vi "XW angle calib checker_fitmode_PN.vi"(0 "XW_Calib_Map file path (dialog if empty)":path=path "C:/Documents and Settings/Paul Nathan/Desktop/XW Calib Map/XW angle calib checker/XW002_OH74.txt") -> (1 "Quantities that vary with Uref (epsilon, theta, k) (higher order method)":string="Uref (m/s)\teps1 (deg)\teps2 (deg)\tProbe zero err. (deg)\ttheta 1 (deg)\ttheta 2 (deg)\tk1\tk2\r\n0.5018157894736842\t6.6267533355295267\t-2.9096917617315063\t1.8585307868990102\t-71.8440498634698343\t62.9636877172930269\t0.6599332295131558\t0.5182677319056692\r\n0.9994315789473684\t-1.5238812538482893\t0.9867720938009588\t-0.2685545800236653\t-50.7967211983630662\t49.0160971121406419\t0.4477378321660209\t0.4147363151308791\r\n2.0002052631578948\t-0.7133248964583326\t0.8757082064818568\t0.0811916550117621\t-47.4142025982968249\t46.7238739777964795\t0.3482854524979783\t0.3208003585595112\r\n3.0007842105263158\t0.1760631838109209\t0.0773496663189839\t0.1267064250649524\t-46.5210606369966584\t46.4000168794064933\t0.3180701353043149\t0.2880980466431173\r\n3.9999473684210529\t0.1906487887884849\t-0.2531251578949695\t-0.0312381845532423\t-46.1290205114913973\t46.2520699692747499\t0.2973863116337986\t0.2724916341605897\r\n4.9998315789473686\t0.2282387696125690\t-0.2130683224321257\t0.0075852235902217\t-45.8252448288331706\t46.0312176850919527\t0.2848963782809624\t0.2591128097080995\r\n6.9997315789473680\t0.1263159354503521\t-0.1724714828642592\t-0.0230777737069536\t-45.2896437061695636\t45.4966612147379905\t0.2642800771604699\t0.2410224971037088\r\n9.0019315789473691\t-0.0565462004426649\t0.0773785766074275\t0.0104161880823813\t-44.8675096760090710\t45.0959281609883007\t0.2463064031896132\t0.2236365187658775\r\n10.9999736842105253\t-0.2539290822848205\t0.4859354251419727\t0.1160031714285761\t-44.4053231675819475\t44.4986166412718589\t0.2285399354877704\t0.2028480726593352\r\n13.0001684210526314\t-0.5118579225506359\t0.7409038885633608\t0.1145229830063624\t-44.0067920576490863\t43.9637273900855589\t0.2106532081178253\t0.1851715125746720\r\n15.0011421052631579\t-0.7550503383633456\t0.9105592735667931\t0.0777544676017238\t-43.6252625738814430\t43.5843363193315980\t0.1938872474806047\t0.1681952069880479\r\n", 2 "Quantities that vary with Uref (epsilon, theta, k) (standard method)":string="Uref (m/s)\teps1 (deg)\teps2 (deg)\tProbe zero err. (deg)\ttheta 1 (deg)\ttheta 2 (deg)\r\n0.5018157894736842\t9.3017890724801830\t-6.2576200383800815\t1.5220845170500508\t-30.2854646617259924\t38.4907443143961103\r\n0.9994315789473684\t-0.5078267063761874\t0.4756008610831978\t-0.0161129226464948\t-33.2549649340571562\t37.2028076780815198\r\n2.0002052631578948\t-0.0170670287325283\t0.4389133857835795\t0.2109231785255256\t-40.3150704772274295\t40.5384275834816208\r\n3.0007842105263158\t0.5397928552976248\t-0.1673075851488837\t0.1862426350743706\t-41.7471477428440920\t42.7336376551682235\r\n3.9999473684210529\t0.5552032611501811\t-0.4809296208955749\t0.0371368201273031\t-42.3649922651800707\t43.4904856798574783\r\n4.9998315789473686\t0.5839145398374913\t-0.4879117310338565\t0.0480014044018174\t-42.5176867926462378\t43.6855272441884636\r\n6.9997315789473680\t0.4769954292660519\t-0.3766339827294708\t0.0501807232682906\t-42.6403950914849332\t43.8399700483001169\r\n9.0019315789473691\t0.2955464302508806\t-0.1481957767585597\t0.0736753267461604\t-42.6422862340712001\t43.6715341103828791\r\n10.9999736842105253\t0.0708841951620765\t0.2586334095830275\t0.1647588023725520\t-42.4997912977266665\t43.2532991548099801\r\n13.0001684210526314\t-0.2243455550085545\t0.5043620030432825\t0.1400082240173640\t-42.3214463588717393\t42.9148784991085179\r\n15.0011421052631579\t-0.4668513181945785\t0.7171710888419789\t0.1251598853237002\t-42.1380350724668275\t42.7497636859784933\r\n")   [LabVIEW 2011]
uses:
  <vilib>/Utility/file.llb/Read From Spreadsheet File (DBL).vi
  <vilib>/Utility/file.llb/Read From Spreadsheet File (string).vi
  <vilib>/Analysis/polynomials.llb/Polynomial Plot (Range).vi
  <vilib>/Analysis/polynomials.llb/Polynomial Roots (DBL).vi
  <vilib>/Analysis/polynomials.llb/Polynomial Plot (Samples).vi
  <vilib>/Analysis/NI_AALPro.lvlib
  <vilib>/Analysis/NI_AALBase.lvlib
panel:
  out "No real roots for the set (i.e. poor dataset)":bool[](array[boolean])
  in  "Transfer query set control here":bool
  in  "Query set (alias)":i32
  out "Quartic tan(2e) function":cluster{dbl[], dbl[]}[](graph)
  out "Roots for e2 (2nd index angle set -1)":cdb[][](array[numeric])=[[-1.531222514048462+0.0i, -5.778988170526063+0.0i, 16.707412903025652+0.0i, 6.4875967459+0.0i, 5.078758977720174+0.0i, 4.514924906289319+0.0i, 3.854535285382964+0.0i, 3.5396117006623293+0.0i, 3.273353030480773+0.0i, 3.048630181958499+0.0i, 2.870340574754266+0.0i], [0.0160598872047017+0.9915361243519932i, 0.030855825212726732+0.9930589066324856i, 0.0324524213798118+1.0004216780304256i, 0.03210670637546993+1.0043354071771735i, 0.03176644318451339+1.0060241435427542i, 0.0316033433674252+1.0067247444186669i, 0.0320563492832904+1.0079772109676077i, 0.032215191064157794+1.0084528128807428i, 0.032831359734918485+1.0088460213011843i, 0.03354547660184823+1.0094431819546545i, 0.03393148490012644+1.0099991970101192i], [0.0160598872047017-0.9915361243519932i, 0.030855825212726732-0.9930589066324856i, 0.0324524213798118-1.0004216780304256i, 0.03210670637546993-1.0043354071771735i, 0.03176644318451339-1.0060241435427542i, 0.0316033433674252-1.0067247444186669i, 0.0320563492832904-1.0079772109676077i, 0.032215191064157794-1.0084528128807428i, 0.032831359734918485-1.0088460213011843i, 0.03354547660184823-1.0094431819546545i, 0.03393148490012644-1.0099991970101192i], [-0.10191810443911936+0.0i, 0.03445847280570602+0.0i, 0.030577507463478096+0.0i, 0.002700019266282215+0.0i, -0.00883596479286889+0.0i, -0.007437624657217361+0.0i, -0.006020463221166026+0.0i, 0.0027010284330839292+0.0i, 0.01696397323767586+0.0i, 0.025868192292574674+0.0i, 0.03179522253597651+0.0i]]
  out "Roots for e1 (2nd index angle set- 1)":cdb[][](array[numeric])=[[-0.015920835836600963+0.9840410941913055i, 3.395480898493786+0.0i, -594.6858847660856+0.0i, -9.256262608165475+0.0i, -6.488582226964654+0.0i, -5.4418669081945525+0.0i, -4.436840208641847+0.0i, -3.919873244378892+0.0i, -3.5319472433943147+0.0i, -3.2746647104988313+0.0i, -3.0804435614198247+0.0i], [-0.015920835836600963-0.9840410941913055i, -0.02744316398189495+0.9898767262763452i, -0.03214949692082159+0.9987358189508451i, -0.033633194220895994+1.0032718682899568i, -0.0335171638363392+1.0048208292329712i, -0.03365083549489199+1.005877792371468i, -0.03393002543702201+1.007203137493328i, -0.03407557298898485+1.0080087857191544i, -0.034416949826886645+1.0087849149152948i, -0.03463560472159085+1.0092611917473095i, -0.03494277753284671+1.009676498285988i], [0.6282192557965216+0.0i, -0.02744316398189495-0.9898767262763452i, -0.03214949692082159-0.9987358189508451i, -0.033633194220895994-1.0032718682899568i, -0.0335171638363392-1.0048208292329712i, -0.03365083549489199-1.005877792371468i, -0.03393002543702201-1.007203137493328i, -0.03407557298898485-1.0080087857191544i, -0.034416949826886645-1.0087849149152948i, -0.03463560472159085-1.0092611917473095i, -0.03494277753284671-1.009676498285988i], [0.23553334080037738+0.0i, -0.053243718596295814+0.0i, -0.024904883355210836+0.0i, 0.006145841875296154+0.0i, 0.0066549964036471156+0.0i, 0.00796720459081318+0.0i, 0.004409286517190577+0.0i, -0.0019738373178073043+0.0i, -0.008864029245855196+0.0i, -0.017869113637998108+0.0i, -0.026362333333484183+0.0i]]
  in  "Coefficient Constraint":cluster{"order":i32, "coefficient":dbl}[](array[cluster])
  in  "Ignore first n pts from calib.":i32
  out "Higher order effective angle method X plot data (each angle set separated by a column of zeros)":string="x_0\ty1_0\ty2_0\t\tx_1\ty1_1\ty2_1\t\tx_2\ty1_2\ty2_2\t\tx_3\ty1_3\ty2_3\t\tx_4\ty1_4\ty2_4\t\tx_5\ty1_5\ty2_5\t\tx_6\ty1_6\ty2_6\t\tx_7\ty1_7\ty2_7\t\tx_8\ty1_8\ty2_8\t\tx_9\ty1_9\ty2_9\t\tx_10\ty1_10\ty2_10\r\n-0.9999999999999999\t-0.9085791502544248\t-3.9630468181290452\t0.0000000000000000\t-0.9999999999999999\t0.1949143754370715\t-2.6536651485735696\t0.0000000000000000\t-0.9999999999999999\t0.5188418104065096\t-2.7107465604685741\t0.0000000000000000\t-0.9999999999999999\t0.6105115215521106\t-2.7972176259688553\t0.0000000000000000\t-0.9999999999999999\t0.6514204222508733\t-2.8375050105836368\t0.0000000000000000\t-0.9999999999999999\t0.6746558655695405\t-2.8404947938821206\t0.0000000000000000\t-0.9999999999999999\t0.7084619405900626\t-2.8035914112508933\t0.0000000000000000\t-0.9999999999999999\t0.7363342408659557\t-2.7810177224561561\t0.0000000000000000\t-0.9999999999999999\t0.7620888951136892\t-2.7288520875385447\t0.0000000000000000\t-0.9999999999999999\t0.7861588927941786\t-2.6856742001602751\t0.0000000000000000\t-0.9999999999999999\t0.8056811585366324\t-2.6550478856042679\t0.0000000000000000\r\n-0.8459634362504808\t-0.4625621144061756\t-2.8818271450789865\t0.0000000000000000\t-0.8459634362504808\t0.2815754544138509\t-2.1394999422469003\t0.0000000000000000\t-0.8459634362504808\t0.5527709767869218\t-2.2324745574527904\t0.0000000000000000\t-0.8459634362504808\t0.6382823976284421\t-2.2665818845631214\t0.0000000000000000\t-0.8459634362504808\t0.6788684735006610\t-2.2842367882197863\t0.0000000000000000\t-0.8459634362504808\t0.7029454921629841\t-2.2878897351586707\t0.0000000000000000\t-0.8459634362504808\t0.7360252511014151\t-2.2626966309367886\t0.0000000000000000\t-0.8459634362504808\t0.7617351722175852\t-2.2416920469763459\t0.0000000000000000\t-0.8432720672116305\t0.7844643868612465\t-2.1887614629441035\t0.0000000000000000\t-0.8432720672116305\t0.8038053956321515\t-2.1508294307461551\t0.0000000000000000\t-0.8432720672116305\t0.8196056618936665\t-2.1284563267855230\t0.0000000000000000\r\n-0.7028117712403573\t-0.0667229984385117\t-1.7990557676966663\t0.0000000000000000\t-0.7028117712403573\t0.3411211378733948\t-1.6837865113002857\t0.0000000000000000\t-0.7028117712403573\t0.5825100736406964\t-1.6930687846557417\t0.0000000000000000\t-0.7028117712403573\t0.6448979960495834\t-1.7825502259833412\t0.0000000000000000\t-0.7028117712403573\t0.6810359033183786\t-1.8105052193118192\t0.0000000000000000\t-0.7028117712403573\t0.7040869499204692\t-1.8110590099219335\t0.0000000000000000\t-0.7028117712403573\t0.7342043939074193\t-1.7929291162742504\t0.0000000000000000\t-0.7028117712403573\t0.7550109725157748\t-1.7756905349598751\t0.0000000000000000\t-0.7028117712403573\t0.7711095218508195\t-1.7384235052178580\t0.0000000000000000\t-0.7028117712403573\t0.7847492951756501\t-1.7045648544699419\t0.0000000000000000\t-0.7028117712403573\t0.7958199433613861\t-1.6859867806778905\t0.0000000000000000\r\n-0.5745611109571804\t-0.0376287976903837\t-1.5446740531776548\t0.0000000000000000\t-0.5745611109571804\t0.3599220910286302\t-1.3459064192482468\t0.0000000000000000\t-0.5745611109571804\t0.5655852803690335\t-1.3559695335879334\t0.0000000000000000\t-0.5745611109571804\t0.6247863747603235\t-1.3916622950809854\t0.0000000000000000\t-0.5745611109571804\t0.6553574621762963\t-1.4097043857813083\t0.0000000000000000\t-0.5745611109571804\t0.6735069299277736\t-1.4112094707533349\t0.0000000000000000\t-0.5745611109571804\t0.6949413208702192\t-1.4067266943759922\t0.0000000000000000\t-0.5745611109571804\t0.7105513693367174\t-1.3847598236387422\t0.0000000000000000\t-0.5745611109571804\t0.7218957685787146\t-1.3544132560361197\t0.0000000000000000\t-0.5766523484064272\t0.7309919560241551\t-1.3305928734680903\t0.0000000000000000\t-0.5745611109571804\t0.7384817158571489\t-1.3099108075871668\t0.0000000000000000\r\n-0.4610063144273182\t0.0412919475631363\t-1.0997890950007321\t0.0000000000000000\t-0.4610063144273182\t0.3770239497989202\t-0.9792680032688384\t0.0000000000000000\t-0.4610063144273182\t0.5367013693167687\t-1.0119826258435312\t0.0000000000000000\t-0.4610063144273182\t0.5743830527285835\t-1.0774202158722981\t0.0000000000000000\t-0.4610063144273182\t0.5979952814046342\t-1.0939710197186976\t0.0000000000000000\t-0.4667326950738877\t0.6116296380054032\t-1.0948501153158237\t0.0000000000000000\t-0.4610063144273182\t0.6279311798252735\t-1.0827733496154128\t0.0000000000000000\t-0.4610063144273182\t0.6377056286721594\t-1.0683619324969325\t0.0000000000000000\t-0.4610063144273182\t0.6452821120555695\t-1.0398621565011508\t0.0000000000000000\t-0.4629123289077153\t0.6520868780188794\t-1.0198362226727229\t0.0000000000000000\t-0.4629123289077153\t0.6571442461528323\t-1.0051143364341999\t0.0000000000000000\r\n-0.3689194771098271\t0.1044333744574640\t-0.7437632758411701\t0.0000000000000000\t-0.3689194771098271\t0.3703284183929321\t-0.7061988569542564\t0.0000000000000000\t-0.3689194771098271\t0.4814947359213608\t-0.7770192864712264\t0.0000000000000000\t-0.3689194771098271\t0.5088608177696153\t-0.8210529776089235\t0.0000000000000000\t-0.3635749763519443\t0.5263421036228286\t-0.8282138902172458\t0.0000000000000000\t-0.3689194771098271\t0.5331564790478260\t-0.8458290235908140\t0.0000000000000000\t-0.3689194771098271\t0.5437170073266897\t-0.8393399765706897\t0.0000000000000000\t-0.3689194771098271\t0.5501602814743358\t-0.8249109991926368\t0.0000000000000000\t-0.3689194771098271\t0.5563221043460842\t-0.7999971908211336\t0.0000000000000000\t-0.3689194771098271\t0.5623927525763176\t-0.7803547186651004\t0.0000000000000000\t-0.3689194771098271\t0.5671583051208874\t-0.7700855374663110\t0.0000000000000000\r\n-0.2718814121476857\t0.0255847727338301\t-0.6689751955611348\t0.0000000000000000\t-0.2718814121476857\t0.3106644522796246\t-0.5047454592362141\t0.0000000000000000\t-0.2718814121476857\t0.3962036651655259\t-0.5446172063124690\t0.0000000000000000\t-0.2718814121476857\t0.4082234758439587\t-0.5916721671054449\t0.0000000000000000\t-0.2718814121476857\t0.4191107855801626\t-0.5983889263646065\t0.0000000000000000\t-0.2718814121476857\t0.4242807676181213\t-0.6036578351430176\t0.0000000000000000\t-0.2718814121476857\t0.4289132363159743\t-0.6011772566633612\t0.0000000000000000\t-0.2718814121476857\t0.4344930216745795\t-0.5885638990500427\t0.0000000000000000\t-0.2718814121476857\t0.4407940406478280\t-0.5667386082032163\t0.0000000000000000\t-0.2718814121476857\t0.4466625036118104\t-0.5511317529698531\t0.0000000000000000\t-0.2718814121476857\t0.4513779468028263\t-0.5395864188016505\t0.0000000000000000\r\n-0.1761470268806888\t-0.0942490676366393\t-0.5868960272983509\t0.0000000000000000\t-0.1761470268806888\t0.2548185009347063\t-0.2645492620955306\t0.0000000000000000\t-0.1761470268806888\t0.3024751991218511\t-0.2921952683619167\t0.0000000000000000\t-0.1761470268806888\t0.2870434875402270\t-0.3500127136267793\t0.0000000000000000\t-0.1761470268806888\t0.2830095550319655\t-0.3828463334548899\t0.0000000000000000\t-0.1761470268806888\t0.2855455723517732\t-0.3809026465127626\t0.0000000000000000\t-0.1761470268806888\t0.2884644985637423\t-0.3799013981302747\t0.0000000000000000\t-0.1761470268806888\t0.2930495918311506\t-0.3699160983941475\t0.0000000000000000\t-0.1761470268806888\t0.2992247712103860\t-0.3541806551714389\t0.0000000000000000\t-0.1761470268806888\t0.3058374237252131\t-0.3408777024657876\t0.0000000000000000\t-0.1761470268806888\t0.3111246627753121\t-0.3320591164269514\t0.0000000000000000\r\n-0.0850270210113130\t-0.0504595050252811\t-0.2775995341357290\t0.0000000000000000\t-0.0850270210113130\t0.1736177181817981\t-0.0758426654882593\t0.0000000000000000\t-0.0850270210113130\t0.1727751104131255\t-0.1124460755508965\t0.0000000000000000\t-0.0850270210113130\t0.1397558723489909\t-0.1611761582181669\t0.0000000000000000\t-0.0850270210113130\t0.1364092384545839\t-0.1803971782800010\t0.0000000000000000\t-0.0850270210113130\t0.1330151029088564\t-0.1846382073328683\t0.0000000000000000\t-0.0850270210113130\t0.1336180079889946\t-0.1859543864792222\t0.0000000000000000\t-0.0850270210113130\t0.1391330147914122\t-0.1779026144672113\t0.0000000000000000\t-0.0881921819968595\t0.1468097530657032\t-0.1664128928822258\t0.0000000000000000\t-0.0850270210113130\t0.1533034947310865\t-0.1537657502004380\t0.0000000000000000\t-0.0850270210113130\t0.1602920927213465\t-0.1466312867329973\t0.0000000000000000\r\n0.0000000000000000\t-0.1396755488429087\t-0.1495552894031837\t0.0000000000000000\t0.0000000000000000\t0.1015398030851381\t0.0979907823209607\t0.0000000000000000\t0.0000000000000000\t0.0485713499475330\t0.0551796899852733\t0.0000000000000000\t0.0000000000000000\t0.0039204586603697\t0.0100793521533393\t0.0000000000000000\t0.0000000000000000\t-0.0123772694902811\t-0.0123048930616856\t0.0000000000000000\t0.0000000000000000\t-0.0158825708767742\t-0.0172400662126269\t0.0000000000000000\t0.0000000000000000\t-0.0185621834928470\t-0.0203971278636718\t0.0000000000000000\t0.0000000000000000\t-0.0117122957217886\t-0.0145134805930901\t0.0000000000000000\t-0.0015707976187244\t-0.0034205951378717\t-0.0026021495757281\t0.0000000000000000\t0.0000000000000000\t0.0051491403774043\t0.0063664317326143\t0.0000000000000000\t0.0000000000000000\t0.0119067452638700\t0.0115332438693104\t0.0000000000000000\r\n0.0834450784477064\t-0.0417648215636864\t0.1352429486294378\t0.0000000000000000\t0.0834450784477064\t-0.0776394529995262\t0.1668355133205353\t0.0000000000000000\t0.0834450784477064\t-0.1147770314630093\t0.1823015191280195\t0.0000000000000000\t0.0834450784477064\t-0.1518089738821856\t0.1616926063828080\t0.0000000000000000\t0.0834450784477064\t-0.1675177345562901\t0.1418323488914914\t0.0000000000000000\t0.0834450784477064\t-0.1743808906051748\t0.1396223268122237\t0.0000000000000000\t0.0834450784477064\t-0.1748799907332232\t0.1407817659046222\t0.0000000000000000\t0.0834450784477064\t-0.1711359562908112\t0.1443459528715696\t0.0000000000000000\t0.0834450784477064\t-0.1631451101745820\t0.1538692306045876\t0.0000000000000000\t0.0834450784477064\t-0.1562961885310737\t0.1594290597441742\t0.0000000000000000\t0.0834450784477064\t-0.1463689695846851\t0.1660732505077365\t0.0000000000000000\r\n0.1745279388943651\t-0.2504441955126037\t0.1552207836757285\t0.0000000000000000\t0.1745279388943651\t-0.1923048605897919\t0.3015431454828965\t0.0000000000000000\t0.1745279388943651\t-0.3118645832700102\t0.3060446247312193\t0.0000000000000000\t0.1745279388943651\t-0.3399045763763606\t0.3042221403451356\t0.0000000000000000\t0.1745279388943651\t-0.3591535093836093\t0.2969861016671120\t0.0000000000000000\t0.1745279388943651\t-0.3625352124879301\t0.2987758625039919\t0.0000000000000000\t0.1745279388943651\t-0.3625811847622155\t0.2987619180587648\t0.0000000000000000\t0.1761470268806888\t-0.3586700905175086\t0.3043173930134577\t0.0000000000000000\t0.1745279388943651\t-0.3487858594270737\t0.3125226906016907\t0.0000000000000000\t0.1745279388943651\t-0.3381938626612139\t0.3167839456066439\t0.0000000000000000\t0.1745279388943651\t-0.3288971373969858\t0.3213424951515983\t0.0000000000000000\r\n0.2701952220731489\t-0.4823610385730527\t0.1684170210190646\t0.0000000000000000\t0.2701952220731489\t-0.3941480974967655\t0.3747405534620119\t0.0000000000000000\t0.2685104627037557\t-0.5123196133813664\t0.4244954643928500\t0.0000000000000000\t0.2685104627037557\t-0.5622716481313378\t0.4320516895393265\t0.0000000000000000\t0.2685104627037557\t-0.5746725215951116\t0.4333475328171350\t0.0000000000000000\t0.2701952220731489\t-0.5761161656795665\t0.4382762721402697\t0.0000000000000000\t0.2701952220731489\t-0.5711564795303717\t0.4462115429854009\t0.0000000000000000\t0.2685104627037557\t-0.5637027508394487\t0.4500064910221563\t0.0000000000000000\t0.2685104627037557\t-0.5531821206069903\t0.4562858049551752\t0.0000000000000000\t0.2685104627037557\t-0.5410697161194152\t0.4598006047578997\t0.0000000000000000\t0.2685104627037557\t-0.5305871950835828\t0.4640535298803268\t0.0000000000000000\r\n0.3635749763519443\t-0.6862363241063577\t0.1938745671240703\t0.0000000000000000\t0.3671359250169842\t-0.6594497435504401\t0.4155995678888906\t0.0000000000000000\t0.3689194771098271\t-0.8062252804138840\t0.4942666230060676\t0.0000000000000000\t0.3671359250169842\t-0.8150435379645339\t0.5333980586374278\t0.0000000000000000\t0.3671359250169842\t-0.8025341705196405\t0.5488805679771741\t0.0000000000000000\t0.3689194771098271\t-0.8130451171136217\t0.5564687631683539\t0.0000000000000000\t0.3671359250169842\t-0.8041120781889549\t0.5656961795372176\t0.0000000000000000\t0.3671359250169842\t-0.7982752853845158\t0.5727446882583248\t0.0000000000000000\t0.3671359250169842\t-0.7840331881102651\t0.5783268868158106\t0.0000000000000000\t0.3671359250169842\t-0.7703712073294504\t0.5816443488942544\t0.0000000000000000\t0.3671359250169842\t-0.7586054072639649\t0.5859279656615510\t0.0000000000000000\r\n0.4629123289077153\t-0.8476294329786266\t0.2235614092068809\t0.0000000000000000\t0.4629123289077153\t-0.9492224197361369\t0.4327728553093401\t0.0000000000000000\t0.4610063144273182\t-0.9819378661710078\t0.5718021480660419\t0.0000000000000000\t0.4610063144273182\t-1.0553848834240576\t0.6055334918430288\t0.0000000000000000\t0.4610063144273182\t-1.0574404797332702\t0.6253666996480907\t0.0000000000000000\t0.4610063144273182\t-1.0556690478955482\t0.6393228823720644\t0.0000000000000000\t0.4610063144273182\t-1.0477195054982680\t0.6529818956214503\t0.0000000000000000\t0.4610063144273182\t-1.0344062288018556\t0.6626927832176096\t0.0000000000000000\t0.4610063144273182\t-1.0205105865152524\t0.6697752152893657\t0.0000000000000000\t0.4610063144273182\t-1.0056840847353361\t0.6738862961883090\t0.0000000000000000\t0.4667326950738877\t-0.9992094770597746\t0.6782936840236679\t0.0000000000000000\r\n0.5724736448682121\t-1.3899789264513560\t0.1020641173846400\t0.0000000000000000\t0.5724736448682121\t-1.2323317956367625\t0.4538004753460074\t0.0000000000000000\t0.5724736448682121\t-1.3238555928281337\t0.6021700169460663\t0.0000000000000000\t0.5724736448682121\t-1.3635980664653848\t0.6589555940191650\t0.0000000000000000\t0.5724736448682121\t-1.3598145734442184\t0.6847037690811968\t0.0000000000000000\t0.5724736448682121\t-1.3684754908238803\t0.7014719043851134\t0.0000000000000000\t0.5724736448682121\t-1.3561242322873066\t0.7226084437915833\t0.0000000000000000\t0.5724736448682121\t-1.3414409891263650\t0.7365615404721209\t0.0000000000000000\t0.5703899296732948\t-1.3202033688759527\t0.7473204528114626\t0.0000000000000000\t0.5703899296732948\t-1.3047561674071091\t0.7540053749349491\t0.0000000000000000\t0.5703899296732948\t-1.2856457129099557\t0.7602089334598410\t0.0000000000000000\r\n0.7004676747806673\t-2.2697364417842891\t-0.1308275547072091\t0.0000000000000000\t0.7004676747806673\t-1.6322660285466430\t0.4389604957859697\t0.0000000000000000\t0.7004676747806673\t-1.7125591635376343\t0.6186366367406101\t0.0000000000000000\t0.7004676747806673\t-1.7507849758841230\t0.6833036449657283\t0.0000000000000000\t0.7004676747806673\t-1.7532033361976842\t0.7149717797808454\t0.0000000000000000\t0.7004676747806673\t-1.7468810658722469\t0.7363863563633494\t0.0000000000000000\t0.6981287310371237\t-1.7323516588972048\t0.7628805858487009\t0.0000000000000000\t0.7004676747806673\t-1.7225575014273988\t0.7821105315579404\t0.0000000000000000\t0.6981287310371237\t-1.6962155420747351\t0.7969917434866054\t0.0000000000000000\t0.6981287310371237\t-1.6783350413415989\t0.8084591863151523\t0.0000000000000000\t0.6981287310371237\t-1.6580717599172035\t0.8184445444178572\t0.0000000000000000\r\n0.8432720672116305\t-2.2413583286537802\t-0.0361829804629510\t0.0000000000000000\t0.8432720672116305\t-2.3075415725227733\t0.3599602272717538\t0.0000000000000000\t0.8432720672116305\t-2.1691060617855422\t0.6115535237817370\t0.0000000000000000\t0.8432720672116305\t-2.2290412862152995\t0.6830463271258672\t0.0000000000000000\t0.8432720672116305\t-2.2222009266918268\t0.7182124425293464\t0.0000000000000000\t0.8379106495048978\t-2.2019648631264235\t0.7421134752332942\t0.0000000000000000\t0.8432720672116305\t-2.1971863462195551\t0.7681137807799585\t0.0000000000000000\t0.8432720672116305\t-2.1821977941933697\t0.7910287339996136\t0.0000000000000000\t0.8432720672116305\t-2.1597258190303488\t0.8104743841359477\t0.0000000000000000\t0.8432720672116305\t-2.1347740356153819\t0.8264250196496778\t0.0000000000000000\t0.8432720672116305\t-2.1122974634158354\t0.8411438740059636\t0.0000000000000000\r\n0.9999999999999999\t-2.8237734406173329\t-0.1791722171870904\t0.0000000000000000\t0.9999999999999999\t-2.6217506945340499\t0.3404580267525550\t0.0000000000000000\t0.9999999999999999\t-2.7652216719375038\t0.5776183997010226\t0.0000000000000000\t0.9999999999999999\t-2.7434622913910154\t0.6673214592086288\t0.0000000000000000\t0.9999999999999999\t-2.7691832771154199\t0.7016501297022305\t0.0000000000000000\t0.9999999999999999\t-2.7634005636598853\t0.7220453961815417\t0.0000000000000000\t0.9999999999999999\t-2.7441674751271026\t0.7453072103707526\t0.0000000000000000\t0.9999999999999999\t-2.7255665231484856\t0.7665049857410070\t0.0000000000000000\t0.9999999999999999\t-2.6957943045968502\t0.7883146132106904\t0.0000000000000000\t0.9999999999999999\t-2.6708083003892944\t0.8079886891481993\t0.0000000000000000\t0.9999999999999999\t-2.6439319990345118\t0.8268920789495620\t0.0000000000000000\r\n"
  out "Standard effective angle method X plot data (each angle set separated by a column of zeros)":string="x_0\ty1_0\ty2_0\t\tx_1\ty1_1\ty2_1\t\tx_2\ty1_2\ty2_2\t\tx_3\ty1_3\ty2_3\t\tx_4\ty1_4\ty2_4\t\tx_5\ty1_5\ty2_5\t\tx_6\ty1_6\ty2_6\t\tx_7\ty1_7\ty2_7\t\tx_8\ty1_8\ty2_8\t\tx_9\ty1_9\ty2_9\t\tx_10\ty1_10\ty2_10\r\n-0.9999999999999999\t-0.3815133550763904\t-1.2277896709808682\t0.0000000000000000\t-0.9999999999999999\t0.1027343623190909\t-0.9114562899981703\t0.0000000000000000\t-0.9999999999999999\t0.3063443292284778\t-0.9263298161188739\t0.0000000000000000\t-0.9999999999999999\t0.3759098795463195\t-0.9486450743962725\t0.0000000000000000\t-0.9999999999999999\t0.4095937180643089\t-0.9589550813083074\t0.0000000000000000\t-0.9999999999999999\t0.4296105414451811\t-0.9597180393827375\t0.0000000000000000\t-0.9999999999999999\t0.4600573554441755\t-0.9502798289606784\t0.0000000000000000\t-0.9999999999999999\t0.4865160575694266\t-0.9444839218816277\t0.0000000000000000\t-0.9999999999999999\t0.5122386804119141\t-0.9310235854433639\t0.0000000000000000\t-0.9999999999999999\t0.5375704300049343\t-0.9198109803207908\t0.0000000000000000\t-0.9999999999999999\t0.5591838915563910\t-0.9118179530499936\t0.0000000000000000\r\n-0.8459634362504808\t-0.2093643431183902\t-0.9702353019573543\t0.0000000000000000\t-0.8459634362504808\t0.1524007163841222\t-0.7718634095908468\t0.0000000000000000\t-0.8459634362504808\t0.3312481602170517\t-0.7979083840543126\t0.0000000000000000\t-0.8459634362504808\t0.3985703678969933\t-0.8073687738154385\t0.0000000000000000\t-0.8459634362504808\t0.4333153200417899\t-0.8122463376207405\t0.0000000000000000\t-0.8459634362504808\t0.4549729292622101\t-0.8132539080775948\t0.0000000000000000\t-0.8459634362504808\t0.4862152698857382\t-0.8062936170337284\t0.0000000000000000\t-0.8459634362504808\t0.5118762167416807\t-0.8004699517004846\t0.0000000000000000\t-0.8432720672116305\t0.5357418679885581\t-0.7857103524771601\t0.0000000000000000\t-0.8432720672116305\t0.5570613988735588\t-0.7750575851915775\t0.0000000000000000\t-0.8432720672116305\t0.5752714536243961\t-0.7687442796474347\t0.0000000000000000\r\n-0.7028117712403573\t-0.0328228301303722\t-0.6730378859119317\t0.0000000000000000\t-0.7028117712403573\t0.1882864654777492\t-0.6382266361222080\t0.0000000000000000\t-0.7028117712403573\t0.3538653960982250\t-0.6410572155338587\t0.0000000000000000\t-0.7028117712403573\t0.4040956419437625\t-0.6680977866969731\t0.0000000000000000\t-0.7028117712403573\t0.4352309350879587\t-0.6764561489379372\t0.0000000000000000\t-0.7028117712403573\t0.4560210940858728\t-0.6766213078456130\t0.0000000000000000\t-0.7028117712403573\t0.4844463111444350\t-0.6712058868596205\t0.0000000000000000\t-0.7028117712403573\t0.5050363372082499\t-0.6660403761493522\t0.0000000000000000\t-0.7028117712403573\t0.5215750025874688\t-0.6548182695443805\t0.0000000000000000\t-0.7028117712403573\t0.5360488120239911\t-0.6445561268834644\t0.0000000000000000\t-0.7028117712403573\t0.5481371262887226\t-0.6388980385240232\t0.0000000000000000\r\n-0.5745611109571804\t-0.0186406617106857\t-0.5952034519702041\t0.0000000000000000\t-0.5745611109571804\t0.1999513083746903\t-0.5316352108933271\t0.0000000000000000\t-0.5745611109571804\t0.3408985513360128\t-0.5349167839293223\t0.0000000000000000\t-0.5745611109571804\t0.3874531648602888\t-0.5465000145751649\t0.0000000000000000\t-0.5745611109571804\t0.4129373646503266\t-0.5523222557772299\t0.0000000000000000\t-0.5745611109571804\t0.4286042789167682\t-0.5528069650646648\t0.0000000000000000\t-0.5745611109571804\t0.4476788261076887\t-0.5513628506497092\t0.0000000000000000\t-0.5745611109571804\t0.4619956964268012\t-0.5442667592222343\t0.0000000000000000\t-0.5745611109571804\t0.4726441131254100\t-0.5344097418995096\t0.0000000000000000\t-0.5766523484064272\t0.4813401461691441\t-0.5266279420566395\t0.0000000000000000\t-0.5745611109571804\t0.4886114157092954\t-0.5198390729242247\t0.0000000000000000\r\n-0.4610063144273182\t0.0208636190821711\t-0.4490649036536395\t0.0000000000000000\t-0.4610063144273182\t0.2107116811955977\t-0.4068646001903803\t0.0000000000000000\t-0.4610063144273182\t0.3193395628632208\t-0.4184437337601838\t0.0000000000000000\t-0.4610063144273182\t0.3476067541187934\t-0.4413258534669730\t0.0000000000000000\t-0.4610063144273182\t0.3659615795589626\t-0.4470559836159407\t0.0000000000000000\t-0.4667326950738877\t0.3768063206397253\t-0.4473597048819011\t0.0000000000000000\t-0.4610063144273182\t0.3900255577692402\t-0.4431816758867931\t0.0000000000000000\t-0.4610063144273182\t0.3980910606014888\t-0.4381800765192558\t0.0000000000000000\t-0.4610063144273182\t0.4044180258399097\t-0.4282374300168551\t0.0000000000000000\t-0.4629123289077153\t0.4101583924636033\t-0.4212094225246056\t0.0000000000000000\t-0.4629123289077153\t0.4144611423251504\t-0.4160205988735473\t0.0000000000000000\r\n-0.3689194771098271\t0.0536561800579369\t-0.3205162913955928\t0.0000000000000000\t-0.3689194771098271\t0.2064815177911305\t-0.3062154711050765\t0.0000000000000000\t-0.3689194771098271\t0.2799269036558585\t-0.3330488687483389\t0.0000000000000000\t-0.3689194771098271\t0.2991867707938265\t-0.3494639593590201\t0.0000000000000000\t-0.3635749763519443\t0.3117719154399675\t-0.3521145995133866\t0.0000000000000000\t-0.3689194771098271\t0.3167405171150758\t-0.3586129042485994\t0.0000000000000000\t-0.3689194771098271\t0.3245127738637020\t-0.3562226869399766\t0.0000000000000000\t-0.3689194771098271\t0.3292990841472899\t-0.3508926675323383\t0.0000000000000000\t-0.3689194771098271\t0.3339084930327397\t-0.3416397395803143\t0.0000000000000000\t-0.3689194771098271\t0.3384811057696974\t-0.3342993362304802\t0.0000000000000000\t-0.3689194771098271\t0.3420929435861684\t-0.3304456161250302\t0.0000000000000000\r\n-0.2718814121476857\t0.0128752726903403\t-0.2918882287416100\t0.0000000000000000\t-0.2718814121476857\t0.1697376633133504\t-0.2266806671812408\t0.0000000000000000\t-0.2718814121476857\t0.2229566711987844\t-0.2428262977232454\t0.0000000000000000\t-0.2718814121476857\t0.2307298756899231\t-0.2616149044401169\t0.0000000000000000\t-0.2718814121476857\t0.2378391151339257\t-0.2642740709057536\t0.0000000000000000\t-0.2718814121476857\t0.2412383560156202\t-0.2663561249281411\t0.0000000000000000\t-0.2718814121476857\t0.2442971723726146\t-0.2653763300549608\t0.0000000000000000\t-0.2718814121476857\t0.2479980197330459\t-0.2603824415827295\t0.0000000000000000\t-0.2718814121476857\t0.2521992515701980\t-0.2516942950270311\t0.0000000000000000\t-0.2718814121476857\t0.2561334149269846\t-0.2454443997906341\t0.0000000000000000\t-0.2718814121476857\t0.2593097454420143\t-0.2408007167960739\t0.0000000000000000\r\n-0.1761470268806888\t-0.0460636059230048\t-0.2597206147786703\t0.0000000000000000\t-0.1761470268806888\t0.1367610417356654\t-0.1245217926281068\t0.0000000000000000\t-0.1761470268806888\t0.1648204978101121\t-0.1367476713685922\t0.0000000000000000\t-0.1761470268806888\t0.1556324778511593\t-0.1619004749232093\t0.0000000000000000\t-0.1761470268806888\t0.1532471169414098\t-0.1759448683738918\t0.0000000000000000\t-0.1761470268806888\t0.1547459389933540\t-0.1751181415129130\t0.0000000000000000\t-0.1761470268806888\t0.1564743623124086\t-0.1746920439546165\t0.0000000000000000\t-0.1761470268806888\t0.1591965698399837\t-0.1704341495334744\t0.0000000000000000\t-0.1761470268806888\t0.1628768138501873\t-0.1636926807243563\t0.0000000000000000\t-0.1761470268806888\t0.1668358047330725\t-0.1579627379435780\t0.0000000000000000\t-0.1761470268806888\t0.1700148572265357\t-0.1541486543885721\t0.0000000000000000\r\n-0.0850270210113130\t-0.0249192675646609\t-0.1303094859974098\t0.0000000000000000\t-0.0850270210113130\t0.0909442911360152\t-0.0372283574450995\t0.0000000000000000\t-0.0850270210113130\t0.0904809569960206\t-0.0547255925362277\t0.0000000000000000\t-0.0850270210113130\t0.0725065349820468\t-0.0775788408363293\t0.0000000000000000\t-0.0850270210113130\t0.0707041582222505\t-0.0864608498606846\t0.0000000000000000\t-0.0850270210113130\t0.0688797622803253\t-0.0884108632923820\t0.0000000000000000\t-0.0850270210113130\t0.0692035711225545\t-0.0890153288541087\t0.0000000000000000\t-0.0850270210113130\t0.0721708211052060\t-0.0853122198092176\t0.0000000000000000\t-0.0881921819968595\t0.0763170203287837\t-0.0800059689104619\t0.0000000000000000\t-0.0850270210113130\t0.0798388699423815\t-0.0741348845468330\t0.0000000000000000\t-0.0850270210113130\t0.0836442245073950\t-0.0708087068813914\t0.0000000000000000\r\n0.0000000000000000\t-0.0675558762158115\t-0.0721731620420199\t0.0000000000000000\t0.0000000000000000\t0.0521285968471978\t0.0502583416112362\t0.0000000000000000\t0.0000000000000000\t0.0245879588335671\t0.0279813221883405\t0.0000000000000000\t0.0000000000000000\t0.0019621543550413\t0.0050524396498774\t0.0000000000000000\t0.0000000000000000\t-0.0061696027461181\t-0.0061336357868599\t0.0000000000000000\t0.0000000000000000\t-0.0079100013774912\t-0.0085831974669353\t0.0000000000000000\t0.0000000000000000\t-0.0092384175668538\t-0.0101470822923124\t0.0000000000000000\t0.0000000000000000\t-0.0058391003146520\t-0.0072305995118944\t0.0000000000000000\t-0.0015707976187244\t-0.0017088375061246\t-0.0013002294895013\t0.0000000000000000\t0.0000000000000000\t0.0025778929547452\t0.0031882984899375\t0.0000000000000000\t0.0000000000000000\t0.0059712002481367\t0.0057833454771090\t0.0000000000000000\r\n0.0834450784477064\t-0.0206688109096341\t0.0700768572776769\t0.0000000000000000\t0.0834450784477064\t-0.0380941445743377\t0.0872215566308192\t0.0000000000000000\t0.0834450784477064\t-0.0558300201561846\t0.0957331804870974\t0.0000000000000000\t0.0834450784477064\t-0.0732236364720010\t0.0844087191234334\t0.0000000000000000\t0.0834450784477064\t-0.0805173457914918\t0.0736266135577358\t0.0000000000000000\t0.0834450784477064\t-0.0836885579377382\t0.0724345450655375\t0.0000000000000000\t0.0834450784477064\t-0.0839188118734830\t0.0730597462104811\t0.0000000000000000\t0.0834450784477064\t-0.0821903512279210\t0.0749842989827523\t0.0000000000000000\t0.0834450784477064\t-0.0784920538300603\t0.0801463326183820\t0.0000000000000000\t0.0834450784477064\t-0.0753121353965432\t0.0831734404720674\t0.0000000000000000\t0.0834450784477064\t-0.0706862143432525\t0.0868041012508523\t0.0000000000000000\r\n0.1745279388943651\t-0.1182326213774142\t0.0808812827908076\t0.0000000000000000\t0.1745279388943651\t-0.0919271315384520\t0.1642626880908670\t0.0000000000000000\t0.1745279388943651\t-0.1453665715699975\t0.1669601598550158\t0.0000000000000000\t0.1745279388943651\t-0.1575424728174603\t0.1658670012193113\t0.0000000000000000\t0.1745279388943651\t-0.1658273926201979\t0.1615407592894643\t0.0000000000000000\t0.1745279388943651\t-0.1672768362680423\t0.1626087309411399\t0.0000000000000000\t0.1745279388943651\t-0.1672965282061860\t0.1626004048596422\t0.0000000000000000\t0.1761470268806888\t-0.1656200455197691\t0.1659240999845745\t0.0000000000000000\t0.1745279388943651\t-0.1613724034206572\t0.1708574854717018\t0.0000000000000000\t0.1745279388943651\t-0.1568032947140209\t0.1734311556843217\t0.0000000000000000\t0.1745279388943651\t-0.1527780087237028\t0.1761932842903005\t0.0000000000000000\r\n0.2701952220731489\t-0.2175225002327688\t0.0880882833404676\t0.0000000000000000\t0.2701952220731489\t-0.1807404869389231\t0.2092665135850209\t0.0000000000000000\t0.2685104627037557\t-0.2297640478487596\t0.2413798476133460\t0.0000000000000000\t0.2685104627037557\t-0.2499086559150384\t0.2463765459722784\t0.0000000000000000\t0.2685104627037557\t-0.2548595624989720\t0.2472367788056693\t0.0000000000000000\t0.2701952220731489\t-0.2554346520944715\t0.2505176934311722\t0.0000000000000000\t0.2701952220731489\t-0.2534578092342684\t0.2558303573682952\t0.0000000000000000\t0.2685104627037557\t-0.2504810077883826\t0.2583845275495908\t0.0000000000000000\t0.2685104627037557\t-0.2462672749482715\t0.2626302182454011\t0.0000000000000000\t0.2685104627037557\t-0.2413982906865207\t0.2650174184090481\t0.0000000000000000\t0.2685104627037557\t-0.2371690244601109\t0.2679163503262259\t0.0000000000000000\r\n0.3635749763519443\t-0.2985516255068020\t0.1021551175866013\t0.0000000000000000\t0.3671359250169842\t-0.2881963140571548\t0.2355391232305545\t0.0000000000000000\t0.3689194771098271\t-0.3439588090465734\t0.2888506647729097\t0.0000000000000000\t0.3671359250169842\t-0.3472355168880212\t0.3169173246505426\t0.0000000000000000\t0.3671359250169842\t-0.3425848839159632\t0.3283457496428495\t0.0000000000000000\t0.3689194771098271\t-0.3464936379774030\t0.3340185912267175\t0.0000000000000000\t0.3671359250169842\t-0.3431723933244590\t0.3409826857640367\t0.0000000000000000\t0.3671359250169842\t-0.3409978692691930\t0.3463523030395692\t0.0000000000000000\t0.3671359250169842\t-0.3356770523259974\t0.3506363783024263\t0.0000000000000000\t0.3671359250169842\t-0.3305529705086716\t0.3531958170313479\t0.0000000000000000\t0.3671359250169842\t-0.3261242050667670\t0.3565157077764454\t0.0000000000000000\r\n0.4629123289077153\t-0.3592753337637767\t0.1188424710682436\t0.0000000000000000\t0.4629123289077153\t-0.3961455582195348\t0.2468551635371455\t0.0000000000000000\t0.4610063144273182\t-0.4078131503047583\t0.3456317153666766\t0.0000000000000000\t0.4610063144273182\t-0.4336613559080322\t0.3719343122276372\t0.0000000000000000\t0.4610063144273182\t-0.4343780811673295\t0.3879270465443606\t0.0000000000000000\t0.4610063144273182\t-0.4337604569437492\t0.3994360003896873\t0.0000000000000000\t0.4610063144273182\t-0.4309855014982744\t0.4109175742066737\t0.0000000000000000\t0.4610063144273182\t-0.4263261298882018\t0.4192184431454539\t0.0000000000000000\t0.4610063144273182\t-0.4214466527152020\t0.4253481186747629\t0.0000000000000000\t0.4610063144273182\t-0.4162217639675419\t0.4289363399657696\t0.0000000000000000\t0.4667326950738877\t-0.4139340426836660\t0.4328083957106452\t0.0000000000000000\r\n0.5724736448682121\t-0.5459556676862879\t0.0524052118044550\t0.0000000000000000\t0.5724736448682121\t-0.4940989912441419\t0.2609468729150842\t0.0000000000000000\t0.5724736448682121\t-0.5244197561131690\t0.3692623500583355\t0.0000000000000000\t0.5724736448682121\t-0.5373997744456009\t0.4160099264706334\t0.0000000000000000\t0.5724736448682121\t-0.5361687971848075\t0.4384875505219825\t0.0000000000000000\t0.5724736448682121\t-0.5389852146215962\t0.4536227533883877\t0.0000000000000000\t0.5724736448682121\t-0.5349671762898730\t0.4733202527071914\t0.0000000000000000\t0.5724736448682121\t-0.5301767836189272\t0.4867374360740118\t0.0000000000000000\t0.5703899296732948\t-0.5232213788139769\t0.4973275945622862\t0.0000000000000000\t0.5703899296732948\t-0.5181423409572335\t0.5040215477815080\t0.0000000000000000\t0.5703899296732948\t-0.5118352135434456\t0.5103153396928193\t0.0000000000000000\r\n0.7004676747806673\t-0.8082412565209017\t-0.0634037590243930\t0.0000000000000000\t0.7004676747806673\t-0.6224259701282654\t0.2509742966933443\t0.0000000000000000\t0.7004676747806673\t-0.6469848704640956\t0.3824537561774100\t0.0000000000000000\t0.7004676747806673\t-0.6585490574246281\t0.4372421879402547\t0.0000000000000000\t0.7004676747806673\t-0.6592779562802864\t0.4661196573958219\t0.0000000000000000\t0.7004676747806673\t-0.6573717343650598\t0.4865668070365429\t0.0000000000000000\t0.6981287310371237\t-0.6529826553528034\t0.5130509121568261\t0.0000000000000000\t0.7004676747806673\t-0.6500174245829644\t0.5332136801039905\t0.0000000000000000\t0.6981287310371237\t-0.6420156948320364\t0.5494356244515167\t0.0000000000000000\t0.6981287310371237\t-0.6365619576849509\t0.5623462399512057\t0.0000000000000000\t0.6981287310371237\t-0.6303593959361240\t0.5739067524799967\t0.0000000000000000\r\n0.8432720672116305\t-0.8003772739772571\t-0.0179307346096546\t0.0000000000000000\t0.8432720672116305\t-0.8186647773910324\t0.1999751424310329\t0.0000000000000000\t0.8432720672116305\t-0.7801983209141452\t0.3767452557595226\t0.0000000000000000\t0.8432720672116305\t-0.7969533344567685\t0.4370136121768726\t0.0000000000000000\t0.8432720672116305\t-0.7950490039806231\t0.4691633420056094\t0.0000000000000000\t0.8379106495048978\t-0.7894034936610645\t0.4921747103907626\t0.0000000000000000\t0.8432720672116305\t-0.7880677689113339\t0.5184543435768094\t0.0000000000000000\t0.8432720672116305\t-0.7838715744675596\t0.5428662493313512\t0.0000000000000000\t0.8432720672116305\t-0.7775617623673021\t0.5646546016505375\t0.0000000000000000\t0.8432720672116305\t-0.7705293094482739\t0.5833766925023012\t0.0000000000000000\t0.8432720672116305\t-0.7641704745902068\t0.6014324072456010\t0.0000000000000000\r\n0.9999999999999999\t-0.9554471203838094\t-0.0858969643511720\t0.0000000000000000\t0.9999999999999999\t-0.9030897757420824\t0.1878781044403217\t0.0000000000000000\t0.9999999999999999\t-0.9404179116719943\t0.3500910830747300\t0.0000000000000000\t0.9999999999999999\t-0.9348029076345258\t0.4232170765432015\t0.0000000000000000\t0.9999999999999999\t-0.9414384556599829\t0.4537858750473681\t0.0000000000000000\t0.9999999999999999\t-0.9399485982004485\t0.4727859980819380\t0.0000000000000000\t0.9999999999999999\t-0.9349851356346648\t0.4953290283469364\t0.0000000000000000\t0.9999999999999999\t-0.9301726666670225\t0.5167867817836591\t0.0000000000000000\t0.9999999999999999\t-0.9224448768682160\t0.5399071976336627\t0.0000000000000000\t0.9999999999999999\t-0.9159353591364442\t0.5618090475012055\t0.0000000000000000\t0.9999999999999999\t-0.9089085884438031\t0.5839375995713647\t0.0000000000000000\r\n"
  out "E1, E2 maps for each method":string="E1' actual data (Volts)\tE2' actual data (Volts)\tE1' eff. angle method (Volts)\tE2' eff. angle method (Volts)\tE1' higher order eff. angle method (Volts)\tE2' higher order eff. angle method (Volts)\r\n2.3579666669999999\t2.9299833330000000\t2.0395896997665717\t2.9328725567299103\t2.3383503559788656\t2.9316284744959002\r\n2.3677166669999998\t2.9294583329999999\t2.2229759600321208\t2.9317042465898777\t2.3592701729486278\t2.9298814778055742\r\n2.4008333330000000\t2.9260500000000000\t2.3377343167669569\t2.9280299068921094\t2.4048236830520433\t2.9257250223026992\r\n2.4493749999999999\t2.9185666669999999\t2.4252876660973257\t2.9203955354098214\t2.4594505790418708\t2.9177220756629936\r\n2.5012333330000001\t2.9088250000000002\t2.4933951475581342\t2.9105498564271732\t2.5115913483381052\t2.9076529792842338\r\n2.5454750000000002\t2.8961416670000002\t2.5444962163141009\t2.8972084895806418\t2.5544939228716399\t2.8942399191403410\r\n2.5916916670000001\t2.8796666670000000\t2.5932962266712836\t2.8803907042279793\t2.5979496262689916\t2.8775059223987949\r\n2.6357833330000000\t2.8591916670000002\t2.6365116405011255\t2.8589275557438158\t2.6378890227350245\t2.8563540026666883\r\n2.6740083330000002\t2.8352249999999999\t2.6734852724476332\t2.8342193226229382\t2.6729624184416063\t2.8322389597734614\r\n2.7039083330000002\t2.8084750000000001\t2.7033947062654788\t2.8062562148127403\t2.7018303550309795\t2.8051956731962187\r\n2.7292333329999998\t2.7755916670000000\t2.7285827443609558\t2.7743852739265726\t2.7264793868299213\t2.7747012472666093\r\n2.7522583329999999\t2.7347416670000002\t2.7519825795542219\t2.7351857769490371\t2.7496761697964351\t2.7377544628056012\r\n2.7705500000000001\t2.6868083330000001\t2.7707162675015229\t2.6889651205445642\t2.7684960736541346\t2.6950384733553792\r\n2.7864583330000001\t2.6357333330000001\t2.7869251327715823\t2.6361899851827268\t2.7850102267006274\t2.6478961670718619\r\n2.7969249999999999\t2.5853166669999998\t2.7982097891734603\t2.5767009830581906\t2.7967509844150462\t2.5972697210789715\r\n2.8072916669999999\t2.5308250000000001\t2.8076664849362332\t2.5097557370787613\t2.8067764571536102\t2.5451810967499253\r\n2.8134833330000002\t2.4766949999999999\t2.8133766584614035\t2.4155406964295745\t2.8132596002773957\t2.4833141088915944\r\n2.8174833330000002\t2.4419083330000002\t2.8170945987406228\t2.2872498626066324\t2.8178884541640654\t2.4293442883413543\r\n2.8178166670000002\t2.4331749999999999\t2.8171173442379427\t2.0739015043781590\t2.8188839610583316\t2.4047536835037193\r\n2.3343583330000000\t2.8727916670000000\t2.0239861365087388\t2.8749489876388608\t2.3158879734420950\t2.8743595443189611\r\n2.3435000000000001\t2.8738916670000001\t2.1975417726471727\t2.8757064602648690\t2.3346533288434306\t2.8744167182193658\r\n2.3714750000000002\t2.8703249999999998\t2.3064220586468598\t2.8719611509911518\t2.3751365251972980\t2.8700709383334031\r\n2.4142416670000002\t2.8624833330000001\t2.3880671783238858\t2.8641129706694453\t2.4238198263324695\t2.8617459752350940\r\n2.4608750000000001\t2.8512000000000000\t2.4528463298915280\t2.8525716099039187\t2.4717792647178030\t2.8498721288557669\r\n2.5054500000000002\t2.8424999999999998\t2.5043471033652853\t2.8435738132132702\t2.5148485663699311\t2.8407023272977865\r\n2.5484416670000001\t2.8258666670000001\t2.5500597207993620\t2.8263240004930599\t2.5550039513135379\t2.8234453018600409\r\n2.5895250000000001\t2.8049416670000000\t2.5903600691464788\t2.8046603519516120\t2.5919002511243088\t2.8020074818932690\r\n2.6267416670000001\t2.7825500000000001\t2.6262022217331515\t2.7816750997190507\t2.6257747186158844\t2.7795390318909603\r\n2.6555416670000000\t2.7572416670000002\t2.6552012173959194\t2.7554273967253837\t2.6537006688968261\t2.7541545449172755\r\n2.6786083330000001\t2.7247833330000000\t2.6777746956268902\t2.7235055578770364\t2.6757295847117124\t2.7235750231381171\r\n2.7000750000000000\t2.6853333330000000\t2.6998398803254786\t2.6859049900378817\t2.6976016491294419\t2.6882208511098544\r\n2.7202500000000001\t2.6422333330000001\t2.7204207146156505\t2.6443183476483778\t2.7182867360527414\t2.6502011926536486\r\n2.7338249999999999\t2.5924333329999998\t2.7342713039074544\t2.5926269166959042\t2.7324792043794761\t2.6042743447956163\r\n2.7455750000000001\t2.5466750000000000\t2.7460446222696948\t2.5406178579450600\t2.7447152330790900\t2.5607784404159464\r\n2.7540749999999998\t2.4944783330000000\t2.7540552420019719\t2.4724338067578486\t2.7533725574405614\t2.5085053460411464\r\n2.7618916670000000\t2.4476916670000000\t2.7615081667655650\t2.3843136301964321\t2.7616548966630807\t2.4535044878158234\r\n2.7636250000000002\t2.4171916670000000\t2.7630099651968179\t2.2617445111296450\t2.7641303636212169\t2.4046965022006161\r\n2.7645749999999998\t2.4109500000000001\t2.7636004624758725\t2.0619468018969167\t2.7657590592939294\t2.3850742592889547\r\n2.3075791670000001\t2.8102583330000002\t2.0089964937990503\t2.8122092391196531\t2.2900992757661354\t2.8120202846450195\r\n2.3143783330000001\t2.8105000000000002\t2.1692451736672211\t2.8120127420867869\t2.3052373411332345\t2.8110647501828767\r\n2.3374916670000001\t2.8074750000000002\t2.2713373467921389\t2.8086762219285344\t2.3408120702512694\t2.8070707374121655\r\n2.3759583329999998\t2.8013416670000000\t2.3502255205959677\t2.8024289706437471\t2.3863658470930544\t2.8002834462357233\r\n2.4189250000000002\t2.7911000000000001\t2.4115654286773642\t2.7919544624384089\t2.4307625657786436\t2.7894306694399891\r\n2.4590999999999998\t2.7811166670000000\t2.4580286929991617\t2.7818944687275433\t2.4687541687154013\t2.7791719495193767\r\n2.4994583330000002\t2.7651666669999999\t2.5012275432366482\t2.7654734346188512\t2.5062212556052352\t2.7627114786855547\r\n2.5392833330000002\t2.7464333330000001\t2.5403090179369228\t2.7459954718144264\t2.5417904795306292\t2.7434336766945329\r\n2.5737250000000000\t2.7246416670000002\t2.5726117460105717\t2.7243539042023279\t2.5721200886672095\t2.7222775540908688\r\n2.6007166669999999\t2.6997666670000000\t2.6000648104747359\t2.6983837450669692\t2.5984393691881378\t2.6971844613138889\r\n2.6247250000000002\t2.6711583330000002\t2.6244175809892569\t2.6700834472656307\t2.6222284263428426\t2.6702787510211685\r\n2.6453000000000002\t2.6334916669999999\t2.6451453836987904\t2.6341096641725317\t2.6427817678884478\t2.6366281689017925\r\n2.6619666670000002\t2.5904416669999999\t2.6621251587267953\t2.5923034812904673\t2.6599037817614808\t2.5985140216684437\r\n2.6758500000000001\t2.5444249999999999\t2.6762182790962887\t2.5441240150503699\t2.6743812861950405\t2.5563365634294906\r\n2.6868249999999998\t2.5016850000000002\t2.6872064354138456\t2.4946668887373571\t2.6858800185168428\t2.5157277834205085\r\n2.6947916670000001\t2.4541700000000000\t2.6947609976576055\t2.4300238165174246\t2.6941400582634114\t2.4675550084744655\r\n2.7006916670000001\t2.4125916670000000\t2.7002517904340890\t2.3455625120289674\t2.7005295928331581\t2.4168745382417525\r\n2.7041916669999999\t2.3881000000000001\t2.7032373067701321\t2.2303196121775088\t2.7045660651345798\t2.3754795919178893\r\n2.7053166670000000\t2.3835083330000000\t2.7041616969929625\t2.0394752588310658\t2.7066081675391604\t2.3603966859582410\r\n2.2740350000000000\t2.7394500000000002\t1.9888965958821232\t2.7412722941471630\t2.2592353460317391\t2.7411826499505429\r\n2.2802375000000001\t2.7401583330000001\t2.1343538232445378\t2.7416112881648735\t2.2708863077094392\t2.7407401618922655\r\n2.2992593330000002\t2.7379166669999999\t2.2315222768149621\t2.7390906730983739\t2.3018633452963102\t2.7375151626217229\r\n2.3320333330000000\t2.7315749999999999\t2.3047654561740369\t2.7327589710081690\t2.3417254197323403\t2.7306160526915919\r\n2.3698583329999998\t2.7217166669999999\t2.3617349721094114\t2.7224881664885294\t2.3814274565447313\t2.7199466119961460\r\n2.4067666669999999\t2.7124750000000000\t2.4052785148382876\t2.7131907748388033\t2.4162716901086929\t2.7104369685913996\r\n2.4441916670000001\t2.6973583329999999\t2.4455624869313626\t2.6976100087209871\t2.4506487990414483\t2.6948099367453247\r\n2.4818250000000002\t2.6800666670000002\t2.4827199825730450\t2.6799921215729974\t2.4841929985006939\t2.6773927754172049\r\n2.5130499999999998\t2.6580416670000000\t2.5127447358120110\t2.6574732242119432\t2.5121447029676571\t2.6554016487178655\r\n2.5383499999999999\t2.6351333330000002\t2.5380161764700944\t2.6336273176606388\t2.5363137470211590\t2.6324570264792277\r\n2.5605583329999999\t2.6081249999999998\t2.5602590109407983\t2.6074583357850729\t2.5580235188590832\t2.6077087089170816\r\n2.5799750000000001\t2.5730083330000002\t2.5800899069953851\t2.5732514851668262\t2.5777160943799244\t2.5759559394444471\r\n2.5960666670000001\t2.5331666670000001\t2.5961032113458304\t2.5351484025649800\t2.5939200220338292\t2.5416134066039042\r\n2.6095083330000000\t2.4905450000000000\t2.6094937166066461\t2.4902476478674158\t2.6077560275977389\t2.5028929061626579\r\n2.6199750000000002\t2.4518916669999999\t2.6201074903450534\t2.4442717013574442\t2.6189430250224723\t2.4659864166354399\r\n2.6276833329999998\t2.4097916669999999\t2.6274218921703163\t2.3827933491868900\t2.6270535829437507\t2.4216415685885599\r\n2.6343500000000000\t2.3747750000000001\t2.6335720028504097\t2.3043131243740471\t2.6341924724784342\t2.3773936133675067\r\n2.6365666669999999\t2.3542083329999999\t2.6352651869411852\t2.1979727469950676\t2.6370115771767688\t2.3418766992389477\r\n2.6372249999999999\t2.3495416670000000\t2.6355371970178276\t2.0206328722204168\t2.6384940165840556\t2.3296455946375976\r\n2.2321166670000001\t2.6560999999999999\t1.9684294426581215\t2.6577172178134587\t2.2202101663833704\t2.6578836922781353\r\n2.2376083329999998\t2.6560333329999999\t2.0973561134959082\t2.6572554096634176\t2.2286043562002589\t2.6566140989136295\r\n2.2525750000000002\t2.6530250000000000\t2.1846371842787229\t2.6540636420544308\t2.2537015862099481\t2.6526936866308528\r\n2.2800241670000001\t2.6478999999999999\t2.2513211064978007\t2.6485005413472500\t2.2880886028809031\t2.6465401675612070\r\n2.3128224999999998\t2.6395000000000000\t2.3039914641539188\t2.6401139175293542\t2.3237292296665646\t2.6377331025544257\r\n2.3450083330000000\t2.6305749999999999\t2.3433959642607727\t2.6310204924832177\t2.3544433903813884\t2.6284150669358177\r\n2.3794666670000000\t2.6172666670000000\t2.3807513954922404\t2.6173186526483287\t2.3858891342469701\t2.6146533928379920\r\n2.4135749999999998\t2.6010249999999999\t2.4146312764018951\t2.6009186884995810\t2.4161571994053390\t2.5984478179293506\r\n2.4428333329999998\t2.5811833329999998\t2.4426120510207512\t2.5807339797714763\t2.4420854184734901\t2.5787888873502567\r\n2.4661166670000001\t2.5598083329999999\t2.4656681658104924\t2.5586917381341974\t2.4640734865814595\t2.5576545635213841\r\n2.4855499999999999\t2.5341833330000001\t2.4855116702976199\t2.5341124751896000\t2.4834304287479552\t2.5345096975866337\r\n2.5037333330000000\t2.5027591669999998\t2.5036302877301275\t2.5035525237550127\t2.5014677538275567\t2.5063743788185424\r\n2.5192749999999999\t2.4664025000000001\t2.5194475452450429\t2.4679454296724042\t2.5175482691966784\t2.4747007316821454\r\n2.5313500000000002\t2.4283833330000002\t2.5312301771259316\t2.4273112969791173\t2.5298423214509862\t2.4401875997107205\r\n2.5405500000000001\t2.3935749999999998\t2.5399759705665690\t2.3845636520256690\t2.5392317193639520\t2.4064660035973326\r\n2.5480333329999998\t2.3577916669999999\t2.5470386846550213\t2.3288217599125969\t2.5471697666667450\t2.3676313057223171\r\n2.5532666669999999\t2.3286416669999999\t2.5517085370270203\t2.2583688271283400\t2.5528945334315658\t2.3294278068141314\r\n2.5558833330000001\t2.3118500000000002\t2.5539792571543773\t2.1611533926393642\t2.5564004938563545\t2.2994994849500370\r\n2.5566333330000002\t2.3058500000000000\t2.5542437701077998\t2.0026571628304319\t2.5579639991190097\t2.2900290779522594\r\n2.1775000000000002\t2.5542500000000001\t1.9415555742813055\t2.5535039822684187\t2.1701290194757528\t2.5556156338827889\r\n2.1830250000000002\t2.5535416670000002\t2.0515760060873882\t2.5528409488885657\t2.1752481019937617\t2.5539334836982759\r\n2.1960166669999999\t2.5513249999999998\t2.1280333659204724\t2.5507638268717474\t2.1948604897554085\t2.5508994495111712\r\n2.2165416670000000\t2.5454166670000000\t2.1862304370459098\t2.5452617839041642\t2.2222903772082740\t2.5445722334409013\r\n2.2438583329999999\t2.5389666670000000\t2.2312505488906140\t2.5394665711806734\t2.2514025040047851\t2.5381504130275676\r\n2.2702916670000000\t2.5302500000000001\t2.2675988928831154\t2.5299799511187833\t2.2785020167160894\t2.5282010087853983\r\n2.2996759999999998\t2.5183249999999999\t2.3008771430343304\t2.5181277072658399\t2.3059413806125288\t2.5160476008130059\r\n2.3292166669999999\t2.5031358330000000\t2.3304276891400169\t2.5030703779449945\t2.3319406385634860\t2.5009302356624836\r\n2.3559749999999999\t2.4863166670000001\t2.3562600801360234\t2.4863587655058175\t2.3557911966161349\t2.4844811643729878\r\n2.3760916669999999\t2.4666950000000001\t2.3764373981884686\t2.4665699031511434\t2.3749772752480527\t2.4653454480928079\r\n2.3937666670000000\t2.4444666669999999\t2.3940665703904651\t2.4448853889365343\t2.3922038783313639\t2.4448336972957656\r\n2.4100833330000002\t2.4163500000000000\t2.4101404129061494\t2.4179339823593757\t2.4082944010114500\t2.4200098586485472\r\n2.4243666670000001\t2.3856666670000002\t2.4241174321996186\t2.3865429877992042\t2.4226408161080477\t2.3922233075293238\r\n2.4357583329999999\t2.3528916670000002\t2.4352097369385954\t2.3505529974037724\t2.4343636777940874\t2.3621283582934387\r\n2.4436166670000001\t2.3235916670000001\t2.4423728946928538\t2.3134500463252969\t2.4422582076255486\t2.3334807173521246\r\n2.4501916669999999\t2.2949333329999999\t2.4482738230449779\t2.2645432104356891\t2.4491471702855887\t2.3006666252684655\r\n2.4553416669999999\t2.2722166669999999\t2.4531560217556367\t2.2025800770307180\t2.4552254746024911\t2.2697560352357065\r\n2.4578833329999998\t2.2576166670000002\t2.4546899973480207\t2.1234607436460573\t2.4580452103119077\t2.2478443043679976\r\n2.4582000000000002\t2.2499500000000001\t2.4547346941160888\t1.9884250641875831\t2.4595552996241476\t2.2415854888313325\r\n2.1434833329999998\t2.4913675000000000\t1.9237891650455088\t2.4898848249321008\t2.1388703075628865\t2.4927400161895208\r\n2.1502083330000001\t2.4918591669999999\t2.0237367442566487\t2.4905347357014502\t2.1431099469176700\t2.4923198608678301\r\n2.1616333330000002\t2.4891800000000002\t2.0932279940783838\t2.4879445898397705\t2.1588467025521054\t2.4887143147054815\r\n2.1792166669999999\t2.4840724999999999\t2.1468994044775682\t2.4833563160886225\t2.1827500400170079\t2.4832433478433602\r\n2.2021833329999998\t2.4772233330000000\t2.1893423236250586\t2.4761883316962998\t2.2088200252962240\t2.4753652240812771\r\n2.2257333330000000\t2.4692133329999999\t2.2235347904198344\t2.4687610929179624\t2.2340989619211231\t2.4674320198639599\r\n2.2519166670000001\t2.4583266670000001\t2.2522805866379101\t2.4581809347785417\t2.2573987264012101\t2.4565234278259576\r\n2.2789400000000000\t2.4450916669999998\t2.2797447212212218\t2.4445771039115458\t2.2813113555610403\t2.4428068912367107\r\n2.3021067500000001\t2.4280249999999999\t2.3027860955210340\t2.4283441322009560\t2.3023811038298891\t2.4267895055529904\r\n2.3218883330000000\t2.4108833330000001\t2.3224978508706515\t2.4113104571718162\t2.3211207830190337\t2.4103615983426550\r\n2.3376666670000001\t2.3902916670000001\t2.3384555460351355\t2.3910674240644307\t2.3367052351734290\t2.3912490791293921\r\n2.3533249999999999\t2.3650166669999999\t2.3534162448591012\t2.3664434690486824\t2.3517208567333325\t2.3687063915906279\r\n2.3658250000000001\t2.3365333330000002\t2.3650708231710498\t2.3372965993788632\t2.3637825665278984\t2.3430220401927895\r\n2.3771583330000001\t2.3082500000000001\t2.3766806250384951\t2.3055545058027098\t2.3760663951051386\t2.3170506850911354\r\n2.3848583329999999\t2.2828416670000000\t2.3831410060243945\t2.2707692559592494\t2.3833188930501366\t2.2906883720483218\r\n2.3908583330000002\t2.2581416669999999\t2.3890381088767825\t2.2264662201276790\t2.3902597246905519\t2.2620510652975150\r\n2.3955750000000000\t2.2385083330000000\t2.3926846180386101\t2.1696188438039501\t2.3951605612875402\t2.2347724676556395\r\n2.3980583329999998\t2.2255333330000000\t2.3943701140777640\t2.0952170088433557\t2.3982430721836430\t2.2161551624453129\r\n2.3979333330000001\t2.2170083329999999\t2.3938533657737646\t1.9788862042908513\t2.3991986886511989\t2.2115758068653273\r\n2.1050916669999999\t2.4168500000000002\t1.9127402638136541\t2.4137325334227357\t2.1031063962079748\t2.4184506588112717\r\n2.1117916669999999\t2.4177083330000002\t1.9958246310782282\t2.4142631644164938\t2.1055858580074953\t2.4177188174051123\r\n2.1217166669999998\t2.4152583330000001\t2.0560693014720246\t2.4126225577875515\t2.1179118773200525\t2.4148584235364052\r\n2.1360083329999999\t2.4109500000000001\t2.1030325104939913\t2.4086686900143359\t2.1372275909775755\t2.4098137791561305\r\n2.1542916669999999\t2.4042833330000000\t2.1400995182298539\t2.4019585171104119\t2.1586888726529172\t2.4021899140704828\r\n2.1732416670000001\t2.3967083329999999\t2.1684423576164558\t2.3954861010982538\t2.1788271310352627\t2.3950610646593389\r\n2.1953499999999999\t2.3868499999999999\t2.1951081650589019\t2.3852835091352285\t2.1998726202469192\t2.3843109990040028\r\n2.2187583329999998\t2.3741666669999999\t2.2207469910199640\t2.3747534114946194\t2.2221484743301518\t2.3734655585315605\r\n2.2397000000000000\t2.3594166670000001\t2.2409859609023943\t2.3601173617975930\t2.2405824645436310\t2.3588524311755443\r\n2.2565833330000000\t2.3436249999999998\t2.2587704455430786\t2.3452968066194142\t2.2575547029220413\t2.3444593128731412\r\n2.2699833329999999\t2.3238916669999998\t2.2717594061651964\t2.3262130662683442\t2.2703340867252422\t2.3263376321193308\r\n2.2846758330000001\t2.3031166669999998\t2.2856179243336023\t2.3049916291479930\t2.2844236525152906\t2.3070234980919864\r\n2.2971474999999999\t2.2791250000000001\t2.2963414336278878\t2.2795788112205875\t2.2957341711881858\t2.2849086800034519\r\n2.3069916670000001\t2.2548499999999998\t2.3044821077412991\t2.2498740226742204\t2.3047340741860558\t2.2607567907770889\r\n2.3146800000000001\t2.2347333329999999\t2.3117189407415295\t2.2204999766665585\t2.3129294552874535\t2.2395960527336158\r\n2.3208058330000001\t2.2148750000000001\t2.3172051349855818\t2.1818781755412364\t2.3196459325088279\t2.2160846035695516\r\n2.3247091670000000\t2.1991000000000001\t2.3201880631609542\t2.1322226322316244\t2.3240772720804843\t2.1942160777261446\r\n2.3268333330000002\t2.1878750000000000\t2.3210110378067368\t2.0678940799316967\t2.3264876888333275\t2.1800156722641160\r\n2.3271250000000001\t2.1803583330000000\t2.3217851908992997\t1.9722390346352847\t2.3289343815238182\t2.1785288618302885\r\n2.0602083329999998\t2.3236666669999999\t1.8945741084460315\t2.3160192660819017\t2.0626720498635471\t2.3254667149933739\r\n2.0647416669999998\t2.3234916669999999\t1.9579945301777324\t2.3147606361792992\t2.0603578405384124\t2.3223407345237268\r\n2.0721750000000001\t2.3222749999999999\t2.0085059309727127\t2.3170264818831048\t2.0687369797223232\t2.3228151932054719\r\n2.0817916670000001\t2.3177083330000001\t2.0454816829280649\t2.3115221438264446\t2.0790309931676458\t2.3155822498434677\r\n2.0951333330000002\t2.3128166669999999\t2.0780523505434103\t2.3088780631345016\t2.0960300617523631\t2.3114415975864317\r\n2.1082666670000001\t2.3056999999999999\t2.1007099247871599\t2.3024682957730995\t2.1102045261773608\t2.3038554567246399\r\n2.1244999999999998\t2.2963916670000000\t2.1227701507283316\t2.2940263188045642\t2.1264836177437183\t2.2942966064052577\r\n2.1421666670000001\t2.2852583329999998\t2.1452533220281285\t2.2867307510115102\t2.1456055329825201\t2.2861110610925035\r\n2.1578333330000001\t2.2717583330000002\t2.1613408743870957\t2.2739070639043182\t2.1600330708935993\t2.2727610822130821\r\n2.1720666670000002\t2.2582416670000001\t2.1765915224451970\t2.2622537562270653\t2.1747041296043985\t2.2610336823042854\r\n2.1853250000000002\t2.2438083330000000\t2.1879316211980124\t2.2471645887868465\t2.1861316598790248\t2.2464437935778672\r\n2.1978916669999999\t2.2268249999999998\t2.1983138379371079\t2.2288322881824261\t2.1971209732448242\t2.2295584474779031\r\n2.2085750000000002\t2.2084250000000001\t2.2082405123256605\t2.2090979552250873\t2.2080460882958683\t2.2127115999283027\r\n2.2177166669999999\t2.1911749999999999\t2.2130869597131904\t2.1830435817613303\t2.2142151042228972\t2.1919024572594381\r\n2.2262333330000001\t2.1776583330000001\t2.2238229762489512\t2.1635665646687663\t2.2263180586584856\t2.1801952510387896\r\n2.2299083330000000\t2.1629583330000002\t2.2247055338315920\t2.1302079651857735\t2.2288885158442500\t2.1607837959550262\r\n2.2349833330000002\t2.1523083330000001\t2.2283665816600475\t2.0920478960885767\t2.2345163014586076\t2.1474263279081578\r\n2.2355416670000001\t2.1430333330000000\t2.2280073959394491\t2.0426169279397808\t2.2362468566696942\t2.1389030046037796\r\n2.2367249999999999\t2.1377166669999998\t2.2268507673957147\t1.9760802393018486\t2.2372400818313447\t2.1389112820815122\r\n2.0031583330000000\t2.1960250000000001\t1.9019612645998605\t2.1831421859349507\t2.0081588878691328\t2.1976404350378567\r\n2.0045999999999999\t2.1949000000000001\t1.9319746950658814\t2.1830336647272226\t2.0039875824271043\t2.1949519062093539\r\n2.0074833330000001\t2.1930499999999999\t1.9584065903439416\t2.1826576229729575\t2.0035360947586591\t2.1920273716756120\r\n2.0119250000000002\t2.1903666670000002\t1.9801641259671172\t2.1801844568774982\t2.0059225051618341\t2.1871525078010197\r\n2.0170333330000001\t2.1855416669999999\t2.0000274625477767\t2.1788799536517498\t2.0130992447705691\t2.1837401331474653\r\n2.0236333329999998\t2.1812083329999998\t2.0162489268636810\t2.1777133679827481\t2.0220456271373544\t2.1809144764269583\r\n2.0313416670000000\t2.1737250000000001\t2.0286520782094364\t2.1707048282156798\t2.0294429076397300\t2.1722597936161585\r\n2.0397916669999998\t2.1643750000000002\t2.0419486186959115\t2.1649401743976786\t2.0401618078465047\t2.1651474904973740\r\n2.0486416670000001\t2.1545083329999999\t2.0529522074309767\t2.1574905104636430\t2.0504270297604310\t2.1568028159743058\r\n2.0583250000000000\t2.1458750000000002\t2.0651530618072602\t2.1522677806504142\t2.0630700092522662\t2.1512481057232393\r\n2.0650333330000001\t2.1343250000000000\t2.0666295474425942\t2.1368143195021050\t2.0658101545565470\t2.1361673035829787\r\n2.0748666670000002\t2.1247666669999998\t2.0773227366920373\t2.1285187336793170\t2.0784776331032386\t2.1292989369291262\r\n2.0832999999999999\t2.1147499999999999\t2.0823995257905596\t2.1140351068652841\t2.0860819442264806\t2.1178731597677332\r\n2.0910083330000000\t2.1058833330000000\t2.0849526345171618\t2.0971600975349647\t2.0914336463851146\t2.1061634918419938\r\n2.0972083330000002\t2.0990750000000000\t2.0864196057127251\t2.0796416941451303\t2.0957559686116736\t2.0962651165977686\r\n2.1020249999999998\t2.0923416669999999\t2.0890605762920598\t2.0600755150567536\t2.1017074652566765\t2.0891387266941703\r\n2.1062166670000000\t2.0873249999999999\t2.0896839126202984\t2.0348423236542255\t2.1060469717271464\t2.0837032208741397\r\n2.1089833329999998\t2.0837249999999998\t2.0845169297931143\t2.0019675828935743\t2.1045492973006641\t2.0786918971248558\r\n2.1112916670000001\t2.0818833329999999\t2.0896757218574296\t1.9679402695348538\t2.1139565471797277\t2.0860855205854398\r\n1.9603916669999999\t2.1036166669999998\t1.8934688001273940\t2.0760101295912388\t1.9575788692332172\t2.0993450708002266\r\n1.9639500000000001\t2.1090666670000000\t1.9150391481407605\t2.0880779278329378\t1.9638754448679856\t2.1081859723393812\r\n1.9648583330000000\t2.1094166670000001\t1.9375643137532430\t2.1007171609491402\t1.9718851848727175\t2.1172539074645957\r\n1.9647833330000000\t2.1051083330000000\t1.9452415389350925\t2.0953221654156229\t1.9657952573738438\t2.1074171893413549\r\n1.9650666670000001\t2.0985000000000000\t1.9550332022470638\t2.0939099746666976\t1.9656095922632972\t2.1021547889051000\r\n1.9663583330000001\t2.0928749999999998\t1.9642891216107354\t2.0939175677102417\t1.9684471598944637\t2.0990573928252814\r\n1.9673416669999999\t2.0863999999999998\t1.9652918270304494\t2.0840508359044243\t1.9645307106499681\t2.0859254402479026\r\n1.9705333330000001\t2.0802000000000000\t1.9665350032635691\t2.0747891686994242\t1.9630488586900885\t2.0738583707786344\r\n1.9759333330000000\t2.0757916669999998\t1.9782059506058267\t2.0766180654902922\t1.9737393912563916\t2.0734453420996939\r\n1.9812083330000001\t2.0706166669999999\t1.9826551832974333\t2.0714914989147863\t1.9787210752237252\t2.0669094436170874\r\n1.9869916670000001\t2.0655083329999999\t1.9974601612851701\t2.0761059125300494\t1.9950392155024053\t2.0708341977011009\r\n1.9886999999999999\t2.0561500000000001\t1.9923386963545016\t2.0609213301259333\t1.9926978447339572\t2.0566333134353028\r\n1.9939833330000001\t2.0512166669999998\t1.9916189875950911\t2.0494920321920445\t1.9955596231884831\t2.0480645848067485\r\n1.9985250000000001\t2.0469833330000000\t1.9922865106934413\t2.0395649531157347\t2.0001865052800407\t2.0431501331204016\r\n2.0033666669999999\t2.0445500000000001\t1.9955094259535489\t2.0309281417320171\t2.0080080426725826\t2.0425933159008554\r\n2.0072916670000001\t2.0421833330000001\t1.9882902965039071\t2.0129827696169316\t2.0054975528492105\t2.0360097778954516\r\n2.0103749999999998\t2.0405666669999998\t1.9777719086080350\t1.9911729128344049\t2.0000078973718614\t2.0297592737895616\r\n2.0160833330000001\t2.0411750000000000\t1.9882748694566297\t1.9816940824139573\t2.0175964547338414\t2.0441717971286488\r\n2.0187750000000002\t2.0414916669999998\t1.9863117544070898\t1.9611513314605555\t2.0219756231439270\t2.0504677149198711\r\n"
  out "Effective angle X plot_":cluster{dbl[], dbl[]}[](graph)=[{[-0.9999999999999999, -0.8459634362504808, -0.7028117712403573, -0.5745611109571804, -0.46100631442731815, -0.3689194771098271, -0.2718814121476857, -0.17614702688068878, -0.08502702101131297, 0.0, 0.0834450784477064, 0.17452793889436508, 0.26851046270375567, 0.3689194771098271, 0.46100631442731815, 0.5724736448682121, 0.7004676747806673, 0.8432720672116305, 0.9999999999999999], [0.5188418104065096, 0.5527709767869218, 0.5825100736406964, 0.5655852803690335, 0.5367013693167687, 0.4814947359213608, 0.3962036651655259, 0.30247519912185106, 0.17277511041312554, 0.04857134994753296, -0.11477703146300927, -0.31186458327001015, -0.5123196133813664, -0.806225280413884, -0.9819378661710078, -1.3238555928281337, -1.7125591635376343, -2.169106061785542, -2.765221671937504]}, {[-0.9999999999999999, -0.8459634362504808, -0.7028117712403573, -0.5745611109571804, -0.46100631442731815, -0.3689194771098271, -0.2718814121476857, -0.17614702688068878, -0.08502702101131297, 0.0, 0.0834450784477064, 0.17452793889436508, 0.26851046270375567, 0.3689194771098271, 0.46100631442731815, 0.5724736448682121, 0.7004676747806673, 0.8432720672116305, 0.9999999999999999], [-2.710746560468574, -2.2324745574527904, -1.6930687846557417, -1.3559695335879334, -1.0119826258435312, -0.7770192864712264, -0.544617206312469, -0.29219526836191667, -0.1124460755508965, 0.05517968998527327, 0.1823015191280195, 0.30604462473121935, 0.42449546439284996, 0.49426662300606755, 0.5718021480660419, 0.6021700169460663, 0.6186366367406101, 0.611553523781737, 0.5776183997010226]}, {[-0.9999999999999999, -0.8459634362504808, -0.7028117712403573, -0.5745611109571804, -0.46100631442731815, -0.3689194771098271, -0.2718814121476857, -0.17614702688068878, -0.08502702101131297, 0.0, 0.0834450784477064, 0.17452793889436508, 0.26851046270375567, 0.3689194771098271, 0.46100631442731815, 0.5724736448682121, 0.7004676747806673, 0.8432720672116305, 0.9999999999999999], [0.5019896305748249, 0.5792706211983512, 0.6016610033211531, 0.5812787539845566, 0.5313291123028855, 0.4688203592849763, 0.38162762409276796, 0.2741639698201765, 0.15209777501455407, 0.020792179522619768, -0.12440427224684139, -0.3013603842087858, -0.5041583453049923, -0.7435017841584197, -0.983603543532702, -1.3005993546185817, -1.7002055402395366, -2.1909817665541462, -2.7841533319516247]}, {[-0.9999999999999999, -0.8459634362504808, -0.7028117712403573, -0.5745611109571804, -0.46100631442731815, -0.3689194771098271, -0.2718814121476857, -0.17614702688068878, -0.08502702101131297, 0.0, 0.0834450784477064, 0.17452793889436508, 0.26851046270375567, 0.3689194771098271, 0.46100631442731815, 0.5724736448682121, 0.7004676747806673, 0.8432720672116305, 0.9999999999999999], [-2.775453643139415, -2.1968375982636825, -1.7071271648913744, -1.3076789676725487, -0.9849942600134657, -0.7446882768884536, -0.5121759440962989, -0.30361736510901655, -0.12432862939743507, 0.026066724526630485, 0.15779656128314734, 0.28364140853636544, 0.393861287390072, 0.48958734148827554, 0.5573717280147603, 0.613812254983678, 0.6440268523548214, 0.6340896215868709, 0.5701968170808951]}]
  out "Variation of tangential cooling coefficient k with speed":cluster{dbl[], dbl[]}[](graph)=[{[0.5018157894736842, 0.9994315789473684, 2.000205263157895, 3.000784210526316, 3.999947368421053, 4.999831578947369, 6.999731578947368, 9.001931578947369, 10.999973684210525, 13.000168421052631, 15.001142105263158], [0.6599332295131558, 0.4477378321660209, 0.34828545249797827, 0.31807013530431494, 0.2973863116337986, 0.28489637828096237, 0.26428007716046986, 0.24630640318961317, 0.22853993548777038, 0.21065320811782534, 0.19388724748060474]}, {[0.5018157894736842, 0.9994315789473684, 2.000205263157895, 3.000784210526316, 3.999947368421053, 4.999831578947369, 6.999731578947368, 9.001931578947369, 10.999973684210525, 13.000168421052631, 15.001142105263158], [0.5182677319056692, 0.41473631513087905, 0.32080035855951117, 0.28809804664311733, 0.2724916341605897, 0.25911280970809947, 0.24102249710370885, 0.22363651876587745, 0.20284807265933522, 0.185171512574672, 0.1681952069880479]}]
  out "Probe zero alignment error_":cluster{dbl[], dbl[]}(graph)={[0.5018157894736842, 0.9994315789473684, 2.000205263157895, 3.000784210526316, 3.999947368421053, 4.999831578947369, 6.999731578947368, 9.001931578947369, 10.999973684210525, 13.000168421052631, 15.001142105263158], [1.8585307868990102, -0.2685545800236653, 0.08119165501176207, 0.1267064250649524, -0.0312381845532423, 0.007585223590221665, -0.023077773706953575, 0.010416188082381303, 0.11600317142857608, 0.11452298300636243, 0.07775446760172378]}
  out "Effective angle variation with speed_":cluster{dbl[], dbl[]}[](graph)=[{[0.5018157894736842, 0.9994315789473684, 2.000205263157895, 3.000784210526316, 3.999947368421053, 4.999831578947369, 6.999731578947368, 9.001931578947369, 10.999973684210525, 13.000168421052631, 15.001142105263158], [-71.84404986346983, -50.796721198363066, -47.414202598296825, -46.52106063699666, -46.1290205114914, -45.82524482883317, -45.289643706169564, -44.86750967600907, -44.40532316758195, -44.006792057649086, -43.62526257388144]}, {[0.5018157894736842, 0.9994315789473684, 2.000205263157895, 3.000784210526316, 3.999947368421053, 4.999831578947369, 6.999731578947368, 9.001931578947369, 10.999973684210525, 13.000168421052631, 15.001142105263158], [62.96368771729303, 49.01609711214064, 46.72387397779648, 46.40001687940649, 46.25206996927475, 46.03121768509195, 45.49666121473799, 45.0959281609883, 44.49861664127186, 43.96372739008556, 43.5843363193316]}]
  out "Wire angle error with speed_":cluster{dbl[], dbl[]}[](graph)=[{[0.5018157894736842, 0.9994315789473684, 2.000205263157895, 3.000784210526316, 3.999947368421053, 4.999831578947369, 6.999731578947368, 9.001931578947369, 10.999973684210525, 13.000168421052631, 15.001142105263158], [6.626753335529527, -1.5238812538482893, -0.7133248964583326, 0.17606318381092093, 0.19064878878848493, 0.228238769612569, 0.12631593545035208, -0.05654620044266492, -0.25392908228482053, -0.5118579225506359, -0.7550503383633456]}, {[0.5018157894736842, 0.9994315789473684, 2.000205263157895, 3.000784210526316, 3.999947368421053, 4.999831578947369, 6.999731578947368, 9.001931578947369, 10.999973684210525, 13.000168421052631, 15.001142105263158], [-2.9096917617315063, 0.9867720938009588, 0.8757082064818568, 0.07734966631898385, -0.25312515789496953, -0.21306832243212567, -0.17247148286425923, 0.07737857660742753, 0.4859354251419727, 0.7409038885633608, 0.9105592735667931]}]
  out "E1', E2' map synthesized from effective angle methods LS fits":cluster{dbl[], dbl[]}[](graph)=[{[2.357966667, 2.367716667, 2.400833333, 2.449375, 2.501233333, 2.545475, 2.591691667, 2.635783333, 2.674008333, 2.703908333, 2.729233333, 2.752258333, 2.77055, 2.786458333, 2.796925, 2.807291667, 2.813483333, 2.817483333, 2.817816667, 2.334358333, 2.3435, 2.371475, 2.414241667, 2.460875, 2.50545, 2.548441667, 2.589525, 2.626741667, 2.655541667, 2.678608333, 2.700075, 2.72025, 2.733825, 2.745575, 2.754075, 2.761891667, 2.763625, 2.764575, 2.307579167, 2.314378333, 2.337491667, 2.375958333, 2.418925, 2.4591, 2.499458333, 2.539283333, 2.573725, 2.600716667, 2.624725, 2.6453, 2.661966667, 2.67585, 2.686825, 2.694791667, 2.700691667, 2.704191667, 2.705316667, 2.274035, 2.2802375, 2.299259333, 2.332033333, 2.369858333, 2.406766667, 2.444191667, 2.481825, 2.51305, 2.53835, 2.560558333, 2.579975, 2.596066667, 2.609508333, 2.619975, 2.627683333, 2.63435, 2.636566667, 2.637225, 2.232116667, 2.237608333, 2.252575, 2.280024167, 2.3128225, 2.345008333, 2.379466667, 2.413575, 2.442833333, 2.466116667, 2.48555, 2.503733333, 2.519275, 2.53135, 2.54055, 2.548033333, 2.553266667, 2.555883333, 2.556633333, 2.1775, 2.183025, 2.196016667, 2.216541667, 2.243858333, 2.270291667, 2.299676, 2.329216667, 2.355975, 2.376091667, 2.393766667, 2.410083333, 2.424366667, 2.435758333, 2.443616667, 2.450191667, 2.455341667, 2.457883333, 2.4582, 2.143483333, 2.150208333, 2.161633333, 2.179216667, 2.202183333, 2.225733333, 2.251916667, 2.27894, 2.30210675, 2.321888333, 2.337666667, 2.353325, 2.365825, 2.377158333, 2.384858333, 2.390858333, 2.395575, 2.398058333, 2.397933333, 2.105091667, 2.111791667, 2.121716667, 2.136008333, 2.154291667, 2.173241667, 2.19535, 2.218758333, 2.2397, 2.256583333, 2.269983333, 2.284675833, 2.2971475, 2.306991667, 2.31468, 2.320805833, 2.324709167, 2.326833333, 2.327125, 2.060208333, 2.064741667, 2.072175, 2.081791667, 2.095133333, 2.108266667, 2.1245, 2.142166667, 2.157833333, 2.172066667, 2.185325, 2.197891667, 2.208575, 2.217716667, 2.226233333, 2.229908333, 2.234983333, 2.235541667, 2.236725, 2.003158333, 2.0046, 2.007483333, 2.011925, 2.017033333, 2.023633333, 2.031341667, 2.039791667, 2.048641667, 2.058325, 2.065033333, 2.074866667, 2.0833, 2.091008333, 2.097208333, 2.102025, 2.106216667, 2.108983333, 2.111291667, 1.960391667, 1.96395, 1.964858333, 1.964783333, 1.965066667, 1.966358333, 1.967341667, 1.970533333, 1.975933333, 1.981208333, 1.986991667, 1.9887, 1.993983333, 1.998525, 2.003366667, 2.007291667, 2.010375, 2.016083333, 2.018775], [2.929983333, 2.929458333, 2.92605, 2.918566667, 2.908825, 2.896141667, 2.879666667, 2.859191667, 2.835225, 2.808475, 2.775591667, 2.734741667, 2.686808333, 2.635733333, 2.585316667, 2.530825, 2.476695, 2.441908333, 2.433175, 2.872791667, 2.873891667, 2.870325, 2.862483333, 2.8512, 2.8425, 2.825866667, 2.804941667, 2.78255, 2.757241667, 2.724783333, 2.685333333, 2.642233333, 2.592433333, 2.546675, 2.494478333, 2.447691667, 2.417191667, 2.41095, 2.810258333, 2.8105, 2.807475, 2.801341667, 2.7911, 2.781116667, 2.765166667, 2.746433333, 2.724641667, 2.699766667, 2.671158333, 2.633491667, 2.590441667, 2.544425, 2.501685, 2.45417, 2.412591667, 2.3881, 2.383508333, 2.73945, 2.740158333, 2.737916667, 2.731575, 2.721716667, 2.712475, 2.697358333, 2.680066667, 2.658041667, 2.635133333, 2.608125, 2.573008333, 2.533166667, 2.490545, 2.451891667, 2.409791667, 2.374775, 2.354208333, 2.349541667, 2.6561, 2.656033333, 2.653025, 2.6479, 2.6395, 2.630575, 2.617266667, 2.601025, 2.581183333, 2.559808333, 2.534183333, 2.502759167, 2.4664025, 2.428383333, 2.393575, 2.357791667, 2.328641667, 2.31185, 2.30585, 2.55425, 2.553541667, 2.551325, 2.545416667, 2.538966667, 2.53025, 2.518325, 2.503135833, 2.486316667, 2.466695, 2.444466667, 2.41635, 2.385666667, 2.352891667, 2.323591667, 2.294933333, 2.272216667, 2.257616667, 2.24995, 2.4913675, 2.491859167, 2.48918, 2.4840725, 2.477223333, 2.469213333, 2.458326667, 2.445091667, 2.428025, 2.410883333, 2.390291667, 2.365016667, 2.336533333, 2.30825, 2.282841667, 2.258141667, 2.238508333, 2.225533333, 2.217008333, 2.41685, 2.417708333, 2.415258333, 2.41095, 2.404283333, 2.396708333, 2.38685, 2.374166667, 2.359416667, 2.343625, 2.323891667, 2.303116667, 2.279125, 2.25485, 2.234733333, 2.214875, 2.1991, 2.187875, 2.180358333, 2.323666667, 2.323491667, 2.322275, 2.317708333, 2.312816667, 2.3057, 2.296391667, 2.285258333, 2.271758333, 2.258241667, 2.243808333, 2.226825, 2.208425, 2.191175, 2.177658333, 2.162958333, 2.152308333, 2.143033333, 2.137716667, 2.196025, 2.1949, 2.19305, 2.190366667, 2.185541667, 2.181208333, 2.173725, 2.164375, 2.154508333, 2.145875, 2.134325, 2.124766667, 2.11475, 2.105883333, 2.099075, 2.092341667, 2.087325, 2.083725, 2.081883333, 2.103616667, 2.109066667, 2.109416667, 2.105108333, 2.0985, 2.092875, 2.0864, 2.0802, 2.075791667, 2.070616667, 2.065508333, 2.05615, 2.051216667, 2.046983333, 2.04455, 2.042183333, 2.040566667, 2.041175, 2.041491667]}, {[2.0395896997665717, 2.222975960032121, 2.337734316766957, 2.4252876660973257, 2.493395147558134, 2.544496216314101, 2.5932962266712836, 2.6365116405011255, 2.6734852724476332, 2.703394706265479, 2.728582744360956, 2.751982579554222, 2.770716267501523, 2.7869251327715823, 2.7982097891734603, 2.807666484936233, 2.8133766584614035, 2.817094598740623, 2.8171173442379427, 2.023986136508739, 2.1975417726471727, 2.30642205864686, 2.388067178323886, 2.452846329891528, 2.5043471033652853, 2.550059720799362, 2.5903600691464788, 2.6262022217331515, 2.6552012173959194, 2.67777469562689, 2.6998398803254786, 2.7204207146156505, 2.7342713039074544, 2.746044622269695, 2.754055242001972, 2.761508166765565, 2.763009965196818, 2.7636004624758725, 2.0089964937990503, 2.169245173667221, 2.271337346792139, 2.3502255205959677, 2.4115654286773642, 2.4580286929991617, 2.501227543236648, 2.5403090179369228, 2.5726117460105717, 2.600064810474736, 2.624417580989257, 2.6451453836987904, 2.6621251587267953, 2.6762182790962887, 2.6872064354138456, 2.6947609976576055, 2.700251790434089, 2.703237306770132, 2.7041616969929625, 1.9888965958821232, 2.134353823244538, 2.231522276814962, 2.304765456174037, 2.3617349721094114, 2.4052785148382876, 2.4455624869313626, 2.482719982573045, 2.512744735812011, 2.5380161764700944, 2.5602590109407983, 2.580089906995385, 2.5961032113458304, 2.609493716606646, 2.6201074903450534, 2.6274218921703163, 2.6335720028504097, 2.635265186941185, 2.6355371970178276, 1.9684294426581215, 2.0973561134959082, 2.184637184278723, 2.2513211064978007, 2.3039914641539188, 2.3433959642607727, 2.3807513954922404, 2.414631276401895, 2.442612051020751, 2.4656681658104924, 2.48551167029762, 2.5036302877301275, 2.519447545245043, 2.5312301771259316, 2.539975970566569, 2.5470386846550213, 2.5517085370270203, 2.5539792571543773, 2.5542437701078, 1.9415555742813055, 2.051576006087388, 2.1280333659204724, 2.18623043704591, 2.231250548890614, 2.2675988928831154, 2.3008771430343304, 2.330427689140017, 2.3562600801360234, 2.3764373981884686, 2.394066570390465, 2.4101404129061494, 2.4241174321996186, 2.4352097369385954, 2.442372894692854, 2.448273823044978, 2.4531560217556367, 2.4546899973480207, 2.454734694116089, 1.9237891650455088, 2.0237367442566487, 2.093227994078384, 2.146899404477568, 2.1893423236250587, 2.2235347904198344, 2.25228058663791, 2.279744721221222, 2.302786095521034, 2.3224978508706515, 2.3384555460351355, 2.353416244859101, 2.3650708231710498, 2.376680625038495, 2.3831410060243945, 2.3890381088767825, 2.39268461803861, 2.394370114077764, 2.3938533657737646, 1.9127402638136541, 1.9958246310782282, 2.0560693014720246, 2.1030325104939913, 2.140099518229854, 2.1684423576164558, 2.195108165058902, 2.220746991019964, 2.2409859609023943, 2.2587704455430786, 2.2717594061651964, 2.2856179243336023, 2.296341433627888, 2.304482107741299, 2.3117189407415295, 2.317205134985582, 2.320188063160954, 2.321011037806737, 2.3217851908992997, 1.8945741084460315, 1.9579945301777324, 2.0085059309727127, 2.045481682928065, 2.0780523505434103, 2.10070992478716, 2.1227701507283316, 2.1452533220281285, 2.1613408743870957, 2.176591522445197, 2.1879316211980124, 2.198313837937108, 2.2082405123256605, 2.2130869597131904, 2.223822976248951, 2.224705533831592, 2.2283665816600475, 2.228007395939449, 2.2268507673957147, 1.9019612645998605, 1.9319746950658814, 1.9584065903439416, 1.9801641259671172, 2.0000274625477767, 2.016248926863681, 2.0286520782094364, 2.0419486186959115, 2.0529522074309767, 2.06515306180726, 2.066629547442594, 2.0773227366920373, 2.0823995257905596, 2.084952634517162, 2.086419605712725, 2.0890605762920598, 2.0896839126202984, 2.0845169297931143, 2.0896757218574296, 1.893468800127394, 1.9150391481407605, 1.937564313753243, 1.9452415389350926, 1.9550332022470638, 1.9642891216107354, 1.9652918270304494, 1.9665350032635691, 1.9782059506058267, 1.9826551832974333, 1.9974601612851701, 1.9923386963545016, 1.9916189875950912, 1.9922865106934413, 1.9955094259535489, 1.988290296503907, 1.977771908608035, 1.9882748694566297, 1.9863117544070898], [2.9328725567299103, 2.9317042465898777, 2.9280299068921094, 2.9203955354098214, 2.9105498564271732, 2.897208489580642, 2.8803907042279793, 2.858927555743816, 2.834219322622938, 2.8062562148127403, 2.7743852739265726, 2.735185776949037, 2.688965120544564, 2.636189985182727, 2.5767009830581906, 2.5097557370787613, 2.4155406964295745, 2.2872498626066324, 2.073901504378159, 2.8749489876388608, 2.875706460264869, 2.871961150991152, 2.8641129706694453, 2.8525716099039187, 2.84357381321327, 2.82632400049306, 2.804660351951612, 2.7816750997190507, 2.7554273967253837, 2.7235055578770364, 2.6859049900378817, 2.644318347648378, 2.592626916695904, 2.54061785794506, 2.4724338067578486, 2.384313630196432, 2.261744511129645, 2.0619468018969167, 2.812209239119653, 2.812012742086787, 2.8086762219285344, 2.802428970643747, 2.791954462438409, 2.7818944687275433, 2.765473434618851, 2.7459954718144264, 2.724353904202328, 2.698383745066969, 2.6700834472656307, 2.6341096641725317, 2.5923034812904673, 2.54412401505037, 2.494666888737357, 2.4300238165174246, 2.3455625120289674, 2.230319612177509, 2.039475258831066, 2.741272294147163, 2.7416112881648735, 2.739090673098374, 2.732758971008169, 2.7224881664885294, 2.7131907748388033, 2.697610008720987, 2.6799921215729974, 2.657473224211943, 2.633627317660639, 2.607458335785073, 2.5732514851668262, 2.53514840256498, 2.490247647867416, 2.444271701357444, 2.38279334918689, 2.304313124374047, 2.1979727469950676, 2.0206328722204168, 2.6577172178134587, 2.6572554096634176, 2.654063642054431, 2.64850054134725, 2.640113917529354, 2.6310204924832177, 2.6173186526483287, 2.600918688499581, 2.5807339797714763, 2.5586917381341974, 2.5341124751896, 2.5035525237550127, 2.467945429672404, 2.4273112969791173, 2.384563652025669, 2.328821759912597, 2.25836882712834, 2.1611533926393642, 2.002657162830432, 2.5535039822684187, 2.5528409488885657, 2.5507638268717474, 2.5452617839041642, 2.5394665711806734, 2.5299799511187833, 2.51812770726584, 2.5030703779449945, 2.4863587655058175, 2.4665699031511434, 2.4448853889365343, 2.4179339823593757, 2.386542987799204, 2.3505529974037724, 2.313450046325297, 2.264543210435689, 2.202580077030718, 2.1234607436460573, 1.9884250641875831, 2.489884824932101, 2.4905347357014502, 2.4879445898397705, 2.4833563160886225, 2.4761883316963, 2.4687610929179624, 2.4581809347785417, 2.444577103911546, 2.428344132200956, 2.4113104571718162, 2.3910674240644307, 2.3664434690486824, 2.3372965993788632, 2.30555450580271, 2.2707692559592494, 2.226466220127679, 2.16961884380395, 2.0952170088433557, 1.9788862042908513, 2.4137325334227357, 2.414263164416494, 2.4126225577875515, 2.408668690014336, 2.401958517110412, 2.3954861010982538, 2.3852835091352285, 2.3747534114946194, 2.360117361797593, 2.345296806619414, 2.3262130662683442, 2.304991629147993, 2.2795788112205875, 2.2498740226742204, 2.2204999766665585, 2.1818781755412364, 2.1322226322316244, 2.0678940799316967, 1.9722390346352847, 2.3160192660819017, 2.314760636179299, 2.317026481883105, 2.3115221438264446, 2.3088780631345016, 2.3024682957730995, 2.294026318804564, 2.2867307510115102, 2.273907063904318, 2.2622537562270653, 2.2471645887868466, 2.228832288182426, 2.2090979552250873, 2.1830435817613303, 2.1635665646687663, 2.1302079651857735, 2.0920478960885767, 2.042616927939781, 1.9760802393018486, 2.1831421859349507, 2.1830336647272226, 2.1826576229729575, 2.180184456877498, 2.17887995365175, 2.177713367982748, 2.17070482821568, 2.1649401743976786, 2.157490510463643, 2.1522677806504142, 2.136814319502105, 2.128518733679317, 2.114035106865284, 2.0971600975349647, 2.0796416941451303, 2.0600755150567536, 2.0348423236542255, 2.0019675828935743, 1.9679402695348538, 2.0760101295912388, 2.0880779278329378, 2.10071716094914, 2.095322165415623, 2.0939099746666976, 2.0939175677102417, 2.0840508359044243, 2.074789168699424, 2.076618065490292, 2.0714914989147863, 2.0761059125300494, 2.0609213301259333, 2.0494920321920445, 2.0395649531157347, 2.030928141732017, 2.0129827696169316, 1.991172912834405, 1.9816940824139573, 1.9611513314605555]}, {[2.3383503559788656, 2.359270172948628, 2.4048236830520433, 2.459450579041871, 2.511591348338105, 2.55449392287164, 2.5979496262689916, 2.6378890227350245, 2.6729624184416063, 2.7018303550309795, 2.7264793868299213, 2.749676169796435, 2.7684960736541346, 2.7850102267006274, 2.796750984415046, 2.8067764571536102, 2.8132596002773957, 2.8178884541640654, 2.8188839610583316, 2.315887973442095, 2.3346533288434306, 2.375136525197298, 2.4238198263324695, 2.471779264717803, 2.514848566369931, 2.555003951313538, 2.5919002511243088, 2.6257747186158844, 2.653700668896826, 2.6757295847117124, 2.697601649129442, 2.7182867360527414, 2.732479204379476, 2.74471523307909, 2.7533725574405614, 2.7616548966630807, 2.764130363621217, 2.7657590592939294, 2.2900992757661354, 2.3052373411332345, 2.3408120702512694, 2.3863658470930544, 2.4307625657786436, 2.4687541687154013, 2.5062212556052352, 2.541790479530629, 2.5721200886672095, 2.598439369188138, 2.6222284263428426, 2.6427817678884478, 2.659903781761481, 2.6743812861950405, 2.6858800185168428, 2.6941400582634114, 2.700529592833158, 2.7045660651345798, 2.7066081675391604, 2.259235346031739, 2.2708863077094392, 2.30186334529631, 2.3417254197323403, 2.3814274565447313, 2.416271690108693, 2.4506487990414483, 2.484192998500694, 2.512144702967657, 2.536313747021159, 2.558023518859083, 2.5777160943799244, 2.593920022033829, 2.607756027597739, 2.6189430250224723, 2.6270535829437507, 2.6341924724784342, 2.637011577176769, 2.6384940165840556, 2.2202101663833704, 2.228604356200259, 2.253701586209948, 2.288088602880903, 2.3237292296665646, 2.3544433903813884, 2.38588913424697, 2.416157199405339, 2.44208541847349, 2.4640734865814595, 2.483430428747955, 2.5014677538275567, 2.5175482691966784, 2.529842321450986, 2.539231719363952, 2.547169766666745, 2.552894533431566, 2.5564004938563545, 2.5579639991190097, 2.1701290194757528, 2.1752481019937617, 2.1948604897554085, 2.222290377208274, 2.251402504004785, 2.2785020167160894, 2.305941380612529, 2.331940638563486, 2.355791196616135, 2.3749772752480527, 2.392203878331364, 2.40829440101145, 2.4226408161080477, 2.4343636777940874, 2.4422582076255486, 2.4491471702855887, 2.455225474602491, 2.4580452103119077, 2.4595552996241477, 2.1388703075628865, 2.14310994691767, 2.1588467025521054, 2.182750040017008, 2.208820025296224, 2.234098961921123, 2.25739872640121, 2.2813113555610403, 2.302381103829889, 2.3211207830190337, 2.336705235173429, 2.3517208567333325, 2.3637825665278984, 2.3760663951051386, 2.3833188930501366, 2.390259724690552, 2.39516056128754, 2.398243072183643, 2.399198688651199, 2.103106396207975, 2.1055858580074953, 2.1179118773200525, 2.1372275909775755, 2.158688872652917, 2.1788271310352627, 2.199872620246919, 2.222148474330152, 2.240582464543631, 2.2575547029220413, 2.270334086725242, 2.2844236525152906, 2.295734171188186, 2.304734074186056, 2.3129294552874535, 2.319645932508828, 2.3240772720804843, 2.3264876888333275, 2.328934381523818, 2.062672049863547, 2.0603578405384124, 2.068736979722323, 2.079030993167646, 2.096030061752363, 2.1102045261773608, 2.1264836177437183, 2.14560553298252, 2.1600330708935993, 2.1747041296043985, 2.186131659879025, 2.1971209732448242, 2.2080460882958683, 2.2142151042228972, 2.2263180586584856, 2.22888851584425, 2.2345163014586076, 2.2362468566696942, 2.2372400818313447, 2.0081588878691328, 2.0039875824271043, 2.003536094758659, 2.005922505161834, 2.013099244770569, 2.0220456271373544, 2.02944290763973, 2.0401618078465047, 2.050427029760431, 2.0630700092522662, 2.065810154556547, 2.0784776331032386, 2.0860819442264806, 2.0914336463851146, 2.0957559686116736, 2.1017074652566765, 2.1060469717271464, 2.104549297300664, 2.1139565471797277, 1.9575788692332172, 1.9638754448679856, 1.9718851848727175, 1.9657952573738438, 1.9656095922632972, 1.9684471598944637, 1.964530710649968, 1.9630488586900885, 1.9737393912563916, 1.9787210752237252, 1.9950392155024053, 1.9926978447339572, 1.9955596231884831, 2.0001865052800407, 2.0080080426725826, 2.0054975528492105, 2.0000078973718614, 2.0175964547338414, 2.021975623143927], [2.9316284744959002, 2.929881477805574, 2.925725022302699, 2.9177220756629936, 2.907652979284234, 2.894239919140341, 2.877505922398795, 2.8563540026666883, 2.8322389597734614, 2.8051956731962187, 2.7747012472666093, 2.737754462805601, 2.695038473355379, 2.647896167071862, 2.5972697210789715, 2.5451810967499253, 2.4833141088915944, 2.4293442883413543, 2.4047536835037193, 2.874359544318961, 2.874416718219366, 2.870070938333403, 2.861745975235094, 2.849872128855767, 2.8407023272977865, 2.823445301860041, 2.802007481893269, 2.7795390318909603, 2.7541545449172755, 2.723575023138117, 2.6882208511098544, 2.6502011926536486, 2.6042743447956163, 2.5607784404159464, 2.5085053460411464, 2.4535044878158234, 2.404696502200616, 2.3850742592889547, 2.8120202846450195, 2.8110647501828767, 2.8070707374121655, 2.8002834462357233, 2.789430669439989, 2.7791719495193767, 2.7627114786855547, 2.743433676694533, 2.722277554090869, 2.697184461313889, 2.6702787510211685, 2.6366281689017925, 2.5985140216684437, 2.5563365634294906, 2.5157277834205085, 2.4675550084744655, 2.4168745382417525, 2.3754795919178893, 2.360396685958241, 2.741182649950543, 2.7407401618922655, 2.737515162621723, 2.730616052691592, 2.719946611996146, 2.7104369685913996, 2.6948099367453247, 2.677392775417205, 2.6554016487178655, 2.6324570264792277, 2.6077087089170816, 2.575955939444447, 2.5416134066039042, 2.502892906162658, 2.46598641663544, 2.42164156858856, 2.3773936133675067, 2.3418766992389477, 2.3296455946375976, 2.6578836922781353, 2.6566140989136295, 2.652693686630853, 2.646540167561207, 2.6377331025544257, 2.6284150669358177, 2.614653392837992, 2.5984478179293506, 2.5787888873502567, 2.557654563521384, 2.5345096975866337, 2.5063743788185424, 2.4747007316821454, 2.4401875997107205, 2.4064660035973326, 2.367631305722317, 2.3294278068141314, 2.299499484950037, 2.2900290779522594, 2.555615633882789, 2.553933483698276, 2.550899449511171, 2.5445722334409013, 2.5381504130275676, 2.5282010087853983, 2.516047600813006, 2.5009302356624836, 2.484481164372988, 2.465345448092808, 2.4448336972957656, 2.4200098586485472, 2.3922233075293238, 2.3621283582934387, 2.3334807173521246, 2.3006666252684655, 2.2697560352357065, 2.2478443043679976, 2.2415854888313325, 2.492740016189521, 2.49231986086783, 2.4887143147054815, 2.48324334784336, 2.475365224081277, 2.46743201986396, 2.4565234278259576, 2.4428068912367107, 2.4267895055529904, 2.410361598342655, 2.391249079129392, 2.368706391590628, 2.3430220401927895, 2.3170506850911354, 2.2906883720483218, 2.262051065297515, 2.2347724676556395, 2.216155162445313, 2.2115758068653273, 2.4184506588112717, 2.4177188174051123, 2.4148584235364052, 2.4098137791561305, 2.4021899140704828, 2.395061064659339, 2.384310999004003, 2.3734655585315605, 2.3588524311755443, 2.3444593128731412, 2.3263376321193308, 2.3070234980919864, 2.284908680003452, 2.260756790777089, 2.239596052733616, 2.2160846035695516, 2.1942160777261446, 2.180015672264116, 2.1785288618302885, 2.325466714993374, 2.322340734523727, 2.322815193205472, 2.3155822498434677, 2.3114415975864318, 2.30385545672464, 2.2942966064052577, 2.2861110610925035, 2.272761082213082, 2.2610336823042854, 2.246443793577867, 2.229558447477903, 2.2127115999283027, 2.191902457259438, 2.1801952510387896, 2.1607837959550262, 2.147426327908158, 2.1389030046037796, 2.138911282081512, 2.1976404350378567, 2.194951906209354, 2.192027371675612, 2.1871525078010197, 2.1837401331474653, 2.1809144764269583, 2.1722597936161585, 2.165147490497374, 2.156802815974306, 2.1512481057232393, 2.1361673035829787, 2.129298936929126, 2.117873159767733, 2.106163491841994, 2.0962651165977686, 2.0891387266941703, 2.0837032208741397, 2.078691897124856, 2.08608552058544, 2.0993450708002266, 2.108185972339381, 2.1172539074645957, 2.107417189341355, 2.1021547889051, 2.0990573928252814, 2.0859254402479026, 2.0738583707786344, 2.073445342099694, 2.0669094436170874, 2.070834197701101, 2.0566333134353028, 2.0480645848067485, 2.0431501331204016, 2.0425933159008554, 2.0360097778954516, 2.0297592737895616, 2.044171797128649, 2.050467714919871]}]
  out "E1', E2' map coloured by angle set":cluster{dbl[], dbl[]}[](graph)=[{[1.960391667, 1.96395, 1.964858333, 1.964783333, 1.965066667, 1.966358333, 1.967341667, 1.970533333, 1.975933333, 1.981208333, 1.986991667, 1.9887, 1.993983333, 1.998525, 2.003366667, 2.007291667, 2.010375, 2.016083333, 2.018775], [2.103616667, 2.109066667, 2.109416667, 2.105108333, 2.0985, 2.092875, 2.0864, 2.0802, 2.075791667, 2.070616667, 2.065508333, 2.05615, 2.051216667, 2.046983333, 2.04455, 2.042183333, 2.040566667, 2.041175, 2.041491667]}, {[2.003158333, 2.0046, 2.007483333, 2.011925, 2.017033333, 2.023633333, 2.031341667, 2.039791667, 2.048641667, 2.058325, 2.065033333, 2.074866667, 2.0833, 2.091008333, 2.097208333, 2.102025, 2.106216667, 2.108983333, 2.111291667], [2.196025, 2.1949, 2.19305, 2.190366667, 2.185541667, 2.181208333, 2.173725, 2.164375, 2.154508333, 2.145875, 2.134325, 2.124766667, 2.11475, 2.105883333, 2.099075, 2.092341667, 2.087325, 2.083725, 2.081883333]}, {[2.060208333, 2.064741667, 2.072175, 2.081791667, 2.095133333, 2.108266667, 2.1245, 2.142166667, 2.157833333, 2.172066667, 2.185325, 2.197891667, 2.208575, 2.217716667, 2.226233333, 2.229908333, 2.234983333, 2.235541667, 2.236725], [2.323666667, 2.323491667, 2.322275, 2.317708333, 2.312816667, 2.3057, 2.296391667, 2.285258333, 2.271758333, 2.258241667, 2.243808333, 2.226825, 2.208425, 2.191175, 2.177658333, 2.162958333, 2.152308333, 2.143033333, 2.137716667]}, {[2.105091667, 2.111791667, 2.121716667, 2.136008333, 2.154291667, 2.173241667, 2.19535, 2.218758333, 2.2397, 2.256583333, 2.269983333, 2.284675833, 2.2971475, 2.306991667, 2.31468, 2.320805833, 2.324709167, 2.326833333, 2.327125], [2.41685, 2.417708333, 2.415258333, 2.41095, 2.404283333, 2.396708333, 2.38685, 2.374166667, 2.359416667, 2.343625, 2.323891667, 2.303116667, 2.279125, 2.25485, 2.234733333, 2.214875, 2.1991, 2.187875, 2.180358333]}, {[2.143483333, 2.150208333, 2.161633333, 2.179216667, 2.202183333, 2.225733333, 2.251916667, 2.27894, 2.30210675, 2.321888333, 2.337666667, 2.353325, 2.365825, 2.377158333, 2.384858333, 2.390858333, 2.395575, 2.398058333, 2.397933333], [2.4913675, 2.491859167, 2.48918, 2.4840725, 2.477223333, 2.469213333, 2.458326667, 2.445091667, 2.428025, 2.410883333, 2.390291667, 2.365016667, 2.336533333, 2.30825, 2.282841667, 2.258141667, 2.238508333, 2.225533333, 2.217008333]}, {[2.1775, 2.183025, 2.196016667, 2.216541667, 2.243858333, 2.270291667, 2.299676, 2.329216667, 2.355975, 2.376091667, 2.393766667, 2.410083333, 2.424366667, 2.435758333, 2.443616667, 2.450191667, 2.455341667, 2.457883333, 2.4582], [2.55425, 2.553541667, 2.551325, 2.545416667, 2.538966667, 2.53025, 2.518325, 2.503135833, 2.486316667, 2.466695, 2.444466667, 2.41635, 2.385666667, 2.352891667, 2.323591667, 2.294933333, 2.272216667, 2.257616667, 2.24995]}, {[2.232116667, 2.237608333, 2.252575, 2.280024167, 2.3128225, 2.345008333, 2.379466667, 2.413575, 2.442833333, 2.466116667, 2.48555, 2.503733333, 2.519275, 2.53135, 2.54055, 2.548033333, 2.553266667, 2.555883333, 2.556633333], [2.6561, 2.656033333, 2.653025, 2.6479, 2.6395, 2.630575, 2.617266667, 2.601025, 2.581183333, 2.559808333, 2.534183333, 2.502759167, 2.4664025, 2.428383333, 2.393575, 2.357791667, 2.328641667, 2.31185, 2.30585]}, {[2.274035, 2.2802375, 2.299259333, 2.332033333, 2.369858333, 2.406766667, 2.444191667, 2.481825, 2.51305, 2.53835, 2.560558333, 2.579975, 2.596066667, 2.609508333, 2.619975, 2.627683333, 2.63435, 2.636566667, 2.637225], [2.73945, 2.740158333, 2.737916667, 2.731575, 2.721716667, 2.712475, 2.697358333, 2.680066667, 2.658041667, 2.635133333, 2.608125, 2.573008333, 2.533166667, 2.490545, 2.451891667, 2.409791667, 2.374775, 2.354208333, 2.349541667]}, {[2.307579167, 2.314378333, 2.337491667, 2.375958333, 2.418925, 2.4591, 2.499458333, 2.539283333, 2.573725, 2.600716667, 2.624725, 2.6453, 2.661966667, 2.67585, 2.686825, 2.694791667, 2.700691667, 2.704191667, 2.705316667], [2.810258333, 2.8105, 2.807475, 2.801341667, 2.7911, 2.781116667, 2.765166667, 2.746433333, 2.724641667, 2.699766667, 2.671158333, 2.633491667, 2.590441667, 2.544425, 2.501685, 2.45417, 2.412591667, 2.3881, 2.383508333]}, {[2.334358333, 2.3435, 2.371475, 2.414241667, 2.460875, 2.50545, 2.548441667, 2.589525, 2.626741667, 2.655541667, 2.678608333, 2.700075, 2.72025, 2.733825, 2.745575, 2.754075, 2.761891667, 2.763625, 2.764575], [2.872791667, 2.873891667, 2.870325, 2.862483333, 2.8512, 2.8425, 2.825866667, 2.804941667, 2.78255, 2.757241667, 2.724783333, 2.685333333, 2.642233333, 2.592433333, 2.546675, 2.494478333, 2.447691667, 2.417191667, 2.41095]}, {[2.357966667, 2.367716667, 2.400833333, 2.449375, 2.501233333, 2.545475, 2.591691667, 2.635783333, 2.674008333, 2.703908333, 2.729233333, 2.752258333, 2.77055, 2.786458333, 2.796925, 2.807291667, 2.813483333, 2.817483333, 2.817816667], [2.929983333, 2.929458333, 2.92605, 2.918566667, 2.908825, 2.896141667, 2.879666667, 2.859191667, 2.835225, 2.808475, 2.775591667, 2.734741667, 2.686808333, 2.635733333, 2.585316667, 2.530825, 2.476695, 2.441908333, 2.433175]}]
  out "Probe angles traversed in each angle set\n1st index: angle (deg)\n2nd index: angle set":dbl[][](array[numeric])=[[-45.0, -45.0, -45.0, -45.0, -45.0, -45.0, -45.0, -45.0, -45.0, -45.0, -45.0], [-40.23, -40.23, -40.23, -40.23, -40.23, -40.23, -40.23, -40.23, -40.14, -40.14, -40.14], [-35.1, -35.1, -35.1, -35.1, -35.1, -35.1, -35.1, -35.1, -35.1, -35.1, -35.1], [-29.88, -29.88, -29.88, -29.88, -29.88, -29.88, -29.88, -29.88, -29.88, -29.97, -29.88], [-24.75, -24.75, -24.75, -24.75, -24.75, -25.02, -24.75, -24.75, -24.75, -24.84, -24.84], [-20.25, -20.25, -20.25, -20.25, -19.98, -20.25, -20.25, -20.25, -20.25, -20.25, -20.25], [-15.21, -15.21, -15.21, -15.21, -15.21, -15.21, -15.21, -15.21, -15.21, -15.21, -15.21], [-9.99, -9.99, -9.99, -9.99, -9.99, -9.99, -9.99, -9.99, -9.99, -9.99, -9.99], [-4.86, -4.86, -4.86, -4.86, -4.86, -4.86, -4.86, -4.86, -5.04, -4.86, -4.86], [0.0, 0.0, 0.0, 0.0, 0.0, 0.0, 0.0, 0.0, -0.09, 0.0, 0.0], [4.77, 4.77, 4.77, 4.77, 4.77, 4.77, 4.77, 4.77, 4.77, 4.77, 4.77], [9.9, 9.9, 9.9, 9.9, 9.9, 9.9, 9.9, 9.99, 9.9, 9.9, 9.9], [15.12, 15.12, 15.03, 15.03, 15.03, 15.12, 15.12, 15.03, 15.03, 15.03, 15.03], [19.98, 20.16, 20.25, 20.16, 20.16, 20.25, 20.16, 20.16, 20.16, 20.16, 20.16], [24.84, 24.84, 24.75, 24.75, 24.75, 24.75, 24.75, 24.75, 24.75, 24.75, 25.02], [29.79, 29.79, 29.79, 29.79, 29.79, 29.79, 29.79, 29.79, 29.7, 29.7, 29.7], [35.01, 35.01, 35.01, 35.01, 35.01, 35.01, 34.92, 35.01, 34.92, 34.92, 34.92], [40.14, 40.14, 40.14, 40.14, 40.14, 39.96, 40.14, 40.14, 40.14, 40.14, 40.14], [45.0, 45.0, 45.0, 45.0, 45.0, 45.0, 45.0, 45.0, 45.0, 45.0, 45.0]]
  out "Uref associated with each angle set (m/s)":dbl[](array[numeric])=[0.5018157894736842, 0.9994315789473684, 2.000205263157895, 3.000784210526316, 3.999947368421053, 4.999831578947369, 6.999731578947368, 9.001931578947369, 10.999973684210525, 13.000168421052631, 15.001142105263158] format="%#.2f"
  out "Effective angle X plot":cluster{dbl[], dbl[]}[](graph)=[{[-0.9999999999999999, -0.8459634362504808, -0.7028117712403573, -0.5745611109571804, -0.46100631442731815, -0.3689194771098271, -0.2718814121476857, -0.17614702688068878, -0.08502702101131297, 0.0, 0.0834450784477064, 0.17452793889436508, 0.26851046270375567, 0.3689194771098271, 0.46100631442731815, 0.5724736448682121, 0.7004676747806673, 0.8432720672116305, 0.9999999999999999], [0.30634432922847776, 0.33124816021705167, 0.35386539609822504, 0.3408985513360128, 0.31933956286322085, 0.27992690365585854, 0.2229566711987844, 0.1648204978101121, 0.09048095699602061, 0.024587958833567094, -0.05583002015618459, -0.14536657156999755, -0.22976404784875964, -0.3439588090465734, -0.4078131503047583, -0.524419756113169, -0.6469848704640956, -0.7801983209141452, -0.9404179116719943]}, {[-0.9999999999999999, -0.8459634362504808, -0.7028117712403573, -0.5745611109571804, -0.46100631442731815, -0.3689194771098271, -0.2718814121476857, -0.17614702688068878, -0.08502702101131297, 0.0, 0.0834450784477064, 0.17452793889436508, 0.26851046270375567, 0.3689194771098271, 0.46100631442731815, 0.5724736448682121, 0.7004676747806673, 0.8432720672116305, 0.9999999999999999], [-0.9263298161188739, -0.7979083840543126, -0.6410572155338587, -0.5349167839293223, -0.41844373376018384, -0.3330488687483389, -0.2428262977232454, -0.1367476713685922, -0.05472559253622773, 0.027981322188340485, 0.0957331804870974, 0.16696015985501583, 0.24137984761334605, 0.2888506647729097, 0.3456317153666766, 0.3692623500583355, 0.38245375617740995, 0.37674525575952256, 0.35009108307473]}, {[-0.9999999999999999, -0.8459634362504808, -0.7028117712403573, -0.5745611109571804, -0.46100631442731815, -0.3689194771098271, -0.2718814121476857, -0.17614702688068878, -0.08502702101131297, 0.0, 0.0834450784477064, 0.17452793889436508, 0.26851046270375567, 0.3689194771098271, 0.46100631442731815, 0.5724736448682121, 0.7004676747806673, 0.8432720672116305, 0.9999999999999999], [0.8490646106157206, 0.718316555449873, 0.5968077309329735, 0.48794705527528537, 0.3915604023947652, 0.31339600692555414, 0.23102895093559755, 0.14976847367312107, 0.07242473615963936, 0.00025279617886625743, -0.07057637226415707, -0.14788858030398422, -0.2276620568639879, -0.31289041456782163, -0.3910548100370327, -0.48566959703900026, -0.5943124418060763, -0.7155264972549548, -0.848559018257988]}, {[-0.9999999999999999, -0.8459634362504808, -0.7028117712403573, -0.5745611109571804, -0.46100631442731815, -0.3689194771098271, -0.2718814121476857, -0.17614702688068878, -0.08502702101131297, 0.0, 0.0834450784477064, 0.17452793889436508, 0.26851046270375567, 0.3689194771098271, 0.46100631442731815, 0.5724736448682121, 0.7004676747806673, 0.8432720672116305, 0.9999999999999999], [-0.8562957498298522, -0.7233812051257119, -0.5998589847170553, -0.48919449243934415, -0.3912107169489937, -0.3117511408758629, -0.22801926638152503, -0.14541230657563686, -0.06678698672456035, 0.006580839135572939, 0.07858364379248216, 0.15717691172790887, 0.23827223129491767, 0.3249128191470088, 0.40437239522013957, 0.50055494509206, 0.610997997030858, 0.7342205640609676, 0.8694574281009981]}]
  out "Wire angle error with speed":cluster{dbl[], dbl[]}[](graph)=[{[0.5018157894736842, 0.9994315789473684, 2.000205263157895, 3.000784210526316, 3.999947368421053, 4.999831578947369, 6.999731578947368, 9.001931578947369, 10.999973684210525, 13.000168421052631, 15.001142105263158], [9.301789072480183, -0.5078267063761874, -0.017067028732528303, 0.5397928552976248, 0.5552032611501811, 0.5839145398374913, 0.47699542926605193, 0.29554643025088057, 0.07088419516207646, -0.22434555500855446, -0.46685131819457854]}, {[0.5018157894736842, 0.9994315789473684, 2.000205263157895, 3.000784210526316, 3.999947368421053, 4.999831578947369, 6.999731578947368, 9.001931578947369, 10.999973684210525, 13.000168421052631, 15.001142105263158], [-6.2576200383800815, 0.4756008610831978, 0.43891338578357947, -0.1673075851488837, -0.48092962089557495, -0.4879117310338565, -0.3766339827294708, -0.1481957767585597, 0.2586334095830275, 0.5043620030432825, 0.7171710888419789]}]
  out "Effective angle variation with speed":cluster{dbl[], dbl[]}[](graph)=[{[0.5018157894736842, 0.9994315789473684, 2.000205263157895, 3.000784210526316, 3.999947368421053, 4.999831578947369, 6.999731578947368, 9.001931578947369, 10.999973684210525, 13.000168421052631, 15.001142105263158], [-30.285464661725992, -33.254964934057156, -40.31507047722743, -41.74714774284409, -42.36499226518007, -42.51768679264624, -42.64039509148493, -42.6422862340712, -42.49979129772667, -42.32144635887174, -42.13803507246683]}, {[0.5018157894736842, 0.9994315789473684, 2.000205263157895, 3.000784210526316, 3.999947368421053, 4.999831578947369, 6.999731578947368, 9.001931578947369, 10.999973684210525, 13.000168421052631, 15.001142105263158], [38.49074431439611, 37.20280767808152, 40.53842758348162, 42.73363765516822, 43.49048567985748, 43.685527244188464, 43.83997004830012, 43.67153411038288, 43.25329915480998, 42.91487849910852, 42.74976368597849]}]
  out "Probe zero alignment error":cluster{dbl[], dbl[]}(graph)={[0.5018157894736842, 0.9994315789473684, 2.000205263157895, 3.000784210526316, 3.999947368421053, 4.999831578947369, 6.999731578947368, 9.001931578947369, 10.999973684210525, 13.000168421052631, 15.001142105263158], [1.5220845170500508, -0.016112922646494804, 0.21092317852552558, 0.18624263507437055, 0.0371368201273031, 0.04800140440181741, 0.05018072326829057, 0.07367532674616044, 0.16475880237255197, 0.140008224017364, 0.12515988532370018]}
  out "Zero angle calibration coeffs. (King's 1914 law)":T1={"A1"=2.895294801714706, "B1"=1.359762188126494, "n1"=0.4357683216387929, "A2"=3.2944413738572145, "B2"=1.3280301230872396, "n2"=0.4590330236259289}
  in  "No. of pts. about zero angle to make up linear least squares fit (for std. method)":i32=4
  in  "Query set":i32=3
  out "Pts per set":i32=19
  out "Angle sets":i32=11
  # "This vi allows you to inspect the finer details of your angle calibration. You can check the extent of validity of the effective angle method. The probe zero angle alignment error is given graphically, you can then correct the recorded angles in the calibration file by ADDING the value obtained from the graph where the curve has levelled off (which typically occurs at speed > 4m/s. Similarly the effective angle typically becomes constant at speed > 4m/s)."
  # "of"
  # "Paul Nathan 23/02/10"
  # "HIGHER ORDER METHOD\nBELOW"
  # "HIGHER ORDER METHOD\nBELOW"
  # "HIGHER ORDER METHOD\nBELOW"
  # "0. Actual data\n1. Standard effective angle method\n2. Higher order effective angle method\n    with tangential cooling factor"
  # "ADVANCED DIAGNOSTICS: This section reveals the guts of the quartic equation for epsilon and whether the algorithm fell back to the lower order method. You can check all the roots for each angle set and see the effects of constraining the polynomial coefficients (in particular setting the zero order coeff to zero). Since the constraint affects the master plots, be sure to empty the coefficient constraint array when finished."
  # "The numerical data for all the standard effective angle method plots is available for copying and pasting into Excel below"
  # "The numerical data for all the higher order effective angle method plots is available for copying and pasting into Excel below"
  # "The numerical data for the E1, E2 plane maps (actual data, and synthesis from both effective angle methods) is available for copying and pasting into Excel below"
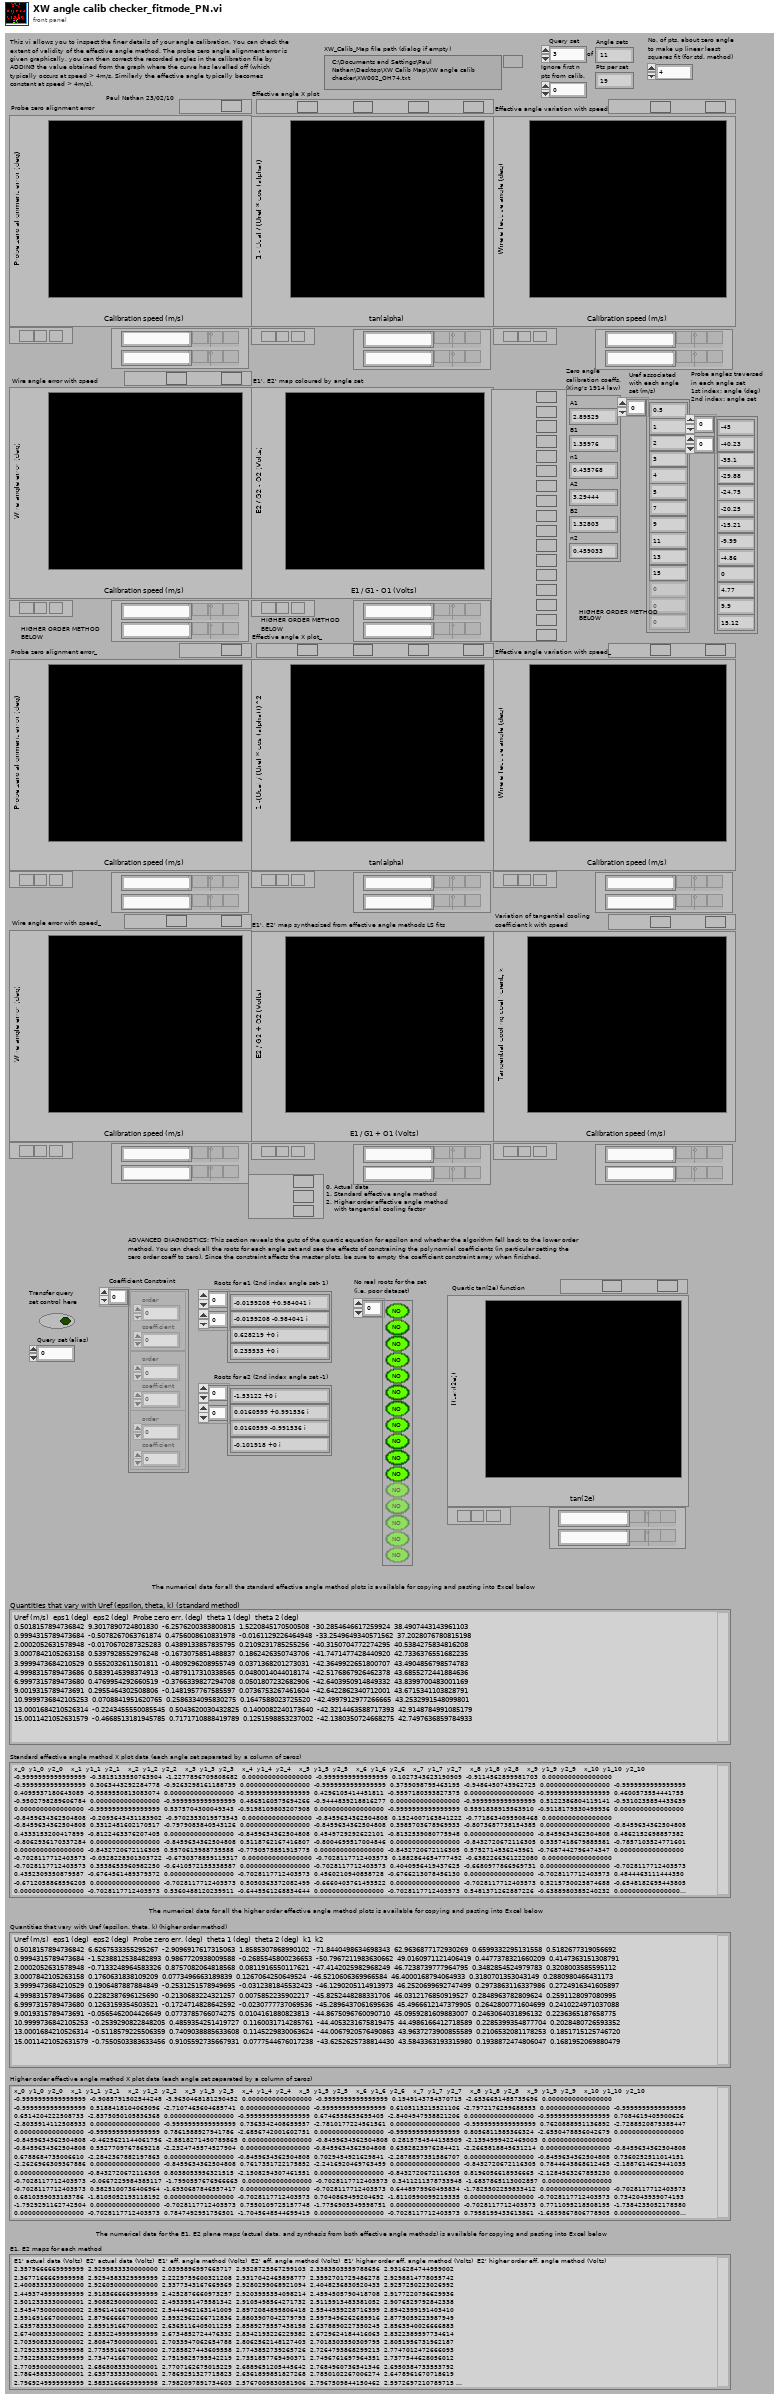
[diagram p1: front panel]
types:
  T1 = cluster{"A1":dbl, "B1":dbl, "n1":dbl, "A2":dbl, "B2":dbl, "n2":dbl}
  T2 = cluster{"A":dbl, "B":dbl, "n":dbl, "A":dbl, "B":dbl, "n":dbl}
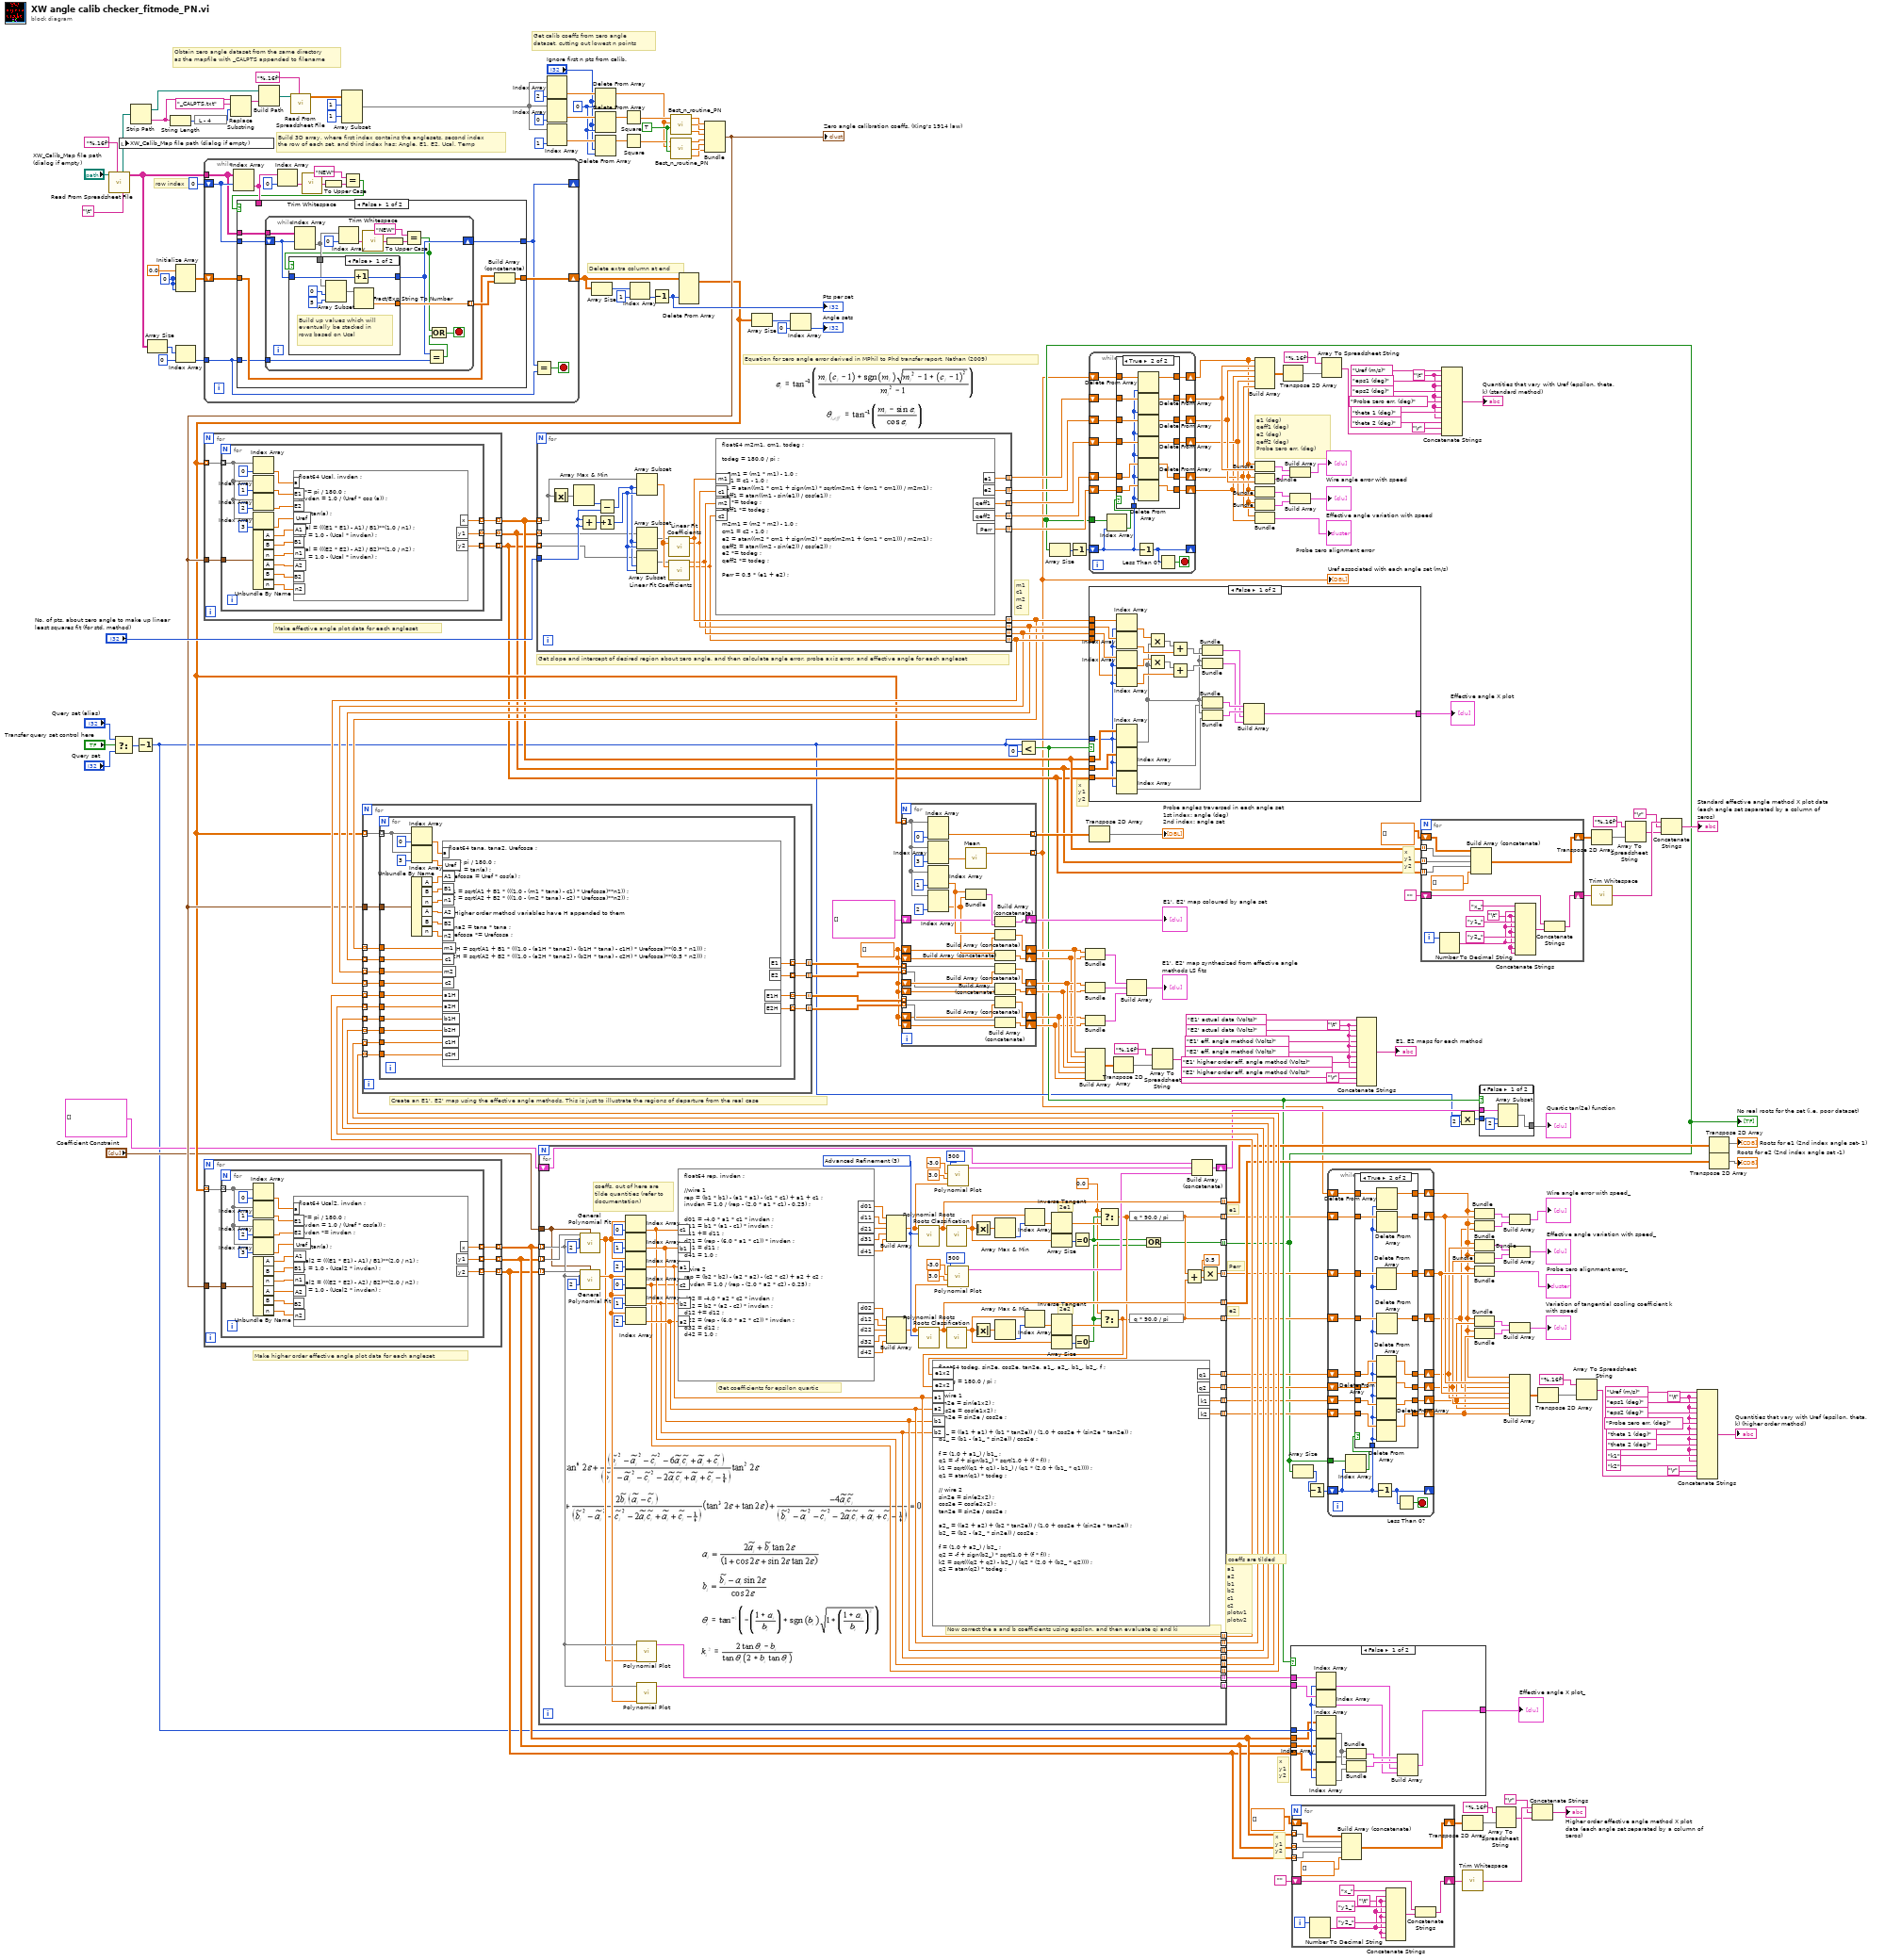
[diagram p0: block diagram]
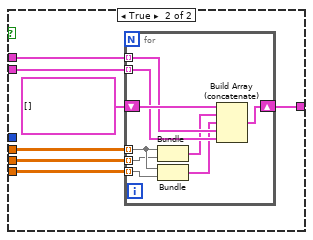
[diagram p5: hidden frame]
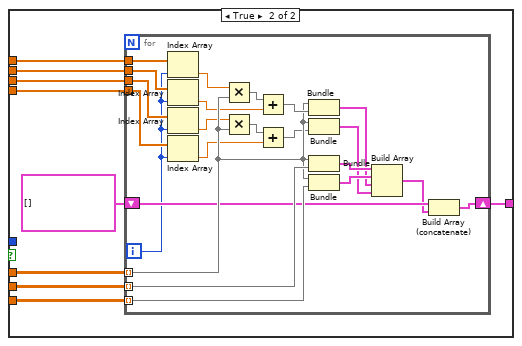
[diagram p6: hidden frame]
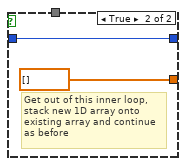
[diagram p7: hidden frame]
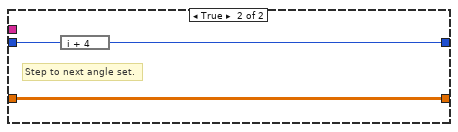
[diagram p8: hidden frame]
diagram:
  w54 = 0 ("index")
  w62 = "\t"
  w108 = "\t"
  w121 = "\t"
  w58 = dbl[] []
  w188 = TRUE ("variable n?")
  w205 = 0 ("dimension size")
  # "x\ny1\ny2"
  # "x\ny1\ny2"
  # "x\ny1\ny2"
  # "coeffs are tilded"
  # "a1\na2\nb1\nb2\nc1\nc2\nplotw1\nplotw2"
  # "Make higher order effective angle plot data for each angleset"
  # "e2"
  # "e1"
  # "Perr"
  # "Create an E1', E2' map using the effective angle methods. This is just to illustrate the regions of departure from the real case"
  # "Equation for zero angle error derived in MPhil to Phd transfer report, Nathan (2009)"
  # "x\ny1\ny2"
  # "m1\nc1\nm2\nc2"
  # "e1 (deg)\nqeff1 (deg)\ne2 (deg)\nqeff2 (deg)\nProbe zero err. (deg)"
  # "Get slope and intercept of desired region about zero angle, and then calculate angle error, probe axis error, and effective angle for each angleset"
  # "Make effective angle plot data for each angleset"
  # "Get calib coeffs from zero angle dataset, cutting out lowest n points"
  # "Obtain zero angle dataset from the same directory as the mapfile with _CALPTS appended to filename"
  # "Delete extra column at end"
  # "Build 3D array, where first index contains the anglesets, second index the row of each set, and third index has: Angle, E1, E2, Ucal, Temp"
  # "row index"
  n1 = call-poly <vilib>:"Read From Spreadsheet File.vi"("delimiter (\\t)"="\t", "format (%s)"="%.16f" ("format (%.3f)"), "file path (dialog if empty)"="XW_Calib_Map file path (dialog if empty)") -> ("all rows"=w219:string[][], "new file path (Not A Path if cancelled)"=w191:path)  [unwired: 2 in, 5 out]
  n2 = Select(t="Query set (alias)", s="Transfer query set control here", f="Query set") -> (s? t:f=w37:i32)
  n3 = local write "XW_Calib_Map file path (dialog if empty)"(w191) -> ()
  n4 = Strip Path(path=w191) -> (stripped path=w198:path, name=w202:string)
  n5 = Decrement(x=w37) -> (x-1=w35:i32)
  n6 = Array Size(array=w219) -> (size(s)=w216:i32[])
  n7 = String Length(string=w202) -> (length=w201:i32)
  n8 = Initialize Array(0.0 ("element"), w205, w205, w205) -> (w204:dbl[][][])
  n9 = Index Array(array=w216, index=0) -> (element=w215:i32)
  n10 = expression code="L - 4"(w201) -> (w200:i32)
  n11 = while {
    tunnel: w219 -> [w228]
    shift-right: [w226] -> w209
    shift-left: w204 -> [w227]
    shift-right: [w225] -> _
    shift-left: 0 ("index") -> [w231]
    tunnel: w215 -> [w224]
    stop <- w233 stop-if-true
    n12 = Index Array(array=w228, index (row)=w231) -> (element=w230:string[])  [unwired: 1 in]
    n13 = Index Array(array=w230, index=0) -> (element=w223:string)
    n14 = call <vilib>:"Trim Whitespace.vi"("string"=w223) -> ("trimmed string"=w222:string)  [unwired: 1 in]
    n15 = To Upper Case(1:w222) -> (0:w235:string)
    n16 = Equal?(x="NEW", y=w235) -> (x = y?=w229:bool)
    n17 = case shown="False" w229 {
      tunnel: w231 -> [w242 w268]
      tunnel: [w237 w266] -> w225
      tunnel: w230 -> [_ _]
      tunnel: w228 -> [w241 _]
      tunnel: w227 -> [w238 w267]
      tunnel: [w240 w267] -> w226
      tunnel: w224 -> [w236 _]
      frame False {
        n18 = while {
          tunnel: w241 -> [w252]
          shift-right: [w247] -> w237
          shift-left: w242 -> [w250]
          tunnel: [w251] -> w239 mode=indexing
          tunnel: w236 -> [w249]
          stop <- w246 stop-if-true
          n19 = Index Array(array=w252, index (row)=w250) -> (element=w253:string[])  [unwired: 1 in]
          n20 = Index Array(array=w253, index=0) -> (element=w244:string)
          n21 = call <vilib>:"Trim Whitespace.vi"("string"=w244) -> ("trimmed string"=w243:string)  [unwired: 1 in]
          n22 = To Upper Case(1:w243) -> (0:w256:string)
          n23 = Equal?(x="NEW", y=w256) -> (x = y?=w245:bool)
          n24 = case shown="False" w245 {
            tunnel: w253 -> [w258 _]
            tunnel: [w257 dbl[] []] -> w251
            tunnel: w250 -> [w261 w265]
            tunnel: [w260 w265] -> w247
            frame False {
              # "Build up values which will eventually be stacked in rows based on Ucal"
              n25 = Array Subset(array=w258, index=0, length=5) -> (w262:string[])
              n26 = Increment(x=w261) -> (x+1=w260:i32)
              n27 = Fract/Exp String To Number(string=w262) -> (number=w257:dbl[])  [unwired: 4 out]
            }
            frame True {
              # "Get out of this inner loop, stack new 1D array onto existing array and continue as before"
            }
          }
          n28 = Equal?(x=w247, y=w249) -> (x = y?=w248:bool)
          n29 = Or(x=w245, y=w248) -> (x .or. y?=w246:bool)
        }
        n30 = Build Array (concatenate)(w238, w239) -> (w240:dbl[][][])
      }
      frame True {
        # "Step to next angle set."
        n31 = expression code="i + 4"(w268) -> (w266:i32)
      }
    }
    n32 = Equal?(x=w225, y=w224) -> (x = y?=w233:bool)
  }
  n33 = Replace Substring(3:w200, 4:"_CALPTS.txt" ("substring (\"\")"), 5:w202) -> (1:w197:string)  [unwired: 2 out]
  n34 = Build Path(base path=w198, name or relative path=w197) -> (appended path=w192:path)
  n35 = call-poly <vilib>:"Read From Spreadsheet File.vi"("format (%.3f)"="%.16f", "file path (dialog if empty)"=w192) -> ("all rows"=w194:dbl[][])  [unwired: 2 in, 7 out]
  n36 = Array Subset(array=w194, index (row)=1 ("index"), index (col)=1 ("index")) -> (w189:dbl[][])  [unwired: 2 in]
  n37 = Index Array(array=w189, index (col)=2 ("index")) -> (element=w57:dbl[])  [unwired: 1 in]
  n38 = Index Array(array=w189, index (col)=0 ("index")) -> (element=w56:dbl[])  [unwired: 1 in]
  n39 = Index Array(array=w189, index (col)=1 ("index")) -> (element=w55:dbl[])  [unwired: 1 in]
  n40 = Array Size(array=w209) -> (size(s)=w211:i32[])
  n41 = Delete From Array(array=w57, length="Ignore first n pts from calib.", index=w54) -> (array with subset deleted=w53:dbl[])  [unwired: 1 out]
  n42 = Delete From Array(array=w56, length="Ignore first n pts from calib.", index=w54) -> (array with subset deleted=w52:dbl[])  [unwired: 1 out]
  n43 = Delete From Array(array=w55, length="Ignore first n pts from calib.", index=w54) -> (array with subset deleted=w51:dbl[])  [unwired: 1 out]
  n44 = Square(x=w52) -> (x^2=w177:dbl[])
  n45 = Square(x=w51) -> (x^2=w176:dbl[])
  n46 = Index Array(array=w211, index=1) -> (element=w210:i32)
  n47 = Decrement(x=w210) -> (x-1=w207:i32)
  "Pts per set" <- w207
  n48 = call "Best_n_routine_PN.vi"("variable n?"=w188, "U"=w53, "E^2"=w177) -> ("n"=w183:dbl, "B"=w184:dbl, "A"=w185:dbl)  [unwired: 1 in]
  n49 = call "Best_n_routine_PN.vi"("variable n?"=w188, "U"=w53, "E^2"=w176) -> ("n"=w180:dbl, "B"=w181:dbl, "A"=w182:dbl)  [unwired: 1 in]
  n50 = Delete From Array(array=w209, index (dim 1)=w207) -> (array with subset deleted=w153:dbl[][][])  [unwired: 3 in, 1 out]
  n51 = Bundle("A"=w185, "B"=w184, "n"=w183, "A"=w182, "B"=w181, "n"=w180) -> (w154:T2)  [unwired: 1 out]
  "Zero angle calibration coeffs. (King's 1914 law)" <- w154
  n52 = for {
    tunnel: w153 -> [w273] mode=indexing
    tunnel: w154 -> [w272]
    tunnel: [w271] -> w97 mode=indexing
    tunnel: [w270] -> w96 mode=indexing
    tunnel: [w269] -> w95 mode=indexing
    n53 = for {
      tunnel: w273 -> [w278] mode=indexing
      tunnel: w272 -> [w291]
      tunnel: [w276] -> w271 mode=indexing
      tunnel: [w275] -> w270 mode=indexing
      tunnel: [w274] -> w269 mode=indexing
      n54 = Index Array(array=w278, index=0) -> (element=w290:dbl)
      n55 = Index Array(array=w278, index=1) -> (element=w279:dbl)
      n56 = Index Array(array=w278, index=2) -> (element=w277:dbl)
      n57 = Index Array(array=w278, index=3) -> (element=w280:dbl)
      n58 = Unbundle By Name(w291) -> ("A"=w289:dbl, "B"=w288:dbl, "n"=w287:dbl, "A"=w286:dbl, "B"=w285:dbl, "n"=w284:dbl)
      n59 = formula code="float64 Ucal, invden ;\n\na *= pi / 180.0 ;\ninvden = 1.0 / (Uref * cos (a)) ;\n\nx = tan(a) ;\n\nUcal = (((E1 * E1) - A1) / B1)**(1.0 / n1) ;\ny1 = 1.0 - (Ucal * invden) ;\n\nUcal = (((E2 * E2) - A2) / B2)**(1.0 / n2) ;\ny2 = 1.0 - (Ucal * invden) ;"("A1"=w289, "B1"=w288, "n1"=w287, "A2"=w286, "B2"=w285, "n2"=w284, "E1"=w279, "E2"=w277, "a"=w290, "Uref"=w280) -> ("x"=w276:dbl, "y1"=w275:dbl, "y2"=w274:dbl)
    }
  }
  n60 = for {
    tunnel: w153 -> [w297] mode=indexing
    tunnel: w154 -> [w296]
    tunnel: [w295] -> w75 mode=indexing
    tunnel: [w294] -> w74 mode=indexing
    tunnel: [w293] -> w73 mode=indexing
    n61 = for {
      tunnel: w297 -> [w302] mode=indexing
      tunnel: w296 -> [w315]
      tunnel: [w300] -> w295 mode=indexing
      tunnel: [w299] -> w294 mode=indexing
      tunnel: [w298] -> w293 mode=indexing
      n62 = Index Array(array=w302, index=0) -> (element=w314:dbl)
      n63 = Index Array(array=w302, index=1) -> (element=w303:dbl)
      n64 = Index Array(array=w302, index=2) -> (element=w301:dbl)
      n65 = Index Array(array=w302, index=3) -> (element=w304:dbl)
      n66 = Unbundle By Name(w315) -> ("A"=w313:dbl, "B"=w312:dbl, "n"=w311:dbl, "A"=w310:dbl, "B"=w309:dbl, "n"=w308:dbl)
      n67 = formula code="float64 Ucal2, invden ;\n\na *= pi / 180.0 ;\ninvden = 1.0 / (Uref * cos(a)) ;\ninvden *= invden ;\n\nx = tan(a) ;\n\nUcal2 = (((E1 * E1) - A1) / B1)**(2.0 / n1) ;\ny1 = 1.0 - (Ucal2 * invden) ;\n\nUcal2 = (((E2 * E2) - A2) / B2)**(2.0 / n2) ;\ny2 = 1.0 - (Ucal2 * invden) ;"("A1"=w313, "B1"=w312, "n1"=w311, "A2"=w310, "B2"=w309, "n2"=w308, "E1"=w303, "E2"=w301, "a"=w314, "Uref"=w304) -> ("x"=w300:dbl, "y1"=w299:dbl, "y2"=w298:dbl)
    }
  }
  n68 = for {
    tunnel: w97 -> [w336] mode=indexing
    tunnel: w96 -> [w330] mode=indexing
    tunnel: w95 -> [w329] mode=indexing
    tunnel: "No. of pts. about zero angle to make up linear least squares fit (for std. method)" -> [w334]
    tunnel: [w325] -> w9 mode=indexing
    tunnel: [w324] -> w11 mode=indexing
    tunnel: [w323] -> w10 mode=indexing
    tunnel: [w322] -> w12 mode=indexing
    tunnel: [w321] -> w13 mode=indexing
    tunnel: [w320] -> w161 mode=indexing
    tunnel: [w319] -> w162 mode=indexing
    tunnel: [w318] -> w163 mode=indexing
    tunnel: [w317] -> w164 mode=indexing
    n69 = Absolute Value(x=w336) -> (abs(x)=w337:dbl[])
    n70 = Array Max & Min(array=w337) -> (min index (indices)=w335:i32)  [unwired: 3 out]
    n71 = Add(x=w334, y=w334) -> (x+y=w333:i32)
    n72 = Subtract(x=w335, y=w334) -> (x-y=w331:i32)
    n73 = Increment(x=w333) -> (x+1=w332:i32)
    n74 = Array Subset(array=w336, index=w331, length=w332) -> (w328:dbl[])
    n75 = Array Subset(array=w330, index=w331, length=w332) -> (w327:dbl[])
    n76 = Array Subset(array=w329, index=w331, length=w332) -> (w326:dbl[])
    n77 = call <vilib>:"Linear Fit Coefficients.vi"("Y"=w327, "X"=w328) -> ("slope"=w320:dbl, "intercept"=w319:dbl)  [unwired: 3 in, 9 out]
    n78 = call <vilib>:"Linear Fit Coefficients.vi"("Y"=w326, "X"=w328) -> ("slope"=w318:dbl, "intercept"=w317:dbl)  [unwired: 3 in, 9 out]
    n79 = formula code="float64 m2m1, cm1, todeg ;\n\ntodeg = 180.0 / pi ;\n\nm2m1 = (m1 * m1) - 1.0 ;\ncm1 = c1 - 1.0 ;\ne1 = atan((m1 * cm1 + sign(m1) * sqrt(m2m1 + (cm1 * cm1))) / m2m1) ;\nqeff1 = atan((m1 - sin(e1)) / cos(e1)) ;\ne1 *= todeg ;\nqeff1 *= todeg ;\n\nm2m1 = (m2 * m2) - 1.0 ;\ncm1 = c2 - 1.0 ;\ne2 = atan((m2 * cm1 + sign(m2) * sqrt(m2m1 + (cm1 * cm1))) / m2m1) ;\nqeff2 = atan((m2 - sin(e2)) / cos(e2)) ;\ne2 *= todeg ;\nqeff2 *= todeg ;\n\nPerr = 0.5 * (e1 + e2) ;"("m1"=w320, "c1"=w319, "m2"=w318, "c2"=w317) -> ("e1"=w325:dbl, "qeff1"=w324:dbl, "Perr"=w321:dbl, "e2"=w323:dbl, "qeff2"=w322:dbl)
  }
  n80 = for {
    tunnel: w75 -> [w381] mode=indexing
    tunnel: w74 -> [w410] mode=indexing
    tunnel: w73 -> [w402] mode=indexing
    tunnel: [w382] -> w32 mode=indexing
    tunnel: [w380] -> w33 mode=indexing
    tunnel: [w379] -> w31 mode=indexing
    tunnel: [w378] -> w30 mode=indexing
    tunnel: [w377] -> w29 mode=indexing
    tunnel: [w376] -> w28 mode=indexing
    tunnel: [w375] -> w27 mode=indexing
    tunnel: [w374] -> w132 mode=indexing
    tunnel: [w373] -> w131 mode=indexing
    tunnel: [w372] -> w152 mode=indexing
    tunnel: [w371] -> w151 mode=indexing
    tunnel: [w370] -> w150 mode=indexing
    tunnel: [w369] -> w149 mode=indexing
    tunnel: [w368] -> w148 mode=indexing
    tunnel: [w367] -> w147 mode=indexing
    tunnel: "Coefficient Constraint" -> [w360]
    tunnel: [w359] -> w48 mode=indexing
    shift-right: [w351] -> w43
    shift-left: cluster{dbl[], dbl[]}[] [] -> [w354]
    tunnel: [w350] -> w45 mode=indexing
    tunnel: [w344] -> w8 mode=indexing
    w343 = 0.0 ("end")
    w391 = u16 3 items=["General", "Simple Classification", "Refinement", "Advanced Refinement"] ("option")
    # "Now correct the a and b coefficients using epsilon, and then evaluate qi and ki"
    # "2e2"
    # "2e1"
    # "coeffs. out of here are tilde quantities (refer to documentation)"
    # "Get coefficients for epsilon quartic"
    n81 = call <vilib>:"General Polynomial Fit.vi"("Y"=w410, "polynomial order"=2, "Coefficient Constraint"=w360, "X"=w381) -> ("Polynomial Coefficients"=w365:dbl[])  [unwired: 8 in, 3 out]
    n82 = call <vilib>:"General Polynomial Fit.vi"("Y"=w402, "polynomial order"=2, "Coefficient Constraint"=w360, "X"=w381) -> ("Polynomial Coefficients"=w366:dbl[])  [unwired: 8 in, 3 out]
    n83 = Index Array(array=w365, index=0) -> (element=w368:dbl)
    n84 = Index Array(array=w365, index=1) -> (element=w370:dbl)
    n85 = Index Array(array=w365, index=2) -> (element=w372:dbl)
    n86 = Index Array(array=w366, index=0) -> (element=w367:dbl)
    n87 = Index Array(array=w366, index=1) -> (element=w369:dbl)
    n88 = Index Array(array=w366, index=2) -> (element=w371:dbl)
    n89 = call-poly <vilib>:"Polynomial Plot.vi"("P(x)"=w365, "X"=w381) -> ("polynomial plot"=w374:cluster{dbl[], "P(A)":dbl[]})  [unwired: 9 out]
    n90 = call-poly <vilib>:"Polynomial Plot.vi"("P(x)"=w366, "X"=w381) -> ("polynomial plot"=w373:cluster{dbl[], "P(A)":dbl[]})  [unwired: 9 out]
    n91 = formula code="float64 rep, invden ;\n\n//wire 1\nrep = (b1 * b1) - (a1 * a1) - (c1 * c1) + a1 + c1 ;\ninvden = 1.0 / (rep - (2.0 * a1 * c1) - 0.25) ;\n\nd01 = -4.0 * a1 * c1 * invden ;\nd11 = b1 * (a1 - c1) * invden ; \nd11 += d11 ;\nd21 = (rep - (6.0 * a1 * c1)) * invden ;\nd31 = d11 ;\nd41 = 1.0 ;\n\n//wire 2\nrep = (b2 * b2) - (a2 * a2) - (c2 * c2) + a2 + c2 ;\ninvden = 1.0 / (rep - (2.0 * a2 * c2) - 0.25) ;\n\nd02 = -4.0 * a2 * c2 * invden ;\nd12 = b2 * (a2 - c2) * invden ;\nd12 += d12 ;\nd22 = (rep - (6.0 * a2 * c2)) * invden ;\nd32 = d12 ;\nd42 = 1.0 ;"("c1"=w368, "a1"=w372, "b1"=w370, "c2"=w367, "b2"=w369, "a2"=w371) -> ("d01"=w401:dbl, "d11"=w400:dbl, "d21"=w399:dbl, "d02"=w394:dbl, "d12"=w395:dbl, "d22"=w396:dbl, "d31"=w398:dbl, "d41"=w397:dbl, "d32"=w393:dbl, "d42"=w392:dbl)
    n92 = Build Array(w401, w400, w399, w398, w397) -> (w364:dbl[])
    n93 = Build Array(w394, w395, w396, w393, w392) -> (w355:dbl[])
    n94 = call-poly <vilib>:"Polynomial Roots.vi"("option"=w391, "P(x)"=w364) -> ("Roots"=w359:cdb[])  [unwired: 9 out]
    n95 = call-poly <vilib>:"Polynomial Roots.vi"("option"=w391, "P(x)"=w355) -> ("Roots"=w350:cdb[])  [unwired: 9 out]
    n96 = call <vilib>:"Roots Classification.vi"("Roots"=w359) -> ("Real Roots"=w341:dbl[])  [unwired: 2 in, 8 out]
    n97 = call <vilib>:"Roots Classification.vi"("Roots"=w350) -> ("Real Roots"=w338:dbl[])  [unwired: 2 in, 8 out]
    n98 = call-poly <vilib>:"Polynomial Plot.vi"("P(x)"=w364, "end"=3.0, "start"=-3.0, "samples"=500) -> ("polynomial plot"=w353:cluster{"Ramp Pattern":dbl[], "P(A)":dbl[]})  [unwired: 7 out]
    n99 = call-poly <vilib>:"Polynomial Plot.vi"("P(x)"=w355, "end"=3.0, "start"=-3.0, "samples"=500) -> ("polynomial plot"=w352:cluster{"Ramp Pattern":dbl[], "P(A)":dbl[]})  [unwired: 7 out]
    n100 = Absolute Value(x=w341) -> (abs(x)=w390:dbl[])
    n101 = Absolute Value(x=w338) -> (abs(x)=w387:dbl[])
    n102 = Array Max & Min(array=w390) -> (min index (indices)=w389:i32)  [unwired: 3 out]
    n103 = Array Max & Min(array=w387) -> (min index (indices)=w388:i32)  [unwired: 3 out]
    n104 = Index Array(array=w341, index=w389) -> (element=w386:dbl)
    n105 = Index Array(array=w338, index=w388) -> (element=w385:dbl)
    n106 = Inverse Tangent(1:w386) -> (0:w349:dbl)
    n107 = Array Size(array=w341) -> (size(s)=w342:i32)
    n108 = Inverse Tangent(1:w385) -> (0:w347:dbl)
    n109 = Array Size(array=w338) -> (size(s)=w340:i32)
    n110 = Equal To 0?(x=w342) -> (x = 0?=w345:bool)
    n111 = Equal To 0?(x=w340) -> (x = 0?=w339:bool)
    n112 = Select(t=w343, s=w345, f=w349) -> (s? t:f=w348:dbl)
    n113 = Select(t=w343, s=w339, f=w347) -> (s? t:f=w346:dbl)
    n114 = formula code="float64 todeg, sin2e, cos2e, tan2e, a1_, a2_, b1_, b2_, f ;\n\ntodeg = 180.0 / pi ;\n\n// wire 1\nsin2e = sin(e1x2) ; \ncos2e = cos(e1x2) ; \ntan2e = sin2e / cos2e ;\n\na1_ = ((a1 + a1) + (b1 * tan2e)) / (1.0 + cos2e + (sin2e * tan2e)) ;\nb1_ = (b1 - (a1_ * sin2e)) / cos2e ;\n\nf = (1.0 + a1_) / b1_ ;\nq1 = -f + sign(b1_) * sqrt(1.0 + (f * f)) ;\nk1 = sqrt(((q1 + q1) - b1_) / (q1 * (2.0 + (b1_ * q1)))) ;\nq1 = atan(q1) * todeg ;\n\n// wire 2\nsin2e = sin(e2x2) ; \ncos2e = cos(e2x2) ; \ntan2e = sin2e / cos2e ;\n\na2_ = ((a2 + a2) + (b2 * tan2e)) / (1.0 + cos2e + (sin2e * tan2e)) ;\nb2_ = (b2 - (a2_ * sin2e)) / cos2e ;\n\nf = (1.0 + a2_) / b2_ ;\nq2 = -f + sign(b2_) * sqrt(1.0 + (f * f)) ;\nk2 = sqrt(((q2 + q2) - b2_) / (q2 * (2.0 + (b2_ * q2)))) ;\nq2 = atan(q2) * todeg ;"("e1x2"=w348, "e2x2"=w346, "a1"=w372, "a2"=w371, "b1"=w370, "b2"=w369) -> ("q1"=w378:dbl, "q2"=w377:dbl, "k1"=w376:dbl, "k2"=w375:dbl)
    n115 = expression code="q * 90.0 / pi"(w348) -> (w380:dbl)
    n116 = expression code="q * 90.0 / pi"(w346) -> (w379:dbl)
    n117 = Or(x=w345, y=w339) -> (x .or. y?=w344:bool)
    n118 = Add(x=w380, y=w379) -> (x+y=w383:dbl)
    n119 = Build Array (concatenate)(w354, w353, w352) -> (w351:cluster{"Ramp Pattern":dbl[], "P(A)":dbl[]}[])
    n120 = Multiply(x=0.5, y=w383) -> (x*y=w382:dbl)
  }
  "No real roots for the set (i.e. poor dataset)" <- w8
  n121 = for {
    tunnel: w153 -> [w427] mode=indexing
    tunnel: w154 -> [w426]
    tunnel: [w425] -> w159 mode=indexing
    tunnel: [w424] -> w160 mode=indexing
    tunnel: w164 -> [w423] mode=indexing
    tunnel: w163 -> [w422] mode=indexing
    tunnel: w162 -> [w421] mode=indexing
    tunnel: w161 -> [w420] mode=indexing
    tunnel: w152 -> [w419] mode=indexing
    tunnel: w151 -> [w418] mode=indexing
    tunnel: w150 -> [w417] mode=indexing
    tunnel: w149 -> [w416] mode=indexing
    tunnel: w148 -> [w415] mode=indexing
    tunnel: w147 -> [w414] mode=indexing
    tunnel: [w413] -> w136 mode=indexing
    tunnel: [w412] -> w135 mode=indexing
    n122 = for {
      tunnel: w427 -> [w442] mode=indexing
      tunnel: w426 -> [w452]
      tunnel: [w441] -> w425 mode=indexing
      tunnel: [w440] -> w424 mode=indexing
      tunnel: w423 -> [w439]
      tunnel: w422 -> [w438]
      tunnel: w421 -> [w437]
      tunnel: w420 -> [w436]
      tunnel: w419 -> [w435]
      tunnel: w418 -> [w434]
      tunnel: w417 -> [w433]
      tunnel: w416 -> [w432]
      tunnel: w415 -> [w431]
      tunnel: w414 -> [w430]
      tunnel: [w429] -> w413 mode=indexing
      tunnel: [w428] -> w412 mode=indexing
      n123 = Index Array(array=w442, index=0) -> (element=w451:dbl)
      n124 = Index Array(array=w442, index=3) -> (element=w443:dbl)
      n125 = Unbundle By Name(w452) -> ("A"=w450:dbl, "B"=w449:dbl, "n"=w448:dbl, "A"=w447:dbl, "B"=w446:dbl, "n"=w445:dbl)
      n126 = formula code="float64 tana, tana2, Urefcosa ;\n\na *= pi / 180.0 ;\ntana = tan(a) ;\nUrefcosa = Uref * cos(a) ;\n\nE1 = sqrt(A1 + B1 * (((1.0 - (m1 * tana) - c1) * Urefcosa)**n1)) ;\nE2 = sqrt(A2 + B2 * (((1.0 - (m2 * tana) - c2) * Urefcosa)**n2)) ;\n\n// Higher order method variables have H appended to them\n\ntana2 = tana * tana ;\nUrefcosa *= Urefcosa ;\n\nE1H = sqrt(A1 + B1 * (((1.0 - (a1H * tana2) - (b1H * tana) - c1H) * Urefcosa)**(0.5 * n1))) ;\nE2H = sqrt(A2 + B2 * (((1.0 - (a2H * tana2) - (b2H * tana) - c2H) * Urefcosa)**(0.5 * n2))) ;"("A1"=w450, "B1"=w449, "n1"=w448, "A2"=w447, "B2"=w446, "n2"=w445, "a"=w451, "Uref"=w443, "m1"=w436, "c1"=w437, "m2"=w438, "c2"=w439, "a1H"=w435, "a2H"=w434, "b1H"=w433, "b2H"=w432, "c1H"=w431, "c2H"=w430) -> ("E1"=w441:dbl, "E2"=w440:dbl, "E1H"=w429:dbl, "E2H"=w428:dbl)
    }
  }
  n127 = Array Size(array=w153) -> (size(s)=w214:i32[])
  n128 = Index Array(array=w214, index=0) -> (element=→"Angle sets":i32)
  n129 = for {
    shift-right: [w475] -> w167
    shift-left: cluster{dbl[], dbl[]}[] [] -> [w472]
    tunnel: w153 -> [w476] mode=indexing
    tunnel: [w482] -> w166 mode=indexing
    tunnel: [w480] -> w1 mode=indexing
    shift-right: [w471] -> w114
    shift-left: w58 -> [w466]
    tunnel: w160 -> [w467] mode=indexing
    tunnel: w159 -> [w468] mode=indexing
    shift-right: [w469] -> w115
    shift-left: w58 -> [w470]
    shift-right: [w462] -> w98
    shift-left: w58 -> [w465]
    shift-right: [w464] -> w116
    shift-left: w58 -> [w463]
    shift-right: [w454] -> w112
    shift-left: w58 -> [w459]
    tunnel: w135 -> [w458] mode=indexing
    tunnel: w136 -> [w457] mode=indexing
    shift-right: [w456] -> w113
    shift-left: w58 -> [w455]
    n130 = Index Array(array=w476, index (col)=0 ("index")) -> (element=w482:dbl[])  [unwired: 1 in]
    n131 = Index Array(array=w476, index (col)=3 ("index")) -> (element=w481:dbl[])  [unwired: 1 in]
    n132 = Index Array(array=w476, index (col)=1 ("index")) -> (element=w461:dbl[])  [unwired: 1 in]
    n133 = Index Array(array=w476, index (col)=2 ("index")) -> (element=w460:dbl[])  [unwired: 1 in]
    n134 = call <vilib>:"Mean.vi"("X"=w481) -> ("mean"=w480:dbl)  [unwired: 1 out]
    n135 = Bundle(w461, w460) -> (w473:cluster{dbl[], dbl[]})  [unwired: 1 out]
    n136 = Build Array (concatenate)(w472, w473) -> (w475:cluster{dbl[], dbl[]}[])
    n137 = Build Array (concatenate)(w461, w463) -> (w464:dbl[])
    n138 = Build Array (concatenate)(w460, w465) -> (w462:dbl[])
    n139 = Build Array (concatenate)(w468, w470) -> (w469:dbl[])
    n140 = Build Array (concatenate)(w467, w466) -> (w471:dbl[])
    n141 = Build Array (concatenate)(w457, w455) -> (w456:dbl[])
    n142 = Build Array (concatenate)(w458, w459) -> (w454:dbl[])
  }
  "Uref associated with each angle set (m/s)" <- w1
  "E1', E2' map coloured by angle set" <- w167
  n143 = Less?(x=w35, y=0) -> (x < y?=w42:bool)
  n144 = Array Size(array=w8) -> (size(s)=w15:i32)
  n145 = Decrement(x=w15) -> (x-1=w14:i32)
  n146 = Bundle(w116, w98) -> (w157:cluster{dbl[], dbl[]})  [unwired: 1 out]
  n147 = Bundle(w115, w114) -> (w156:cluster{dbl[], dbl[]})  [unwired: 1 out]
  n148 = Bundle(w113, w112) -> (w134:cluster{dbl[], dbl[]})  [unwired: 1 out]
  n149 = Build Array(w116, w98, w115, w114, w113, w112) -> (w111:dbl[][])
  n150 = while {
    shift-right: [w496] -> w7
    shift-left: w9 -> [w499]
    shift-right: [w497] -> w6
    shift-left: w10 -> [w498]
    shift-right: [w494] -> w5
    shift-left: w11 -> [w495]
    shift-right: [w490] -> w4
    shift-left: w12 -> [w493]
    shift-right: [w491] -> w3
    shift-left: w13 -> [w492]
    shift-right: [w488] -> w2
    shift-left: w1 -> [w489]
    shift-right: [w483] -> _
    shift-left: w14 -> [w484]
    tunnel: w8 -> [w487]
    stop <- w486 stop-if-true
    n151 = Index Array(array=w487, index=w484) -> (element=w485:bool)
    n152 = case shown="True" w485 {
      tunnel: [w505 w517] -> w496
      tunnel: w499 -> [w505 w518]
      tunnel: w498 -> [w504 w516]
      tunnel: [w504 w515] -> w497
      tunnel: w495 -> [w503 w514]
      tunnel: [w503 w513] -> w494
      tunnel: w493 -> [w501 w511]
      tunnel: w492 -> [w502 w512]
      tunnel: [w502 w509] -> w491
      tunnel: [w501 w510] -> w490
      tunnel: w489 -> [w500 w508]
      tunnel: [w500 w507] -> w488
      tunnel: w484 -> [_ w506]
      frame False {
      }
      frame True {
        n153 = Delete From Array(array=w508, index=w506) -> (array with subset deleted=w507:dbl[])  [unwired: 1 in, 1 out]
        n154 = Delete From Array(array=w518, index=w506) -> (array with subset deleted=w517:dbl[])  [unwired: 1 in, 1 out]
        n155 = Delete From Array(array=w516, index=w506) -> (array with subset deleted=w515:dbl[])  [unwired: 1 in, 1 out]
        n156 = Delete From Array(array=w514, index=w506) -> (array with subset deleted=w513:dbl[])  [unwired: 1 in, 1 out]
        n157 = Delete From Array(array=w511, index=w506) -> (array with subset deleted=w510:dbl[])  [unwired: 1 in, 1 out]
        n158 = Delete From Array(array=w512, index=w506) -> (array with subset deleted=w509:dbl[])  [unwired: 1 in, 1 out]
      }
    }
    n159 = Decrement(x=w484) -> (x-1=w483:i32)
    n160 = Less Than 0?(x=w483) -> (x < 0?=w486:bool)
  }
  n161 = case shown="False" w42 {
    tunnel: w161 -> [w539 w548]
    tunnel: w162 -> [w538 w547]
    tunnel: w163 -> [w537 w546]
    tunnel: w164 -> [w535 w545]
    tunnel: w97 -> [w542 w551]
    tunnel: w96 -> [w541 w550]
    tunnel: w95 -> [w540 w549]
    tunnel: [w519 w543] -> w168
    tunnel: w35 -> [w536 _]
    frame False {
      n162 = Index Array(array=w539, index=w536) -> (element=w527:dbl)
      n163 = Index Array(array=w538, index=w536) -> (element=w526:dbl)
      n164 = Index Array(array=w537, index=w536) -> (element=w525:dbl)
      n165 = Index Array(array=w535, index=w536) -> (element=w524:dbl)
      n166 = Index Array(array=w542, index (row)=w536) -> (element=w523:dbl[])  [unwired: 1 in]
      n167 = Index Array(array=w541, index (row)=w536) -> (element=w522:dbl[])  [unwired: 1 in]
      n168 = Index Array(array=w540, index (row)=w536) -> (element=w521:dbl[])  [unwired: 1 in]
      n169 = Multiply(x=w527, y=w523) -> (x*y=w532:dbl[])
      n170 = Multiply(x=w525, y=w523) -> (x*y=w530:dbl[])
      n171 = Add(x=w532, y=w526) -> (x+y=w531:dbl[])
      n172 = Add(x=w530, y=w524) -> (x+y=w529:dbl[])
      n173 = Bundle(w523, w531) -> (w528:cluster{dbl[], dbl[]})  [unwired: 1 out]
      n174 = Bundle(w523, w529) -> (w520:cluster{dbl[], dbl[]})  [unwired: 1 out]
      n175 = Bundle(w523, w522) -> (w534:cluster{dbl[], dbl[]})  [unwired: 1 out]
      n176 = Bundle(w523, w521) -> (w533:cluster{dbl[], dbl[]})  [unwired: 1 out]
      n177 = Build Array(w534, w533, w528, w520) -> (w519:cluster{dbl[], dbl[]}[])
    }
    frame True {
      n178 = for {
        tunnel: w551 -> [w567] mode=indexing
        tunnel: w550 -> [w573] mode=indexing
        tunnel: w549 -> [w571] mode=indexing
        tunnel: w548 -> [w560]
        tunnel: w547 -> [w559]
        tunnel: w546 -> [w558]
        tunnel: w545 -> [w557]
        shift-right: [w561] -> w543
        shift-left: cluster{dbl[], dbl[]}[] [] -> [w563]
        i -> [w556]
        n179 = Index Array(array=w560, index=w556) -> (element=w555:dbl)
        n180 = Index Array(array=w559, index=w556) -> (element=w554:dbl)
        n181 = Index Array(array=w558, index=w556) -> (element=w553:dbl)
        n182 = Index Array(array=w557, index=w556) -> (element=w552:dbl)
        n183 = Multiply(x=w555, y=w567) -> (x*y=w570:dbl[])
        n184 = Multiply(x=w553, y=w567) -> (x*y=w568:dbl[])
        n185 = Add(x=w570, y=w554) -> (x+y=w569:dbl[])
        n186 = Add(x=w568, y=w552) -> (x+y=w566:dbl[])
        n187 = Bundle(w567, w569) -> (w565:cluster{dbl[], dbl[]})  [unwired: 1 out]
        n188 = Bundle(w567, w566) -> (w564:cluster{dbl[], dbl[]})  [unwired: 1 out]
        n189 = Bundle(w567, w573) -> (w574:cluster{dbl[], dbl[]})  [unwired: 1 out]
        n190 = Bundle(w567, w571) -> (w572:cluster{dbl[], dbl[]})  [unwired: 1 out]
        n191 = Build Array(w574, w572, w565, w564) -> (w562:cluster{dbl[], dbl[]}[])
        n192 = Build Array (concatenate)(w563, w562) -> (w561:cluster{dbl[], dbl[]}[])
      }
    }
  }
  "Effective angle X plot" <- w168
  n193 = Transpose 2D Array(2D array=w166) -> (transposed array=→"Probe angles traversed in each angle set\n1st index: angle (deg)\n2nd index: angle set":dbl[][])
  n194 = Transpose 2D Array(2D array=w111) -> (transposed array=w109:dbl[][])
  n195 = Build Array(w157, w156, w134) -> (→"E1', E2' map synthesized from effective angle methods LS fits":cluster{dbl[], dbl[]}[])
  n196 = Array To Spreadsheet String(array=w109, 3:"%.16f" ("format string")) -> (spreadsheet string=w100:string)  [unwired: 1 out]
  n197 = Build Array(w2, w7, w6, w3, w5, w4) -> (w71:dbl[][])
  n198 = Bundle(w2, w7) -> (w172:cluster{dbl[], dbl[]})  [unwired: 1 out]
  n199 = Bundle(w2, w6) -> (w173:cluster{dbl[], dbl[]})  [unwired: 1 out]
  n200 = Bundle(w2, w5) -> (w175:cluster{dbl[], dbl[]})  [unwired: 1 out]
  n201 = Bundle(w2, w4) -> (w174:cluster{dbl[], dbl[]})  [unwired: 1 out]
  n202 = Bundle(w2, w3) -> (→"Probe zero alignment error":cluster{dbl[], dbl[]})  [unwired: 1 out]
  n203 = Transpose 2D Array(2D array=w71) -> (transposed array=w70:dbl[][])
  n204 = Build Array(w172, w173) -> (→"Wire angle error with speed":cluster{dbl[], dbl[]}[])
  n205 = Build Array(w175, w174) -> (→"Effective angle variation with speed":cluster{dbl[], dbl[]}[])
  n206 = case shown="False" w42 {
    tunnel: w132 -> [w588 w595]
    tunnel: w131 -> [w587 w592]
    tunnel: [w577 w593] -> w133
    tunnel: w35 -> [w586 _]
    tunnel: w75 -> [w585 w589]
    tunnel: w74 -> [w584 w590]
    tunnel: w73 -> [w583 w591]
    frame False {
      n207 = Index Array(array=w588, index=w586) -> (element=w575:cluster{dbl[], "P(A)":dbl[]})
      n208 = Index Array(array=w587, index=w586) -> (element=w576:cluster{dbl[], "P(A)":dbl[]})
      n209 = Index Array(array=w585, index (row)=w586) -> (element=w580:dbl[])  [unwired: 1 in]
      n210 = Index Array(array=w584, index (row)=w586) -> (element=w579:dbl[])  [unwired: 1 in]
      n211 = Index Array(array=w583, index (row)=w586) -> (element=w578:dbl[])  [unwired: 1 in]
      n212 = Bundle(w580, w579) -> (w581:cluster{dbl[], dbl[]})  [unwired: 1 out]
      n213 = Bundle(w580, w578) -> (w582:cluster{dbl[], dbl[]})  [unwired: 1 out]
      n214 = Build Array(w581, w582, w575, w576) -> (w577:cluster{dbl[], "P(A)":dbl[]}[])
    }
    frame True {
      n215 = for {
        tunnel: w595 -> [w601] mode=indexing
        tunnel: w592 -> [w602] mode=indexing
        shift-right: [w604] -> w593
        shift-left: cluster{dbl[], dbl[]}[] [] -> [w603]
        tunnel: w591 -> [w598] mode=indexing
        tunnel: w590 -> [w599] mode=indexing
        tunnel: w589 -> [w600] mode=indexing
        n216 = Bundle(w600, w599) -> (w597:cluster{dbl[], dbl[]})  [unwired: 1 out]
        n217 = Bundle(w600, w598) -> (w596:cluster{dbl[], dbl[]})  [unwired: 1 out]
        n218 = Build Array (concatenate)(w603, w597, w596, w601, w602) -> (w604:cluster{dbl[], "P(A)":dbl[]}[])
      }
    }
  }
  "Effective angle X plot_" <- w133
  n219 = for {
    tunnel: w75 -> [w610] mode=indexing
    tunnel: w74 -> [w609] mode=indexing
    tunnel: w73 -> [w608] mode=indexing
    shift-right: [w613] -> w79
    shift-left: "" -> [w612]
    shift-right: [w606] -> w80
    shift-left: dbl[][] [] -> [w605]
    i -> [w619]
    w614 = "\t"
    n220 = Number To Decimal String(number=w619) -> (decimal integer string=w615:string)  [unwired: 1 out]
    n221 = Build Array (concatenate)(w605, w610, w609, w608, dbl[] [] ("element")) -> (w606:dbl[][])
    n222 = Concatenate Strings("x_" ("format string"), w615, w614, "y1_" ("format string"), w615, w614, "y2_" ("format string"), w615, w614, w614) -> (w611:string)
    n223 = Concatenate Strings(w612, w611) -> (w613:string)
  }
  n224 = Array Size(array=w8) -> (size(s)=w18:i32)
  n225 = Decrement(x=w18) -> (x-1=w19:i32)
  n226 = Array To Spreadsheet String(array=w70, 3:"%.16f" ("format string")) -> (spreadsheet string=w60:string)  [unwired: 1 out]
  n227 = while {
    shift-right: [w637] -> w25
    shift-left: w33 -> [w640]
    shift-right: [w638] -> w26
    shift-left: w32 -> [w639]
    shift-right: [w635] -> w17
    shift-left: w31 -> [w636]
    shift-right: [w627] -> w24
    shift-left: w30 -> [w634]
    shift-right: [w628] -> w23
    shift-left: w29 -> [w633]
    shift-right: [w629] -> w22
    shift-left: w28 -> [w632]
    shift-right: [w630] -> w21
    shift-left: w27 -> [w631]
    shift-right: [w625] -> w20
    shift-left: w1 -> [w626]
    shift-right: [w620] -> _
    shift-left: w19 -> [w621]
    tunnel: w8 -> [w624]
    stop <- w623 stop-if-true
    n228 = Index Array(array=w624, index=w621) -> (element=w622:bool)
    n229 = case shown="True" w622 {
      tunnel: [w648 w664] -> w637
      tunnel: w640 -> [w648 w665]
      tunnel: w639 -> [w647 w663]
      tunnel: [w647 w662] -> w638
      tunnel: w636 -> [w646 w661]
      tunnel: [w646 w660] -> w635
      tunnel: w634 -> [w642 w655]
      tunnel: w633 -> [w643 w656]
      tunnel: w632 -> [w644 w657]
      tunnel: w631 -> [w645 w659]
      tunnel: [w645 w658] -> w630
      tunnel: [w644 w652] -> w629
      tunnel: [w643 w653] -> w628
      tunnel: [w642 w654] -> w627
      tunnel: w626 -> [w641 w651]
      tunnel: [w641 w650] -> w625
      tunnel: w621 -> [_ w649]
      frame False {
      }
      frame True {
        n230 = Delete From Array(array=w663, index=w649) -> (array with subset deleted=w662:dbl[])  [unwired: 1 in, 1 out]
        n231 = Delete From Array(array=w655, index=w649) -> (array with subset deleted=w654:dbl[])  [unwired: 1 in, 1 out]
        n232 = Delete From Array(array=w656, index=w649) -> (array with subset deleted=w653:dbl[])  [unwired: 1 in, 1 out]
        n233 = Delete From Array(array=w657, index=w649) -> (array with subset deleted=w652:dbl[])  [unwired: 1 in, 1 out]
        n234 = Delete From Array(array=w659, index=w649) -> (array with subset deleted=w658:dbl[])  [unwired: 1 in, 1 out]
        n235 = Delete From Array(array=w651, index=w649) -> (array with subset deleted=w650:dbl[])  [unwired: 1 in, 1 out]
        n236 = Delete From Array(array=w665, index=w649) -> (array with subset deleted=w664:dbl[])  [unwired: 1 in, 1 out]
        n237 = Delete From Array(array=w661, index=w649) -> (array with subset deleted=w660:dbl[])  [unwired: 1 in, 1 out]
      }
    }
    n238 = Decrement(x=w621) -> (x-1=w620:i32)
    n239 = Less Than 0?(x=w620) -> (x < 0?=w623:bool)
  }
  n240 = Concatenate Strings("E1' actual data (Volts)", w108, "E2' actual data (Volts)", w108, "E1' eff. angle method (Volts)", w108, "E2' eff. angle method (Volts)", w108, "E1' higher order eff. angle method (Volts)", w108, "E2' higher order eff. angle method (Volts)", "\r", w100) -> (→"E1, E2 maps for each method":string)
  n241 = for {
    tunnel: w97 -> [w671] mode=indexing
    tunnel: w96 -> [w670] mode=indexing
    tunnel: w95 -> [w669] mode=indexing
    shift-right: [w674] -> w89
    shift-left: "" -> [w673]
    shift-right: [w667] -> w90
    shift-left: dbl[][] [] -> [w666]
    i -> [w680]
    w675 = "\t"
    n242 = Number To Decimal String(number=w680) -> (decimal integer string=w676:string)  [unwired: 1 out]
    n243 = Build Array (concatenate)(w666, w671, w670, w669, dbl[] [] ("element")) -> (w667:dbl[][])
    n244 = Concatenate Strings("x_" ("format string"), w676, w675, "y1_" ("format string"), w676, w675, "y2_" ("format string"), w676, w675, w675) -> (w672:string)
    n245 = Concatenate Strings(w673, w672) -> (w674:string)
  }
  n246 = Concatenate Strings("Uref (m/s)", w62, "eps1 (deg)", w62, "eps2 (deg)", w62, "Probe zero err. (deg)", w62, "theta 1 (deg)", w62, "theta 2 (deg)", "\r", w60) -> (→"Quantities that vary with Uref (epsilon, theta, k) (standard method)":string)
  n247 = Multiply(x=w35, y=2) -> (x*y=w34:i32)
  n248 = Transpose 2D Array(2D array=w80) -> (transposed array=w82:dbl[][])
  n249 = call <vilib>:"Trim Whitespace.vi"("string"=w79) -> ("trimmed string"=w78:string)  [unwired: 1 in]
  n250 = Bundle(w20, w25) -> (w144:cluster{dbl[], dbl[]})  [unwired: 1 out]
  n251 = Bundle(w20, w17) -> (w143:cluster{dbl[], dbl[]})  [unwired: 1 out]
  n252 = Bundle(w20, w24) -> (w141:cluster{dbl[], dbl[]})  [unwired: 1 out]
  n253 = Bundle(w20, w23) -> (w142:cluster{dbl[], dbl[]})  [unwired: 1 out]
  n254 = Bundle(w20, w26) -> (→"Probe zero alignment error_":cluster{dbl[], dbl[]})  [unwired: 1 out]
  n255 = Bundle(w20, w22) -> (w139:cluster{dbl[], dbl[]})  [unwired: 1 out]
  n256 = Bundle(w20, w21) -> (w138:cluster{dbl[], dbl[]})  [unwired: 1 out]
  n257 = case shown="False" w42 {
    tunnel: w43 -> [w684 w685]
    tunnel: w34 -> [w683 _]
    tunnel: [w681 w685] -> w41
    frame False {
      n258 = Array Subset(array=w684, index=w683, length=2) -> (w681:cluster{dbl[], dbl[]}[])
    }
    frame True {
    }
  }
  "Quartic tan(2e) function" <- w41
  n259 = Array To Spreadsheet String(array=w82, 3:"%.16f" ("format string")) -> (spreadsheet string=w76:string)  [unwired: 1 out]
  n260 = Build Array(w144, w143) -> (→"Wire angle error with speed_":cluster{dbl[], dbl[]}[])
  n261 = Build Array(w141, w142) -> (→"Effective angle variation with speed_":cluster{dbl[], dbl[]}[])
  n262 = Build Array(w139, w138) -> (→"Variation of tangential cooling coefficient k with speed":cluster{dbl[], dbl[]}[])
  n263 = Build Array(w20, w25, w17, w26, w24, w23, w22, w21) -> (w130:dbl[][])
  n264 = Concatenate Strings(w78, "\r", w76) -> (→"Higher order effective angle method X plot data (each angle set separated by a column of zeros)":string)
  n265 = Transpose 2D Array(2D array=w130) -> (transposed array=w16:dbl[][])
  n266 = Array To Spreadsheet String(array=w16, 3:"%.16f" ("format string")) -> (spreadsheet string=w118:string)  [unwired: 1 out]
  n267 = Transpose 2D Array(2D array=w90) -> (transposed array=w92:dbl[][])
  n268 = call <vilib>:"Trim Whitespace.vi"("string"=w89) -> ("trimmed string"=w88:string)  [unwired: 1 in]
  n269 = Array To Spreadsheet String(array=w92, 3:"%.16f" ("format string")) -> (spreadsheet string=w85:string)  [unwired: 1 out]
  n270 = Concatenate Strings(w88, "\r", w85) -> (→"Standard effective angle method X plot data (each angle set separated by a column of zeros)":string)
  n271 = Concatenate Strings("Uref (m/s)", w121, "eps1 (deg)", w121, "eps2 (deg)", w121, "Probe zero err. (deg)", w121, "theta 1 (deg)", w121, "theta 2 (deg)", w121, "k1", w121, "k2", "\r", w118) -> (→"Quantities that vary with Uref (epsilon, theta, k) (higher order method)":string)
  n272 = Transpose 2D Array(2D array=w48) -> (transposed array=→"Roots for e1 (2nd index angle set- 1)":cdb[][])
  n273 = Transpose 2D Array(2D array=w45) -> (transposed array=→"Roots for e2 (2nd index angle set -1)":cdb[][])
